vi "fly dominator105.vi"() -> ()   [LabVIEW 2021]
uses:
  states.ctl
  <vilib>/Analysis/NI_AALBase.lvlib
  <vilib>/Analysis/baseanly.llb/Mean (DBL).vi
  <extravilib>/ChannelInstances/Tag-bool.lvlib
  <vilib>/DAQmx/write.llb/DAQmx Write (Digital Bool 1Line 1Point).vi
  <vilib>/DAQmx/create/channels.llb/DAQmx Create Channel (DO-Digital Output).vi
  <resource>/objmgr/daqmx.rc
  <extravilib>/ChannelInstances/Tag-dbl.lvlib
  <vilib>/Waveform/WDTFileIO.llb/ Write Waveform to File.vi
  C:/Users/IMAGINGPC-3/Desktop/software/4c wheel/Thorlabs.MotionControl.Controls.dll
  software/4c wheel/Thorlabs.MotionControl.Controls.dll
  C:/Users/IMAGINGPC-3/Desktop/software/4c wheel/Thorlabs.MotionControl.Benchtop.StepperMotorCLI.dll
  software/4c wheel/Thorlabs.MotionControl.Benchtop.StepperMotorCLI.dll
  <vilib>/Analysis/NI_AALPro.lvlib
  0273469b-1630-426e-8888-91f9d245564e.vi
  8ea25fb4-7a89-4be8-837a-9bc05b844755.vi
  <vilib>/smtpClient/LabVIEWSMTPClient.lvlib
  a9b58a78-20d6-47fd-9184-b30837673e93.vi
  <vilib>/smtpClient/Set Message Text.vi
  <vilib>/DAQmx/create/channels.llb/DAQmx Create Channel (AI-Voltage-Basic).vi
  <vilib>/DAQmx/configure/timing.llb/DAQmx Timing (Sample Clock).vi
  <vilib>/DAQmx/read.llb/DAQmx Read (Analog 1D DBL 1Chan NSamp).vi
  <vilib>/DAQmx/read.llb/DAQmx Read (Digital Bool 1Line 1Point).vi
  <vilib>/DAQmx/create/channels.llb/DAQmx Create Channel (DI-Digital Input).vi
  <vilib>/Instr/_visa.llb/VISA Configure Serial Port (Instr).vi
panel:
  in  "fast scan setting":enum32{"4000", "2000"}(tab)
  out "Last saved file 4000":path
  in  "Save base file name 4000":path=path "\\\\157.82.9.50\\d/20240220/gp mor/tm6b/4000/uasmcherry.tm6b.2.50w.4000"
  out "Last saved file number 4000":i32
  out "Last saved file 2000":path
  in  "Save base file name 2000":path=path "\\\\FINDSCTRL\\findsdata/finds2/20240321/2000test"
  out "Last saved file number 2000":i32
  in  "genotypic screening":enum32{"general ", "morphology", "intensity"}(tab)
  in  "screening method":T1(ring)=enum."Pix count"
  out "mean":dbl format="%0.2f"
  out "screening time":dbl
  in  "Enable screening\n(during flow zoometry)":bool
  in  "go to 2000?":bool=TRUE
  in  "go to 4000?":bool
  in  "GS speed 3":bool
  in  "calibration?":bool
  in  "GS speed 2":bool
  in  "morphology\nthreshold 1":i32=40
  out "morphology \nscreening time":dbl
  in  "morphology\nthreshold 2":dbl=110.0
  in  "max intensity\n threshold":i32=3500
  out "larva size":bool
  out "triggered?":bool
  out "Numeric 7":i32
  out "Numeric 6":i32
  out "Numeric 5":dbl
  out "waiting number":i32
  out "larvae in chamber?":bool
  in  "batch#":string="3"
  in  "High speed?":bool
  out "x-y 2":i32
  out "RAL r2":i32
  in  "clearing date":string="20240224"
  in  "genotype":T2(ring)
  in  "laser channel":string="594-655"
  in  "wait for\nclearing":bool
  in  "wait for clearing? 2":bool
  out "clear finished?":bool
  out "relative seconds 2":dbl format="%_19f"
  in  "real laser power":string="10.5_19mw"
  in  "Operator":enum16{"kobayashi", "hanqing WANG", "chenglang"}(ring)=enum."hanqing WANG"
  out "screening":bool
  out "experiment time(mins)":dbl
  out "experiment stop time (relative)":dbl format="%_19f"
  out "experiment start time (relative)":dbl format="%_19f"
  out "at imaging time":dbl[](graph)
  in  "SerialNumber":string="40227394"
  in  "High Speed 2":u32=10000
  in  "correction":i32=-200
  out "OK Done":bool
  in  "Main/Sub":bool
  in  "Acceleration Time":u16
  in  "Low Speed":u32=100 min=1 max=500000
  in  "Save start #":i32
  out "Last saved file number 4":i32
  in  "sample name":string="exp"
  in  "Acquire speed 3 (um/s)":u32=2000
  in  "Samples to measure 3":i32=100
  out "Mean intensity\nof frame":dbl format="%0.2f"
  in  "wave trigger":dbl
  in  "Acquire speed 2 (um/s)":u32=4000
  in  "Samples to measure 2":i32=100
  in  "file (boundary finding) 3":path=path "D:/data/garbage data/as"
  in  "file ( time) 2":path=path "D:/data/garbage data/sssa"
  in  "Go to edge pulses":u32=500
  in  "Go to edge speed":u32=4000
  in  "um to move":u32=6000
  in  "488":bool
  in  "532":bool
  in  "594":bool
  in  "405":bool
  in  "# to measure":i32=200
  out "Last saved #":i32
  out "Last saved file":path
  out "Current state":string
  in  "Acquire speed (um/s)":u32=200
  in  "Movement direction":bool=TRUE
  out "Saving image":bool
  out "Moving":bool
  in  "Save directory":path=path "\\\\FINDSCTRL\\findsdata/finds2/20240401"
  in  "Mean trigger":i32=150
  out "Sub img mean":dbl
  out "Sub image":u16[][](graph) caption="Image"
  in  "XS x length":i32=1000
  in  "XS x px start":i32=500
  out "READY":bool
  in  "Shut down":bool
  out "Streaming":bool
  in  "XS y length":i32=1000
  in  "XS y px start":i32=1000
  out "Camera error out":errorcluster {"code" format="%.0x"}
  out "Obtained image":u16[][](graph) caption="Image"
  out "Frame count":i32
  in  "Frames in memory":i32=1500
  in  "tube to stop":i32=6
  in  "maximum":i32=15
  in  "594?":bool
  in  "488?":bool
  in  "532?":bool
  in  "405?":bool
  in  "shower time":u32=20000
  in  "waiting time for\n robotic arm":u32=12000
  in  "washing time":u32=11000
  in  "Range 2":bool
  out "4c label #":i32
  out "max value":i32
  out "R2":i32
  out "real R2":i32
  out "R1":i32
  in  "manual loading":bool
  in  "shower time(ms)":u32=5000
  in  "BUBBLE SIZE":i32=3
  out "gp":dbl
  in  "um to move short":u32=6500
  in  "um to move long":u32=7000
  out "OK Done 4":bool
  out "homing speed":bool
  out "homing":bool
  in  "4c direction":bool=TRUE
  in  "manual 4c":bool
  out "tube changing #":i32
  in  "# BEFORE GO DOWN":i32=1
  in  "TIME THRESHOLD":dbl=40.0
  in  "force anticlogging":bool
  in  "Flow Rate (5.00)":dbl=100.0 format="%#.4f"
  in  "milliseconds to wait":u32=4000
  in  "position":dbl=0.083333
  out "#of edgehunting":u32
  in  "wavelength":string
  in  "4c Base file name":string="brp_each"
  out "594 i":bool
  out "532 i":bool
  out "488 i":bool
  out "405 i":bool
  out "Last saved file 4c":path
  in  "BenchtopStepperControl":refnum<k24>(container)
  in  "4C":bool
  in  "Frames in memory 2":i32=800
  out "larva size in frame":i32
  out "backwards pulses":i32
  in  "scanning Speed":u32=20000 min=1 max=500000
  out "larvae size in scan":dbl[](graph)
  in  "Direction 2":bool
  in  "scanning distance (um)":u32=43000 min=1 max=500000
  in  "manual edgehunting":bool
  in  "Number of samples":i32=150
  out "Waveform Graph":dbl[](graph)
  out "loading tube#":i32
  in  "manual load":bool
  in  "Force move":bool
  in  "Larva # to move":i32=1000
  out "Larvae until move":i32
  in  "tb Pulses to move":u32=750 min=1 max=500000
  in  "tube Direction":bool
  in  "force reverse":bool
  in  "reverse flow \nthreshold (sec)":dbl=90.0
  out "Elapsed (sec)":dbl
  in  "next loop":bool=TRUE
  out "False triggers":i32
  in  "Wait v2":u32=100
  in  "Wait v1":u32=40
  in  "Return move":u32=1700
  in  "manual imaging":bool
  in  "SampClk.Rate 2":dbl=100000.0
  in  "Physical Channel 2":tag="Dev1/ai0"
  in  "First move":u32=3000
  in  "Abort 2":bool
  in  "Stop Trigger stream":bool
  out "Mean":dbl format="%0.2f"
  out "Triggered":bool
  in  "Trigger":dbl=0.10000000000000009
  out "Trigger PD running mean":dbl(graph)
  out "#triggers":i32
  in  "START AUTO IMAGING":bool caption="Start\nauto imaging"
  in  "Continuous\nacquisition":bool
  in  "START":bool
  in  "Quit":bool
  # "NOTICE:\nplease check the state frequently\nyou have to go back to chilling state before you do any other operation"
  # "File & save settings"
  # "motion tracker"
  # "Status"
  # "Laser output\n(Chilling state updates)"
  # "Camera streaming"
  # "Acquisition settings"
  # "Edgehunting settings"
  # "B"
  # "F"
  # "Flow zoometry"
  # "Trigger"
  # "No-flow imaging"
  # "error trigger exclusion setting"
  # "Manual image acquisition\n(initiate from chilling state)"
  # "Find boundary settings"
  # "Sucking tube settings"
  # "Abort bd finding"
  # "down"
  # "up"
  # "Anti-clogging settings"
  # "ROBOTIC ARM LOADING"
  # "channel selection"
types:
  T1 = enum16{"morphology", "Pix count", "MAX INTENSITY", "Average int"}
  T2 = enum16{"others", "ptc>mcherry_4hit", "ptc>mcherry_noncancer", "TB", "nonTB", "63148"}
  T3 = enum32{"Invalid", "Standard", "Closed", "Hidden", "Minimized", "Maximized"}
  T4 = typedef "states.ctl" = enum16{"manual_imaging", "initialize_2", "4c?", "Initialize", "Chilling", "4climbo", "light reverse", "wait for clearing", "manual loading", "4cini", "reverse", "2000", "4000", "screening", "tube position", "Edgehunting", "Edgehunting2", "homing", "gp", "antic\n", "Stream w/o flow2", "Stream w/o flow", "stopflow triggertest", "Find boundaries", "Acquire", "save", "auto imaging", "robotic arm", "Close", "594", "532", "488", "405", "4c acquirement", "Stop"}
  T5 = enum32{"Map Pixel Pointer", "Unmap Pixel Pointer", "Get Pixels Infos"}
  T6 = cluster{"Output Trigger Period":dbl, "Delay":dbl, "Source":u32}
  T7 = cluster{"Output Trigger Mode":u32, "Output Trigger Polarity":u32}
  T8 = typedef "Image Type" = u32
  T9 = typedef "IMAQ Image.ctl" = refnum<image>
  T10 = typedef "Tag-bool.lvlib/))Channel.ctl" = refnum<queue>
  T11 = typedef "Tag-dbl.lvlib/))Channel.ctl" = refnum<queue>
  T12 = typedef "LabVIEWSMTPClient.lvlib/SmtpClientHandle.ctl" = refnum<k1>
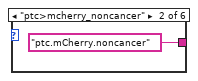
[diagram p2: hidden frame]
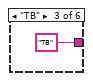
[diagram p3: hidden frame]
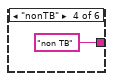
[diagram p4: hidden frame]
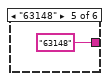
[diagram p5: hidden frame]
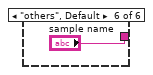
[diagram p6: hidden frame]
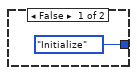
[diagram p9: hidden frame]
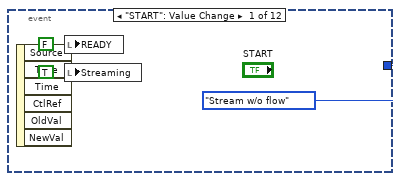
[diagram p13: hidden frame]
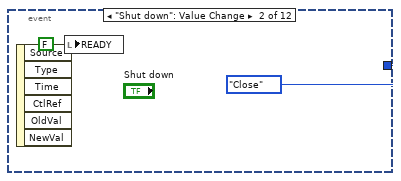
[diagram p14: hidden frame]
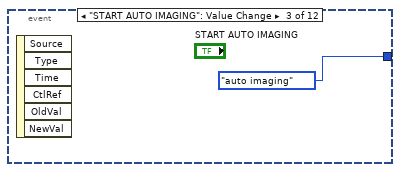
[diagram p15: hidden frame]
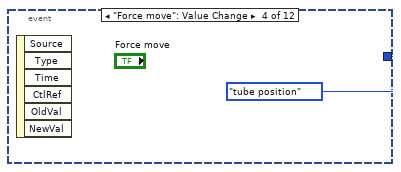
[diagram p16: hidden frame]
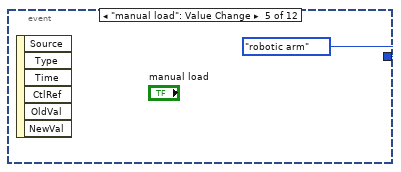
[diagram p17: hidden frame]
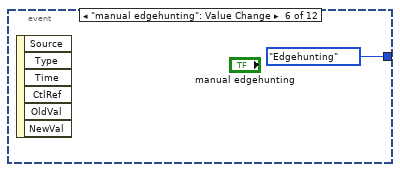
[diagram p18: hidden frame]
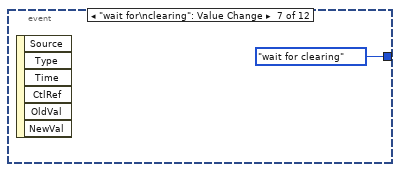
[diagram p19: hidden frame]
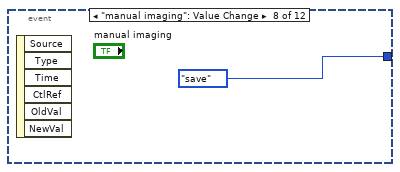
[diagram p20: hidden frame]
diagram:
  w14 = 0  # 4c counter
  # "screening time record"
  # "unused yet"
  # "4c counter"
  # "stage"
  # "HD pump"
  # "command"
  # "stop"
  # "r1"
  # "R2"
  # "R1"
  # "TF"
  # "Is this VISA wired?"
  # "200"
  # "500"
  # "false trigger SR"
  # "laser"
  # "camera"
  # "kimitsu\npw"
  # "laser detector  RF"
  # "HD pump"
  # "IMAQ image SR"
  # "Larva size SR"
  # "Stage SR"
  # "Pinch valve engage to flow"
  # "State shift register"
  # "Pump shift registers"
  n1 = Open VI Reference(vi path=path "C:/FINDS_VIs/Abyss-watcher_love-edition.vi") -> (vi reference=w12:refnum<vi>)  [unwired: 5 in, 1 out]
  n2 = call "PortInit.vi"("VISAリソース名"=refnum<visa-resource-name> "COM11") -> ("VISA resource name out"=w2:refnum<visa-resource-name>)
  n3 = Initialize Array(0.0 ("element"), 1000 ("dimension size")) -> (w64:dbl[])
  n4 = Initialize Array(i16 0 ("element"), 1000 ("dimension size")) -> (w42:i16[])
  n5 = invoke class="VI" method="FP.Open"(reference=w12, "State"=T3."Hidden") -> (reference out=w10:refnum<vi>)  [unwired: 3 in, 4 out]
  n6 = call-poly <vilib>:"DAQmx Create Virtual Channel.vi"("lines"=tag "Dev1/port0/line2") -> ("task out"=w68:refnum<k21>, "error out"=w77:errorcluster)  [unwired: 13 in]
  n7 = call <vilib>:"DAQmx Start Task.vi"("task/channels in"=w68, "error in"=w77) -> ("task out"=w69:refnum<k21>, "error out"=w47:errorcluster)  [unwired: 12 in]
  n8 = Initialize Array(0.0 ("element"), 200 ("dimension size")) -> (w60:dbl[])
  n9 = Initialize Array(i16 0 ("element"), 1000 ("dimension size")) -> (w53:i16[])
  n10 = invoke class="VI" method="Run VI"(reference=w10, "Wait until done"=FALSE ("Wait Until Done"), "Auto Dispose Ref"=TRUE ("Auto Dispose Reference")) -> (reference out=w4:refnum<vi>)  [unwired: 2 in, 4 out]
  n11 = call-poly <vilib>:"DAQmx Create Virtual Channel.vi"("lines"=tag "Dev1/port0/line3") -> ("task out"=w71:refnum<k21>, "error out"=w75:errorcluster)  [unwired: 13 in]
  n12 = call-poly <vilib>:"DAQmx Create Virtual Channel.vi"("lines"=tag "Dev1/port0/line1") -> ("task out"=w80:refnum<k21>, "error out"=w73:errorcluster)  [unwired: 13 in]
  n13 = call <vilib>:"DAQmx Start Task.vi"("task/channels in"=w71, "error in"=w75) -> ("task out"=w70:refnum<k21>, "error out"=w46:errorcluster)  [unwired: 12 in]
  n14 = call-poly <vilib>:"DAQmx Create Virtual Channel.vi"("lines"=tag "Dev1/port1/line2") -> ("task out"=w25:refnum<k21>, "error out"=w23:errorcluster)  [unwired: 13 in]
  n15 = call-poly <vilib>:"DAQmx Create Virtual Channel.vi"("lines"=tag "Dev1/port0/line0") -> ("task out"=w84:refnum<k21>, "error out"=w83:errorcluster)  [unwired: 13 in]
  n16 = Initialize Array(0.0 ("element"), 200 ("dimension size")) -> (w17:dbl[])
  n17 = call <vilib>:"DAQmx Start Task.vi"("task/channels in"=w84, "error in"=w83) -> ("task out"=w81:refnum<k21>, "error out"=w67:errorcluster)  [unwired: 12 in]
  n18 = call <vilib>:"DAQmx Start Task.vi"("task/channels in"=w80, "error in"=w73) -> ("task out"=w78:refnum<k21>, "error out"=w72:errorcluster)  [unwired: 12 in]
  n19 = Create Network Stream Reader Endpoint(7:1 ("reader buffer size"), 9:cluster{dbl, bool} {0.0, TRUE}, 11:"reader" ("reader name")) -> (3:w5:refnum<k21>)  [unwired: 4 in, 1 out]
  n20 = Initialize Array(0.0 ("element"), 200 ("dimension size")) -> (w27:dbl[])
  n21 = Initialize Array("", 1000 ("dimension size")) -> (w57:string[])
  n22 = Initialize Array(i16 0 ("element"), 1000 ("dimension size")) -> (w51:i16[])
  n23 = call <vilib>:"High Resolution Relative Seconds.vi"() -> ("relative seconds"=w31:dbl)
  n24 = call <vilib>:"DAQmx Start Task.vi"("task/channels in"=w25, "error in"=w23) -> ("task out"=w22:refnum<k21>)  [unwired: 12 in, 1 out]
  n25 = while {
    shift-right: [w211] -> _
    shift-left: states."Stream w/o flow2" -> [w225]
    shift-right: [w222] -> _
    shift-left: _ -> [w220]
    shift-right: [w221] -> _
    shift-left: _ -> [w219]
    shift-right: [w217] -> _
    shift-left: "Save start #" -> [w218]
    shift-right: [w216] -> _
    shift-left: _ -> [w215]
    shift-right: [w115] -> w15
    shift-left: _ -> [w214]
    shift-right: [w213] -> _
    shift-left: _ -> [w212]
    shift-right: [w209] -> w66
    shift-left: _ -> [w208]
    tunnel: w81 -> [w126]
    tunnel: w78 -> [w207]
    tunnel: w72 -> [w206]
    tunnel: w70 -> [w204]
    tunnel: w69 -> [w205]
    tunnel: [w126] -> w33
    tunnel: [w125] -> w32
    tunnel: w67 -> [w125]
    shift-right: [w202] -> _
    shift-left: 0 -> [w203]
    shift-right: [w166] -> w45
    shift-left: w64 -> [w201]
    shift-right: [w130] -> _
    shift-left: w60 -> [w200]
    shift-right: [w191] -> _
    shift-left: w57 -> [w193]
    shift-right: [w187] -> _
    shift-left: 0 -> [w188]
    tunnel: ["file ( time) 2"] -> _
    shift-right: [w180] -> _
    shift-left: i32[] [] -> [w181]
    shift-right: [w88] -> w49
    shift-left: w53 -> [w179]
    tunnel: [w160] -> w50
    shift-right: [w165] -> w34
    shift-left: _ -> [w177]
    shift-right: [w175] -> _
    shift-left: 1 -> [w176]
    shift-right: [w173] -> w48
    shift-left: w51 -> [w174]
    tunnel: w47 -> [w170]
    tunnel: w46 -> [w169]
    shift-right: [w167] -> w41
    shift-left: w42 -> [w168]
    shift-right: [w163] -> _
    shift-left: 1 -> [w164]
    shift-right: [w159] -> _
    shift-left: _ -> [w158]
    shift-right: [w156] -> _
    shift-left: 0 -> [w157]
    shift-right: [w155] -> _
    shift-left: u32 0 ("millisecond timer value") -> [w154]
    tunnel: [w153] -> _ mode=indexing
    shift-right: [w151] -> _
    shift-left: 0 -> [w152]
    shift-right: [w141] -> _
    shift-left: _ -> [w138]
    shift-right: [w140] -> _
    shift-left: _ -> [w136]
    shift-right: [w139] -> _
    shift-left: _ -> [w137]
    shift-right: [w135] -> _
    shift-left: _ -> [w133]
    shift-right: [w134] -> _
    shift-left: _ -> [w94]
    tunnel: w31 -> [w132]
    shift-right: [w129] -> _
    shift-left: w27 -> [w131]
    shift-right: [w127] -> _
    shift-left: u32 0 ("millisecond timer value") -> [w128]
    tunnel: w22 -> [w124]
    tunnel: [w123] -> _
    shift-right: [w121] -> _
    shift-left: 0 -> [w122]
    shift-right: [w119] -> _
    shift-left: 0 -> [w120]
    tunnel: w2 -> [w118]
    shift-right: [w116] -> _
    shift-left: w17 -> [w117]
    shift-right: [w98] -> _
    shift-left: w14 -> [w99]
    shift-right: [w95] -> _
    shift-left: w5 -> [w96]
    tunnel: w4 -> [w93]
    shift-right: [w91] -> _
    shift-left: 0 -> [w92]
    shift-right: [w90] -> _
    shift-left: _ -> [w89]
    stop <- w224 stop-if-true
    (unwired) TRUE ("replace all? (F)")
    w111 = "_" ("string")
    # "loading tube#"
    # "larva until move"
    # "robotic arm"
    # "valve"
    # "405"
    # "r1"
    # "r2"
    # "stage"
    # "camera"
    # "camera"
    # "camera"
    n26 = Get Date/Time In Seconds() -> (seconds since 1Jan1904=w105:timestamp)
    n27 = Path To String(path="Save directory") -> (string=w145:string)
    n28 = Concatenate Strings(w145, "\\raw") -> (w143:string)
    n29 = case shown="\"ptc>mcherry_4hit\"" "genotype" {
      tunnel: ["ptc.mCherry.4hit" ("sample name") "ptc.mCherry.noncancer" ("sample name") "TB" ("sample name") "non TB" ("sample name") "63148" ("sample name") "sample name"] -> w109
      frame "ptc>mcherry_4hit" {
      }
      frame "ptc>mcherry_noncancer" {
      }
      frame "TB" {
      }
      frame "nonTB" {
      }
      frame "63148" {
      }
      frame "others", Default {
      }
    }
    n30 = String To Path(string=w143) -> (path=w142:path)
    n31 = Get Date/Time String(date format (0)=enum16{"short", "long", "abbreviated"}."long", seconds (now)=w105) -> (time string=w192:string)  [unwired: 1 in, 1 out]
    n32 = Format Date/Time String(time format string (%c)="%Y", seconds (now)=w105) -> (date/time string=w108:string)  [unwired: 1 in]
    n33 = Format Date/Time String(time format string (%c)="%m", seconds (now)=w105) -> (date/time string=w107:string)  [unwired: 1 in]
    n34 = Format Date/Time String(time format string (%c)="%d", seconds (now)=w105) -> (date/time string=w106:string)  [unwired: 1 in]
    n35 = Concatenate Strings(w145, "\\temp") -> (w147:string)
    n36 = String To Path(string=w147) -> (path=w146:path)
    n37 = call <vilib>:"Check if File or Folder Exists.vi"("path"=w146) -> ("file or folder exists?"=w150:bool)  [unwired: 8 in, 2 out]
    n38 = case shown="False" w150 {
      tunnel: w146 -> [w233 _]
      tunnel: w142 -> [w232 _]
      frame False {
        n39 = Create Folder(path (use dialog)=w232) -> ()  [unwired: 2 in, 3 out]
        n40 = Create Folder(path (use dialog)=w233) -> ()  [unwired: 2 in, 3 out]
      }
      frame True {
      }
    }
    n41 = Concatenate Strings(w108, w107, w106) -> (w97:string)
    n42 = Concatenate Strings(w97, w111, w109, w111, "laser channel", "B" ("string"), "batch#") -> (w114:string)
    n43 = Path To String(path="Save directory") -> (string=w162:string)
    n44 = Search and Replace String(input string=w192, search string="PM", replace string="" ("replace string (\"\")")) -> (result string=w197:string)  [unwired: 5 in, 3 out]
    n45 = Search and Replace String(input string=w197, search string="am", replace string="" ("replace string (\"\")")) -> (result string=w185:string)  [unwired: 5 in, 3 out]
    n46 = Search and Replace String(input string=w185, search string=":", replace string=" " ("replace string (\"\")")) -> (result string=w171:string)  [unwired: 5 in, 3 out]
    n47 = Path To String(path="file (boundary finding) 3") -> ()  [unwired: 1 out]
    n48 = Concatenate Strings(w97, " " ("string")) -> (w190:string)
    n49 = Concatenate Strings(w162, w114) -> (w161:string)
    n50 = Equal?(x=w225, y=states."Stop") -> (x = y?=w224:bool)
    n51 = String To Path(string=w161) -> (path=w160:path)
    n52 = Concatenate Strings(w190, w185) -> (w186:string)
    n53 = case shown="\"manual_imaging\"" w225 {
      tunnel: [w271 w343 w530 w703 w767 w815 w903 w1242 w1443 w1757 w1881 w2119 w2410 w2516 w2754 w2926 w3076 w3239 w3451 w3648 w3705 w3763 w3818 w3875 w3936 w3971 w4182 w4331 w4583 u32 0 ("Handle out") u32 0 ("Handle out")] -> w222
      tunnel: [w270 w346 w533 w702 w766 w816 w905 w1241 w1442 w1756 w1880 w2118 w2409 w2517 w2752 w2925 w3075 w3237 w3449 w3647 w3704 w3762 w3817 w3874 w3935 w3970 w4181 w4330 w4582 errorcluster {"status"=FALSE, "code"=0, "source"=""} ("error out") errorcluster {"status"=FALSE, "code"=0, "source"=""} ("error out")] -> w221
      tunnel: [w247 states."Chilling" states."Chilling" w649 w735 states."Chilling" w906 w1225 w1423 w1729 w1853 w2054 w2338 w2524 w2760 w2895 w3077 w3276 w3483 w3613 w3670 w3729 w3783 w3840 w3884 w4007 w4189 w4296 w4590 states."Stop" states."Stop"] -> w211
      tunnel: w220 -> [w271 _ _ w703 w767 w812 w903 w1242 w1443 w1757 w1881 w2119 w2410 w2528 w2753 w2926 w3076 w3288 w3494 w3648 w3705 w3763 w3818 w3875 w3936 w4018 w4202 w4331 w4603 w4787 _]
      tunnel: w219 -> [w270 _ _ w702 w766 w813 w905 w1241 w1442 w1756 w1880 w2118 w2409 w2526 w2751 w2925 w3075 w3289 w3495 w3647 w3704 w3762 w3817 w3874 w3935 w4019 w4203 w4330 w4604 w4786 _]
      tunnel: w218 -> [w269 w355 w547 w699 w765 w820 w907 w1240 w1441 w1755 w1879 w2117 w2408 w2515 w2774 w2924 w3074 w3217 w3418 w3646 w3703 w3761 w3816 w3873 w3934 w3958 w4140 w4329 w4539 w4782 w4924]
      tunnel: [w269 w355 w547 w699 w765 w820 w907 w1240 w1441 w1755 w1879 w2117 w2408 w2515 w2774 w2924 w3074 w3249 w3460 w3646 w3703 w3761 w3816 w3873 w3934 w3957 w4140 w4329 w4539 w4782 w4924] -> w217
      tunnel: [_ _ _ w696 _ w819 _ _ _ _ _ _ _ _ _ _ _ w3287 w3493 _ _ _ _ _ _ w4017 w4201 _ w4602 refnum<visa-resource-name> refnum ("VISA resource name out") refnum<visa-resource-name> refnum ("VISA resource name out")] -> w216
      tunnel: w215 -> [_ _ _ w696 _ w819 _ _ _ _ _ _ _ _ _ _ _ w3287 w3493 _ _ _ _ _ _ w4017 w4201 _ w4602 _ _]
      tunnel: [w268 w276 w482 w671 w764 w818 w904 w1239 w1422 w1754 w1878 w2116 w2407 w2507 w2741 w2905 w3040 w3271 w3480 w3645 w3702 w3760 w3815 w3872 w3933 w4004 w4184 w4328 w4585 w4780 w4922] -> w115
      tunnel: w214 -> [w268 _ _ w671 w764 w818 w904 w1239 w1422 w1754 w1878 w2116 w2407 w2507 w2759 w2907 w3040 w3286 w3492 w3645 w3702 w3760 w3815 w3872 w3933 w4016 w4200 w4328 w4601 w4780 w4922]
      tunnel: [w267 w335 w522 u32 0 w763 w807 w897 w1238 w1386 w1753 w1877 w2115 w2406 w2518 w2773 w2923 w3079 w3255 w3466 w3644 w3701 w3759 w3814 w3871 w3932 w3989 w4167 w4327 w4518 w4775 w4917] -> w213
      tunnel: w212 -> [w267 w335 w522 _ w763 w807 w897 w1238 w1386 w1753 w1877 w2115 w2406 _ w2773 w2923 w3079 w3255 w3466 w3644 w3701 w3759 w3814 w3871 w3932 w3989 w4167 w4327 w4518 w4775 w4917]
      tunnel: "Save directory" -> [_ _ _ _ _ _ _ _ _ _ _ _ _ _ _ _ _ w3279 w3485 _ _ _ _ _ _ w4009 _ _ _ _ _]
      tunnel: [w266 w340 w527 w694 w762 w811 w901 w1237 w1440 w1752 w1876 w2114 w2405 w2510 w2745 w2922 w3081 w3267 w3477 w3643 w3700 w3758 w3813 w3870 w3931 w4001 w4179 w4326 w4580 w4779 w4921] -> w209
      tunnel: w208 -> [w266 _ _ w694 w762 w814 w901 w1237 w1440 w1752 w1876 w2114 w2405 w2539 w2750 w2922 w3081 w3267 w3477 w3643 w3700 w3758 w3813 w3870 w3931 w4001 w4179 w4326 w4580 w4779 w4921]
      tunnel: w207 -> [_ _ _ w693 _ _ _ _ _ _ _ _ _ _ _ _ _ _ _ w3619 w3676 w3735 w3789 w3846 _ _ _ _ _ w4765 w4909]
      tunnel: w206 -> [_ _ _ w692 _ _ _ _ _ _ _ _ _ _ _ _ _ _ _ _ _ _ _ _ _ _ _ _ _ _ w4908]
      tunnel: w205 -> [_ _ _ w691 _ _ _ _ _ _ _ _ _ _ _ _ _ _ _ w3618 w3675 w3734 w3788 w3845 _ _ _ _ _ w4766 w4907]
      tunnel: w204 -> [_ _ _ w690 _ _ _ _ _ _ _ _ _ _ _ _ _ _ _ w3617 w3674 w3733 w3787 w3844 _ _ _ _ _ w4764 w4906]
      tunnel: w203 -> [w265 w338 w525 w686 w761 w810 w900 w1236 w1439 w1751 w1875 w2113 w2404 _ w2772 w2921 w3073 w3253 w3464 w3642 w3699 w3757 w3812 w3869 w3930 w3987 w4165 w4325 w4567 w4778 w4920]
      tunnel: [w265 w338 w525 w686 w761 w810 w900 w1236 w1439 w1751 w1875 w2113 w2404 0 w2772 w2921 w3072 w3253 w3464 w3642 w3699 w3757 w3812 w3869 w3930 w3987 w4165 w4325 w4567 w4778 w4920] -> w202
      tunnel: [w264 w337 w524 w685 w760 w809 w899 w1235 w1438 w1750 w1874 w2112 w2403 w2494 w2771 w2920 w3071 w3230 w3442 w3641 w3698 w3756 w3811 w3868 w3929 w3976 w4122 w4324 w4537 w4777 w4919] -> w166
      tunnel: w201 -> [w264 w337 w524 w685 w760 w809 w899 w1235 w1438 w1750 w1874 w2112 w2403 w2494 w2771 w2920 w3071 w3230 w3442 w3641 w3698 w3756 w3811 w3868 w3929 w3976 w4124 w4324 w4537 w4777 w4919]
      tunnel: w200 -> [w263 w336 w523 w684 w759 w808 w898 w1234 w1437 w1749 w1873 w2111 w2402 w2493 w2728 w2919 w3070 w3229 w3441 w3640 w3697 w3755 w3810 w3867 w3928 w3975 w4129 w4323 w4565 w4776 w4918]
      tunnel: [w263 w336 w523 w684 w759 w808 w898 w1234 w1437 w1749 w1873 w2111 w2402 w2493 w2727 w2919 w3070 w3229 w3441 w3640 w3697 w3755 w3810 w3867 w3928 w3975 w4129 w4323 w4564 w4776 w4918] -> w130
      tunnel: w186 -> [_ _ _ _ _ _ _ _ _ _ _ _ _ _ _ _ _ _ _ _ _ _ _ _ _ _ _ _ _ _ _]
      tunnel: w193 -> [w262 w334 w521 w683 w758 w806 w894 w1233 w1388 w1748 w1872 w2110 w2401 w2492 w2770 w2918 w3069 w3252 w3463 w3639 w3696 w3754 w3809 w3866 w3927 w3986 w4158 w4322 w4556 w4774 w4916]
      tunnel: w171 -> [_ _ _ _ _ _ _ _ _ _ _ _ _ _ _ _ _ w3251 w3462 _ _ _ _ _ _ w3985 w4163 _ w4562 _ _]
      tunnel: [w262 w334 w521 w683 w758 w806 w894 w1233 w1388 w1748 w1872 w2110 w2401 w2492 w2770 w2918 w3069 w3250 w3461 w3639 w3696 w3754 w3809 w3866 w3927 w3984 w4158 w4322 w4556 w4774 w4916] -> w191
      tunnel: w188 -> [w261 w333 w520 w682 w757 w805 w893 w1232 w1387 w1747 w1871 w2109 w2400 w2491 w2769 w2917 w3068 _ _ w3638 w3695 w3753 w3808 w3865 w3926 w3964 _ w4321 _ w4773 w4915]
      tunnel: [w261 w333 w520 w682 w757 w805 w893 w1232 w1379 w1747 w1871 w2109 w2400 w2491 w2769 w2917 w3068 0 0 w3638 w3695 w3753 w3808 w3865 w3926 w3964 0 w4321 0 w4773 w4915] -> w187
      tunnel: w181 -> [w260 w332 w519 w681 w756 w804 w892 w1231 w1382 w1746 w1870 w2108 w2399 w2480 w2768 w2916 w3067 w3248 w3459 w3637 w3694 w3752 w3807 w3864 w3925 w3983 w4162 w4320 w4561 w4772 w4914]
      tunnel: [w260 w332 w519 w681 w756 w804 w892 w1231 w1382 w1746 w1870 w2108 w2399 w2479 w2768 w2916 w3067 w3248 w3459 w3637 w3694 w3752 w3807 w3864 w3925 w3983 w4162 w4320 w4561 w4772 w4914] -> w180
      tunnel: w179 -> [w259 w331 w518 w680 w755 w803 w891 w1230 w1381 w1745 w1869 w2107 w2398 w2489 w2711 w2915 w3066 _ _ w3636 w3693 w3751 w3806 w3863 w3924 _ w4159 w4319 w4557 w4771 w4913]
      tunnel: [w259 w331 w518 w680 w755 w803 w891 w1230 w1381 w1745 w1869 w2107 w2398 w2489 w2711 w2915 w3066 i16[] [] i16[] [] w3636 w3693 w3751 w3806 w3863 w3924 w3965 w4159 w4319 w4557 w4771 w4913] -> w88
      tunnel: "Save base file name 4000" -> [_ _ _ _ _ _ _ _ _ _ _ _ _ _ _ _ _ _ _ _ _ _ _ _ _ _ w4160 _ _ _ _]
      tunnel: [w258 w330 w517 w679 w754 w802 w890 w1229 w1380 w1744 w1868 w2106 w2397 w2488 w2767 w2914 w3065 w3247 w3458 w3635 w3692 w3750 w3805 w3862 w3923 w3982 w4131 w4318 w4558 w4770 w4912] -> w165
      tunnel: w177 -> [w258 w330 w517 w679 w754 w802 w890 w1229 w1380 w1744 w1868 w2106 w2397 w2488 w2767 w2914 w3065 w3247 w3458 w3635 w3692 w3750 w3805 w3862 w3923 w3982 w4131 w4318 _ w4770 w4912]
      tunnel: w176 -> [w257 w329 w516 w678 w753 w801 w889 w1209 w1378 w1743 w1867 w2105 w2396 w2487 w2766 w2913 w3064 w3246 w3457 w3634 w3691 w3749 w3804 w3861 w3922 w3981 w4141 w4317 w4526 w4763 w4911]
      tunnel: [w257 w329 w516 w678 w753 w801 w889 w1209 w1378 w1743 w1867 w2105 w2396 w2487 w2766 w2913 w3064 w3246 w3457 w3634 w3691 w3749 w3804 w3861 w3922 w3981 w4125 w4317 w4526 w4763 w4911] -> w175
      tunnel: w174 -> [w256 w328 w515 w677 w752 w800 w888 w1228 w1377 w1742 w1866 w2104 w2395 w2486 w2765 w2904 w3063 w3245 w3456 w3633 w3690 w3748 w3803 w3860 w3921 w3965 w4139 w4316 w4533 w4762 w4910]
      tunnel: [w256 w328 w515 w677 w752 w800 w888 w1228 w1377 w1742 w1866 w2104 w2395 w2486 w2765 w2904 w3063 w3245 w3456 w3633 w3690 w3748 w3803 w3860 w3921 w3965 w4138 w4316 w4533 w4762 w4910] -> w173
      tunnel: w170 -> [_ _ _ _ _ _ _ _ _ _ _ _ _ _ _ _ _ _ _ _ _ _ _ _ _ _ _ _ _ _ w4895]
      tunnel: w169 -> [_ _ _ _ _ _ _ _ _ _ _ _ _ _ _ _ _ _ _ _ _ _ _ _ _ _ _ _ _ _ w4892]
      tunnel: [w255 w327 w514 w676 w751 w799 w887 w1227 w1376 w1741 w1865 w2103 w2394 w2485 w2764 w2912 w3062 w3244 w3455 w3632 w3689 w3747 w3802 w3859 w3920 w3980 w4132 w4315 w4535 w4761 w4890] -> w167
      tunnel: w168 -> [w255 w327 w514 w676 w751 w799 w887 w1227 w1376 w1741 w1865 w2103 w2394 w2485 w2764 w2912 w3062 w3244 w3455 w3632 w3689 w3747 w3802 w3859 w3920 w3980 w4132 w4315 w4534 w4761 w4890]
      tunnel: w164 -> [w254 w326 w513 w675 w750 w798 w886 w1226 w1375 w1740 w1864 w2102 w2393 w2484 w2763 w2911 w3028 w3243 w3454 w3631 w3688 w3746 w3801 w3858 w3919 w3979 w4130 w4314 w4506 w4760 w4889]
      tunnel: [w254 w326 w513 w675 w750 w798 w886 w1226 w1375 w1740 w1864 w2102 w2393 w2484 w2763 w2911 w3028 w3243 w3454 w3631 w3688 w3746 w3801 w3858 w3919 w3979 w4130 w4314 w4527 w4760 w4889] -> w163
      tunnel: w114 -> [_ _ _ _ _ _ _ _ _ _ _ _ _ _ _ _ _ w3241 _ _ _ _ _ _ _ w3967 _ _ _ _ w4867]
      tunnel: [w253 refnum<visa-resource-name> refnum ("VISA resource name out") w488 w674 w749 w797 w885 w1214 w1291 w1739 w1863 w2101 w2392 w2478 w2762 w2910 w3061 w3227 w3438 w3630 w3687 w3745 w3800 w3857 w3918 w3961 w4121 w4313 w4521 w4713 w4888] -> w159
      tunnel: w158 -> [w253 _ _ w674 w749 w797 w885 w1214 w1291 w1739 w1863 w2101 w2392 w2478 w2762 w2910 w3061 w3227 w3438 w3630 w3687 w3745 w3800 w3857 w3918 w3961 w4121 w4313 w4521 w4713 w4888]
      tunnel: w157 -> [w252 w301 w487 w673 w748 w796 w884 w1204 w1278 w1738 w1862 _ w2391 w2477 w2761 w2909 w3060 w3226 w3437 w3629 w3686 w3744 w3799 w3856 w3917 w3960 w4120 w4312 w4520 w4726 w4887]
      tunnel: [w252 w301 w487 w673 w748 w796 w884 w1204 w1278 w1738 w1862 0 ("Larva # to move") w2391 w2477 w2761 w2909 w3060 w3225 w3436 w3629 w3686 w3744 w3799 w3856 w3917 w3960 w4120 w4312 w4520 w4726 w4887] -> w156
      tunnel: [w251 w300 w486 w672 w747 w795 w883 w1223 w1277 w1737 w1861 w2100 w2390 w2469 w2720 w2908 w3059 w3223 w3435 w3628 w3685 w3743 w3798 w3855 w3916 w3959 w4119 w4311 w4519 w4725 w4886] -> w155
      tunnel: w154 -> [w251 w300 w486 w672 w747 w795 w882 w1223 w1277 w1737 w1861 w2100 w2390 w2469 w2720 w2908 w3059 w3223 w3435 w3628 w3685 w3743 w3798 w3855 w3916 w3959 w4119 w4311 w4519 w4725 w4886]
      tunnel: [_ _ _ _ _ _ w881 _ _ _ _ _ _ _ _ _ _ _ _ _ _ _ _ _ _ _ _ _ _ _ _] -> w153
      tunnel: w152 -> [w239 w288 w463 w651 w746 w785 w853 w1205 w1267 w1687 w1821 w2053 w2389 w2465 w2713 w2890 w3035 w3193 w3407 w3602 w3659 w3722 w3771 w3829 w3915 w3947 w4109 w4310 w4508 w4705 w4876]
      tunnel: [w239 w288 w463 w651 w746 w785 w853 w1205 w1267 w1687 w1821 w1927 w2389 w2465 w2713 w2890 w3035 w3193 w3407 w3602 w3659 w3722 w3771 w3829 w3915 w3947 w4109 w4310 w4508 w4705 w4876] -> w151
      tunnel: [w250 w298 w484 w663 w745 w793 w878 w1221 w1275 w1736 w1860 w2051 w2388 w2474 w2743 w2906 w3027 w3215 w3402 w3627 w3684 w3742 w3797 w3854 w3914 w3955 w4117 w4309 w4516 w4723 w4884] -> w141
      tunnel: [w249 w297 w483 w662 w744 w792 w877 w1220 w1274 w1735 w1859 w2050 w2387 w2473 w2742 w2902 w3057 w3214 w3430 w3626 w3683 w3741 w3796 w3853 w3913 w3954 w4116 w4308 w4515 w4722 w4883] -> w140
      tunnel: [w248 w299 w485 w664 w743 w794 w879 w1222 w1276 w1734 w1858 w2052 w2386 w2475 w2733 w2900 w3058 w3216 w3405 w3625 w3682 w3740 w3795 w3852 w3912 w3956 w4118 w4307 w4517 w4724 w4885] -> w139
      tunnel: w138 -> [w248 w299 w485 w664 w743 w794 w879 w1222 w1276 w1734 w1858 w2052 w2386 w2475 _ w2900 w3058 w3216 w3405 w3625 w3682 w3740 w3795 w3852 w3912 w3956 w4118 w4307 w4517 w4724 w4885]
      tunnel: w137 -> [w250 w298 w484 w663 w745 w793 w878 w1221 w1275 w1736 w1860 w2051 w2388 w2474 _ w2906 w3027 w3215 w3402 w3627 w3684 w3742 w3797 w3854 w3914 w3955 w4117 w4309 w4516 w4723 w4884]
      tunnel: w136 -> [w249 w297 w483 w662 w744 w792 w877 w1220 w1274 w1735 w1859 w2050 w2387 w2473 _ w2902 w3057 w3214 w3430 w3626 w3683 w3741 w3796 w3853 w3913 w3954 w4116 w4308 w4515 w4722 w4883]
      tunnel: [w245 w294 w473 w659 w742 w791 w876 w1219 w1273 w1733 w1857 w2049 w2385 w2472 w2730 w2897 w3056 w3212 w3423 w3624 w3681 w3739 w3794 w3851 w3911 w3953 w4115 w4306 w4514 w4721 w4882] -> w135
      tunnel: [w244 w293 w468 w658 w741 w790 w875 w1218 w1272 w1732 w1856 w2048 w2384 w2471 w2729 w2896 w3055 w3211 w3416 w3615 w3672 w3731 w3785 w3842 w3910 w3952 w4114 w4305 w4513 w4719 w4881] -> w134
      tunnel: w133 -> [w245 w294 _ w659 w742 w791 w876 w1219 w1273 w1733 w1857 w2049 w2385 w2472 w2730 w2897 w3056 w3212 w3423 w3624 w3681 w3739 w3794 w3851 w3911 w3953 w4115 w4306 w4514 w4721 w4882]
      tunnel: w94 -> [w244 w293 _ w658 w741 w790 w875 w1218 w1272 w1732 w1856 w2048 w2384 w2471 w2729 w2896 w3055 w3211 w3416 w3616 w3673 w3732 w3786 w3843 w3910 w3952 w4114 w4305 w4513 w4719 w4881]
      tunnel: w126 -> [_ _ _ w655 _ _ _ _ _ _ _ _ _ _ _ _ _ _ _ w3620 w3677 w3736 w3790 w3847 _ _ _ _ _ _ _]
      tunnel: w132 -> [_ _ _ _ _ _ _ _ _ _ _ _ _ _ _ _ _ _ _ _ _ _ _ _ _ _ _ _ _ _ _]
      tunnel: w131 -> [w243 w292 w472 w657 w740 w789 w874 w1217 w1271 w1731 w1855 w2047 w2383 w2470 w2724 w2894 w3054 w3210 w3415 w3608 w3665 w3727 w3777 w3835 w3909 w3951 w4113 w4304 w4512 w4718 w4880]
      tunnel: [w243 w292 w472 w657 w740 w789 w872 w1217 w1271 w1731 w1855 w2047 w2383 w2470 w2724 w2894 w3054 w3210 w3415 w3608 w3665 w3727 w3777 w3835 w3909 w3951 w4113 w4304 w4512 w4718 w4880] -> w129
      tunnel: w128 -> [w242 w291 w466 w656 w739 w788 w870 w1216 w1270 w1730 w1854 w2046 w2382 w2468 w2722 w2893 w3053 w3209 w3413 w3606 w3663 w3725 w3775 w3833 w3908 w3950 w4112 w4303 w4511 w4717 w4879]
      tunnel: [w242 w291 w466 w656 w739 w788 w870 w1216 w1270 w1730 w1854 w2046 w2382 w2468 w2721 w2893 w3053 w3209 w3413 w3606 w3663 w3725 w3775 w3833 w3908 w3950 w4112 w4303 w4511 w4717 w4879] -> w127
      tunnel: w124 -> [_ _ _ _ _ _ _ _ _ w1726 w1852 w2042 _ _ _ _ _ _ _ _ _ _ _ _ _ _ _ _ _ _ _]
      tunnel: [_ _ _ _ _ _ _ _ _ w1723 w1849 w2041 _ _ _ _ _ _ _ _ _ _ _ _ _ _ _ _ _ _ _] -> w123
      tunnel: w122 -> [w241 w290 w465 w653 w738 w787 w868 _ w1269 w1699 w1833 w2019 w2381 w2467 w2719 w2892 w3052 w3205 w3412 w3605 w3662 w3724 w3774 w3832 w3907 w3949 w4111 w4302 w4510 w4716 w4878]
      tunnel: [w241 w290 w465 w653 w738 w787 w866 0 w1269 w1699 w1833 w2019 w2381 w2467 w2719 w2892 w3052 w3205 w3412 w3605 w3662 w3724 w3774 w3832 w3907 w3949 w4111 w4302 w4510 w4716 w4878] -> w121
      tunnel: w120 -> [w240 w289 w464 w652 w737 w786 w864 w1208 w1268 w1698 w1832 w2018 w2380 w2466 w2718 w2891 w3051 w3204 w3411 w3604 w3661 w3723 w3773 w3831 w3906 w3948 w4110 w4301 w4509 w4715 w4877]
      tunnel: [w240 w289 w464 w652 w737 w786 w864 w1207 w1268 w1698 w1832 w2018 w2380 w2466 w2718 w2891 w3051 w3204 w3411 w3604 w3661 w3723 w3773 w3831 w3906 w3948 w4110 w4301 w4509 w4715 w4877] -> w119
      tunnel: w118 -> [_ _ _ _ _ _ _ w1206 _ _ _ w2009 _ _ _ _ _ _ _ _ _ _ _ _ _ _ _ _ _ w4706 _]
      tunnel: w117 -> [w238 w287 w462 w650 w736 w784 w858 w1203 w1266 w1686 w1820 w2008 w2379 w2464 w2712 w2889 w3034 w3192 w3406 w3601 w3658 w3721 w3770 w3828 w3905 w3946 w4108 w4300 w4507 w4704 w4875]
      tunnel: [w238 w287 w462 w650 w736 w784 w858 w1203 w1266 w1686 w1820 w2008 w2379 w2464 w2712 w2884 w3034 w3192 w3406 w3601 w3658 w3721 w3770 w3828 w3905 w3946 w4108 w4300 w4507 w4704 w4875] -> w116
      tunnel: "real laser power" -> [_ _ _ _ _ _ _ _ _ _ _ _ _ _ _ _ _ _ _ _ _ _ _ _ _ _ _ _ _ _ w4866]
      tunnel: w99 -> [w237 w280 w457 w648 w722 w783 w857 w1202 w1265 w1676 w1809 w1930 w2337 w2463 w2687 w2881 w3029 w3187 w3401 w3600 w3657 w3720 w3769 w3827 w3904 w3945 w4105 w4293 w4505 w4702 w4865]
      tunnel: [w237 w280 w457 w648 w722 w783 w857 w1202 w1265 w1676 w1809 w1930 w2337 w2463 w2687 w2881 w3029 w3187 w3401 w3600 w3657 w3719 w3769 w3827 w3904 w3945 w4105 w4293 w4505 w4702 w4865] -> w98
      tunnel: w96 -> [w236 w279 w456 w647 w721 w782 w856 w1201 w1264 w1675 w1808 w1929 w2336 w2462 w2686 w2880 w3026 w3186 w3400 w3599 w3656 w3718 w3768 w3826 w3903 w3944 w4104 w4292 w4504 w4701 w4864]
      tunnel: [w236 w278 w456 w647 w721 w782 w855 w1201 w1264 w1675 w1808 w1929 w2336 w2462 w2686 w2880 w3026 w3186 w3400 w3599 w3656 w3718 w3768 w3826 w3903 w3944 w4104 w4292 w4504 w4701 w4864] -> w95
      tunnel: w93 -> [_ _ _ _ _ _ _ _ _ _ _ _ _ _ _ _ _ _ _ _ _ _ _ _ _ _ _ _ _ _ w4863]
      tunnel: w92 -> [w235 w275 w455 w646 w720 w781 w850 w1200 w1263 w1674 w1807 w1924 w2335 w2461 w2679 w2879 w3023 w3185 w3398 w3598 w3655 w3712 w3767 w3825 w3882 w3943 w4103 w4291 w4503 w4700 w4862]
      tunnel: [w235 w275 w455 w646 w720 w781 w850 w1200 w1263 w1674 w1807 w1924 w2335 w2461 w2679 w2879 w3023 w3185 w3398 w3598 w3655 w3712 w3767 w3825 w3882 w3943 w4103 w4291 w4503 w4700 w4862] -> w91
      tunnel: [w234 w274 w454 w645 w719 w780 w849 w1199 w1262 w1673 w1806 w1923 w2334 w2460 w2678 w2878 w3022 w3184 w3397 w3597 w3654 w3711 w3766 w3824 w3881 w3942 w4102 w4290 w4502 w4699 w4861] -> w90
      tunnel: w89 -> [w234 w274 w454 w645 w719 w780 w849 w1199 w1262 w1673 w1806 w1923 w2334 w2460 w2678 w2878 w3022 w3184 w3397 w3597 w3654 w3711 w3766 w3824 w3881 w3942 _ w4290 _ w4699 w4861]
      frame "4c?" {
        n54 = case shown="True" "4C" {
          tunnel: [states."Initialize" states."stopflow triggertest"] -> w247
          frame False {
          }
          frame True {
          }
        }
      }
      frame "Initialize" {
        w344 = 1 items=["Snap", "Sequence"] ("Capture mode")
        w351 = u32 4343216 items=["SENSOR MODE"=4212128, "SENSOR MODE LINE BUNDLE HEIGHT"=4212192, "READOUT DIRECTION"=4211904, "BIT PER CHANNEL"=4342976, "EXPOSURE TIME"=2049184, "CONTRAST GAIN"=3163312, "BINNING"=4215968, "TIMING READOUT TIME"=4223904, "INTERNAL FRAME RATE"=4225952, "INTERNAL FRAME INTERVAL"=4225968, "INTERNAL LINE SPEED"=4226000, "IMAGE WIDTH"=4343200, "IMAGE HEIGHT"=4343216, "IMAGE ROWBYTES"=4343232, "IMAGE FRAMEBYTES"=4343248, "IMAGE PIXEL TYPE"=4343296] ("Parameter")
        w352 = u32 4343200 items=["SENSOR MODE"=4212128, "SENSOR MODE LINE BUNDLE HEIGHT"=4212192, "READOUT DIRECTION"=4211904, "BIT PER CHANNEL"=4342976, "EXPOSURE TIME"=2049184, "CONTRAST GAIN"=3163312, "BINNING"=4215968, "TIMING READOUT TIME"=4223904, "INTERNAL FRAME RATE"=4225952, "INTERNAL FRAME INTERVAL"=4225968, "INTERNAL LINE SPEED"=4226000, "IMAGE WIDTH"=4343200, "IMAGE HEIGHT"=4343216, "IMAGE ROWBYTES"=4343232, "IMAGE FRAMEBYTES"=4343248, "IMAGE PIXEL TYPE"=4343296] ("Parameter")
        (unwired) u32 120000 ("timeout (10sec)")
        (unwired) enum16{"None", "Odd", "Even", "Mark", "Space"}."None" ("parity (0:none)")
        (unwired) u16 8 ("data bits (8)")
        w364 = u32 2 items=["FORWARD"=1, "BACKWARD"=2] ("Readout Direction")
        w391 = u32 2049184 items=["SENSOR MODE"=4212128, "SENSOR MODE LINE BUNDLE HEIGHT"=4212192, "READOUT DIRECTION"=4211904, "BIT PER CHANNEL"=4342976, "EXPOSURE TIME"=2049184, "CONTRAST GAIN"=3163312, "BINNING"=4215968, "TIMING READOUT TIME"=4223904, "INTERNAL FRAME RATE"=4225952, "INTERNAL FRAME INTERVAL"=4225968, "INTERNAL LINE SPEED"=4226000, "IMAGE WIDTH"=4343200, "IMAGE HEIGHT"=4343216, "IMAGE ROWBYTES"=4343232, "IMAGE FRAMEBYTES"=4343248, "IMAGE PIXEL TYPE"=4343296] ("Parameter")
        w385 = 2 items=["Internal"=1, "External"=2, "Software"=3, "Master Pulse"=4] ("Source")
        w372 = u32 2 items=["NEGATIVE"=1, "POSITIVE"=2] ("Output Trigger Polarity")
        w380 = u32 3 items=["LOW"=1, "GLOBAL EXPOSURE"=2, "PROGRAMMABLE"=3, "TRIGGER READY"=4, "HIGH"=5] ("Output Trigger Mode")
        w377 = u32 4 items=["Exposure"=1, "Readout End"=2, "V Sync"=3, "H Sync"=4, "Trigger"=6] ("Source")
        w371 = u32 4226016 items=["SENSOR MODE"=4212128, "CCD MODE"=4212384, "READOUT MODE"=4211872, "ACTIVE VIEW INDEX"=4343136, "BITS PER CHANNEL"=4342976, "IMAGE PIXEL TYPE"=4343296, "BINNING"=4215968, "EXPOSURE TIME"=2049184, "CONTRAST GAIN"=3163312, "CONTRAST OFFSET"=3163328, "LIGHT MODE"=2114720, "SENSITIVITY"=2114992, "PHOTON IMAGING MODE"=2115200, "HIGH DYNAMIC RANGE MODE"=3163360, "WHITE BALANCE"=3163568, "TEMPERATURE"=2115232, "TEMPERATURE TARGET"=2115264, "SENSOR COOLER FAN"=2115296, "LINEBUNDLE HEIGHT"=4212192, "MECHANICAL SHUTTER"=2115488, "BACK FOCUS POSITION"=8422304, "TRIGGER CONNECTOR"=1066432, "TRIGGER SOURCE"=1066144, "OUTPUT TRIGGER SOURCE"=1852576, "TRIGGER GLOBAL EXPOSURE"=2049680, "FIRST TRIGGER BEHAVIOR"=2049696, "CHANNEL SYNC"=1852352, "READOUT DIRECTION"=4211904, "PRE HSYNC COUNT"=1852704, "INTERNAL LINE SPEED"=4226000, "INTERNAL LINE INTERVAL"=4226016] ("Parameter")
        w368 = u32 4212128 items=["SENSOR MODE"=4212128, "CCD MODE"=4212384, "READOUT MODE"=4211872, "ACTIVE VIEW INDEX"=4343136, "BITS PER CHANNEL"=4342976, "IMAGE PIXEL TYPE"=4343296, "BINNING"=4215968, "EXPOSURE TIME"=2049184, "CONTRAST GAIN"=3163312, "CONTRAST OFFSET"=3163328, "LIGHT MODE"=2114720, "SENSITIVITY"=2114992, "PHOTON IMAGING MODE"=2115200, "HIGH DYNAMIC RANGE MODE"=3163360, "WHITE BALANCE"=3163568, "TEMPERATURE"=2115232, "TEMPERATURE TARGET"=2115264, "SENSOR COOLER FAN"=2115296, "LINEBUNDLE HEIGHT"=4212192, "MECHANICAL SHUTTER"=2115488, "BACK FOCUS POSITION"=8422304, "TRIGGER CONNECTOR"=1066432, "TRIGGER SOURCE"=1066144, "OUTPUT TRIGGER SOURCE"=1852576, "TRIGGER GLOBAL EXPOSURE"=2049680, "FIRST TRIGGER BEHAVIOR"=2049696, "CHANNEL SYNC"=1852352, "READOUT DIRECTION"=4211904, "PRE HSYNC COUNT"=1852704, "INTERNAL LINE SPEED"=4191408, "INTERNAL LINE INTERVAL"=4191424] ("Parameter")
        w367 = u32 1852704 items=["SENSOR MODE"=4212128, "CCD MODE"=4212384, "READOUT MODE"=4211872, "ACTIVE VIEW INDEX"=4343136, "BITS PER CHANNEL"=4342976, "IMAGE PIXEL TYPE"=4343296, "BINNING"=4215968, "EXPOSURE TIME"=2049184, "CONTRAST GAIN"=3163312, "CONTRAST OFFSET"=3163328, "LIGHT MODE"=2114720, "SENSITIVITY"=2114992, "PHOTON IMAGING MODE"=2115200, "HIGH DYNAMIC RANGE MODE"=3163360, "WHITE BALANCE"=3163568, "TEMPERATURE"=2115232, "TEMPERATURE TARGET"=2115264, "SENSOR COOLER FAN"=2115296, "LINEBUNDLE HEIGHT"=4212192, "MECHANICAL SHUTTER"=2115488, "BACK FOCUS POSITION"=8422304, "TRIGGER CONNECTOR"=1066432, "TRIGGER SOURCE"=1066144, "OUTPUT TRIGGER SOURCE"=1852576, "TRIGGER GLOBAL EXPOSURE"=2049680, "FIRST TRIGGER BEHAVIOR"=2049696, "CHANNEL SYNC"=1852352, "READOUT DIRECTION"=4211904, "PRE HSYNC COUNT"=1852704, "INTERNAL LINE SPEED"=4191408, "INTERNAL LINE INTERVAL"=4191424] ("Parameter")
        w366 = u32 4211904 items=["SENSOR MODE"=4212128, "CCD MODE"=4212384, "READOUT MODE"=4211872, "ACTIVE VIEW INDEX"=4343136, "BITS PER CHANNEL"=4342976, "IMAGE PIXEL TYPE"=4343296, "BINNING"=4215968, "EXPOSURE TIME"=2049184, "CONTRAST GAIN"=3163312, "CONTRAST OFFSET"=3163328, "LIGHT MODE"=2114720, "SENSITIVITY"=2114992, "PHOTON IMAGING MODE"=2115200, "HIGH DYNAMIC RANGE MODE"=3163360, "WHITE BALANCE"=3163568, "TEMPERATURE"=2115232, "TEMPERATURE TARGET"=2115264, "SENSOR COOLER FAN"=2115296, "LINEBUNDLE HEIGHT"=4212192, "MECHANICAL SHUTTER"=2115488, "BACK FOCUS POSITION"=8422304, "TRIGGER CONNECTOR"=1066432, "TRIGGER SOURCE"=1066144, "OUTPUT TRIGGER SOURCE"=1852576, "TRIGGER GLOBAL EXPOSURE"=2049680, "FIRST TRIGGER BEHAVIOR"=2049696, "CHANNEL SYNC"=1852352, "READOUT DIRECTION"=4211904, "PRE HSYNC COUNT"=1852704, "INTERNAL LINE SPEED"=4191408, "INTERNAL LINE INTERVAL"=4191424] ("Parameter")
        n55 = call <userlib>:"tm_initialize_40.vi"() -> ("error out"=w357:errorcluster)  [unwired: 8 in, 3 out]
        n56 = call <userlib>:"tm_opencamera_40.vi"("error in (no error)"=w357, "Camera Index"=u32 0) -> ("error out"=w381:errorcluster, "Handle out"=w382:u32)  [unwired: 7 in, 1 out]
        n57 = call-poly <vilib>:"DAQmx Create Virtual Channel.vi"("lines"=tag "Dev1/port0/line6") -> ("task out"=w324:refnum<k21>, "error out"=w323:errorcluster)  [unwired: 13 in]
        n58 = Wait (ms)(milliseconds to wait=u32 500) -> ()  [unwired: 1 out]
        n59 = call <vilib>:"DAQmx Start Task.vi"("task/channels in"=w324, "error in"=w323) -> ("task out"=w321:refnum<k21>, "error out"=w320:errorcluster)  [unwired: 12 in]
        n60 = call <userlib>:"tm_setparameter_40.vi"("error in (no error)"=w381, "Value in"=12.0, "Parameter"=w368, "Handle in"=w382) -> ("error out"=w379:errorcluster, "Handle out"=w378:u32)  [unwired: 6 in]
        n61 = call-poly <vilib>:"DAQmx Write.vi"("task/channels in"=w321, "data"=FALSE, "error in"=w320) -> ("task out"=w318:refnum<k21>, "error out"=w317:errorcluster)  [unwired: 10 in, 1 out]
        n62 = call <vilib>:"DAQmx Stop Task.vi"("task/channels in"=w318, "error in"=w317) -> ("task out"=w316:refnum<k21>, "error out"=w315:errorcluster)  [unwired: 12 in]
        n63 = call <vilib>:"DAQmx Clear Task.vi"("task in"=w316, "error in"=w315) -> ()  [unwired: 13 in, 1 out]
        n64 = call "RS232C_Init.vi"("baud rate"=u16 9600 ("baud rate 2"), "COM Port"=refnum<visa-resource-name> "COM9" ("VISA resource name")) -> ("VISA resource name out"=w276:refnum<visa-resource-name>)  [unwired: 1 in, 2 out]
        n65 = To Double Precision Float(number=w364) -> (double precision float=w363:dbl)
        n66 = To Double Precision Float(number=u32 0) -> (double precision float=w360:dbl)
        n67 = call <vilib>:"High Resolution Relative Seconds.vi"() -> ("relative seconds"=→"experiment start time (relative)":dbl)
        n68 = call <userlib>:"tm_setparameter_40.vi"("error in (no error)"=w379, "Value in"=w360, "Parameter"=w367, "Handle in"=w378) -> ("error out"=w361:errorcluster, "Handle out"=w362:u32)  [unwired: 6 in]
        n69 = call <userlib>:"tm_setparameter_40.vi"("error in (no error)"=w361, "Value in"=w363, "Parameter"=w366, "Handle in"=w362) -> ("error out"=w370:errorcluster, "Handle out"=w369:u32)  [unwired: 6 in]
        n70 = call <userlib>:"tm_setparameter_40.vi"("error in (no error)"=w370, "Value in"=9.74436e-06, "Parameter"=w371, "Handle in"=w369) -> ("error out"=w390:errorcluster, "Handle out"=w389:u32)  [unwired: 6 in]
        n71 = flat-sequence {
          tunnel: refnum<visa-resource-name> "USB0::0x1AB1::0x0643::DG9A242400208::INSTR" ("VISA resource name") -> [w399]
          tunnel: [w397] -> w311
          tunnel: refnum<visa-resource-name> "USB0::0x1AB1::0x0643::DG9A242400205::INSTR" ("VISA resource name") -> [w396]
          tunnel: [w395] -> w308
          tunnel: w311 -> [w404]
          tunnel: [w404] -> w310
          tunnel: w308 -> [w401]
          tunnel: [w400] -> w307
          tunnel: w310 -> [w409]
          tunnel: [w409] -> w312
          tunnel: w307 -> [w407]
          tunnel: [w405] -> w304
          tunnel: w312 -> [w414]
          tunnel: [w411] -> w314
          tunnel: [w410] -> w305
          tunnel: w304 -> [w410]
          tunnel: w314 -> [w419]
          tunnel: [w416] -> w313
          tunnel: [w415] -> w306
          tunnel: w305 -> [w415]
          tunnel: w313 -> [w424]
          tunnel: [w421] -> w284
          tunnel: w306 -> [w421]
          tunnel: [w420] -> w282
          tunnel: w284 -> [w429]
          tunnel: [w429] -> w283
          tunnel: w282 -> [w427]
          tunnel: [w425] -> w281
          tunnel: [w430] -> w303
          tunnel: w283 -> [w434]
          tunnel: [w434] -> w302
          tunnel: w281 -> [w431]
          tunnel: w303 -> [w437]
          tunnel: w302 -> [w435]
          frame #0 {
            n72 = VISA Open(VISA resource name=w399) -> (VISA resource name=w397:refnum<visa-resource-name>)  [unwired: 4 in, 1 out]
            n73 = VISA Open(VISA resource name=w396) -> (VISA resource name=w395:refnum<visa-resource-name>)  [unwired: 4 in, 1 out]
            n74 = Wait (ms)(milliseconds to wait=u32 500) -> ()  [unwired: 1 out]
          }
          frame #1 {
            n75 = Wait (ms)(milliseconds to wait=u32 500) -> ()  [unwired: 1 out]
            n76 = VISA Write(VISA resource name=w401, write buffer=":OUTP2 ON") -> (VISA resource name out=w400:refnum<visa-resource-name>)  [unwired: 1 in, 2 out]
          }
          frame #2 {
            n77 = Wait (ms)(milliseconds to wait=u32 500) -> ()  [unwired: 1 out]
            n78 = VISA Write(VISA resource name=w407, write buffer=":OUTP1 ON") -> (VISA resource name out=w405:refnum<visa-resource-name>)  [unwired: 1 in, 2 out]
          }
          frame #3 {
            n79 = Wait (ms)(milliseconds to wait=u32 500) -> ()  [unwired: 1 out]
            n80 = VISA Write(VISA resource name=w414, write buffer=":OUTP2 ON") -> (VISA resource name out=w411:refnum<visa-resource-name>)  [unwired: 1 in, 2 out]
          }
          frame #4 {
            n81 = Wait (ms)(milliseconds to wait=u32 500) -> ()  [unwired: 1 out]
            n82 = VISA Write(VISA resource name=w419, write buffer=":OUTP1 ON") -> (VISA resource name out=w416:refnum<visa-resource-name>)  [unwired: 1 in, 2 out]
          }
          frame #5 {
            n83 = Wait (ms)(milliseconds to wait=u32 500) -> ()  [unwired: 1 out]
            n84 = VISA Write(VISA resource name=w424, write buffer=":TRIG1") -> (VISA resource name out=w420:refnum<visa-resource-name>)  [unwired: 1 in, 2 out]
          }
          frame #6 {
            n85 = Wait (ms)(milliseconds to wait=u32 500) -> ()  [unwired: 1 out]
            n86 = VISA Write(VISA resource name=w427, write buffer=":TRIG2") -> (VISA resource name out=w425:refnum<visa-resource-name>)  [unwired: 1 in, 2 out]
          }
          frame #7 {
            n87 = VISA Write(VISA resource name=w431, write buffer=":TRIG2") -> (VISA resource name out=w430:refnum<visa-resource-name>)  [unwired: 1 in, 2 out]
            n88 = Wait (ms)(milliseconds to wait=u32 500) -> ()  [unwired: 1 out]
          }
          frame #8 {
            n89 = VISA Clear(VISA resource name=w435) -> ()  [unwired: 1 in, 2 out]
            n90 = VISA Clear(VISA resource name=w437) -> ()  [unwired: 1 in, 2 out]
            n91 = Wait (ms)(milliseconds to wait=u32 200) -> ()  [unwired: 1 out]
          }
        }
        n92 = call <userlib>:"tm_setparameter_40.vi"("error in (no error)"=w390, "Value in"=0.0195, "Parameter"=w391, "Handle in"=w389) -> ("error out"=w388:errorcluster, "Handle out"=w387:u32)  [unwired: 6 in]
        n93 = Bundle("Output Trigger Period"=1e-06, "Delay"=0.0, "Source"=w377) -> (w374:T6)  [unwired: 1 in]
        n94 = call <userlib>:"tm_inputtriggersource_40.vi"("error in (no error)"=w388, "External Options"=cluster{"Polarity":i32, "Delay":dbl} {"Polarity"=2, "Delay"=0.0}, "Source"=w385, "Handle in"=w387) -> ("error out"=w384:errorcluster, "Handle out"=w383:u32)  [unwired: 6 in]
        n95 = Bundle("Output Trigger Mode"=w380, "Output Trigger Polarity"=w372) -> (w373:T7)  [unwired: 1 in]
        n96 = call <userlib>:"tm_setoutputtrigger_40.vi"("Port"=0 ("Index"), "error in (no error)"=w384, "Programmable Options"=w374, "Type"=w373, "Handle in"=w383) -> ("error out"=w348:errorcluster, "Handle out"=w342:u32)  [unwired: 5 in]
        n97 = call <userlib>:"tm_getparameter_40.vi"("error in (no error)"=w348, "Parameter"=w351, "Handle in"=w342) -> ("error out"=w350:errorcluster, "Value out"=w353:dbl, "Handle out"=w341:u32)  [unwired: 6 in]
        n98 = call <userlib>:"tm_getparameter_40.vi"("error in (no error)"=w350, "Parameter"=w352, "Handle in"=w341) -> ("error out"=w349:errorcluster, "Value out"=w354:dbl)  [unwired: 6 in, 1 out]
        n99 = for {
          N: "Frames in memory" -> [_]
          tunnel: [w445] -> w345 mode=indexing
          tunnel: [w444] -> w347
          tunnel: w349 -> [w442]
          tunnel: w354 -> [w441]
          tunnel: w353 -> [w440]
          tunnel: [w439] -> w340 mode=indexing
          i -> [w449]
          w446 = T8 7 items=["Grayscale (U8)", "Grayscale (I16)", "Grayscale (SGL)", "Complex (CSG)", "RGB (U32)", "HSL (U32)", "RGB (U64)", "Grayscale (U16)"] ("Image Type")
          w451 = 0
          n100 = Number To Decimal String(number=w449, width (-)=i16 3) -> (decimal integer string=w450:string)
          n101 = call "IMAQ Create"("Border Size"=0, "Image Name"=w450, "Image Type"=w446, "error in (no error)"=w442) -> ("New Image"=w438:T9, "error out"=w453:errorcluster)  [unwired: 1 in]
          n102 = call "IMAQ SetImageSize"("error in (no error)"=w453, "Y Resolution"=w440, "X Resolution"=w441, "Image"=w438) -> ("error out"=w452:errorcluster, "Image Out"=w439:T9)  [unwired: 1 in]
          n103 = call "IMAQ GetImagePixelPtr"("Function"=T5."Map Pixel Pointer", "error in (no error)"=w452, "Y Coordinate"=w451, "X Coordinate"=w451, "Image"=w439) -> ("error out"=w444:errorcluster, "Pixel Pointer out"=w445:u64)  [unwired: 1 in, 4 out]
        }
        n104 = call <userlib>:"tm_prepare_attach_40.vi"("error in (no error)"=w347, "buffers"=w345, "Capture mode"=w344) -> ("error out"=w346:errorcluster, "Handle out"=w343:u32)  [unwired: 7 in]
        n105 = shared-variable-read(w279) -> (w278:refnum<k21>)  [unwired: 2 in, 3 out]
      }
      frame "initialize_2" {
        w531 = 1 items=["Snap", "Sequence"] ("Capture mode")
        w538 = u32 4343216 items=["SENSOR MODE"=4212128, "SENSOR MODE LINE BUNDLE HEIGHT"=4212192, "READOUT DIRECTION"=4211904, "BIT PER CHANNEL"=4342976, "EXPOSURE TIME"=2049184, "CONTRAST GAIN"=3163312, "BINNING"=4215968, "TIMING READOUT TIME"=4223904, "INTERNAL FRAME RATE"=4225952, "INTERNAL FRAME INTERVAL"=4225968, "INTERNAL LINE SPEED"=4226000, "IMAGE WIDTH"=4343200, "IMAGE HEIGHT"=4343216, "IMAGE ROWBYTES"=4343232, "IMAGE FRAMEBYTES"=4343248, "IMAGE PIXEL TYPE"=4343296] ("Parameter")
        w539 = u32 4343200 items=["SENSOR MODE"=4212128, "SENSOR MODE LINE BUNDLE HEIGHT"=4212192, "READOUT DIRECTION"=4211904, "BIT PER CHANNEL"=4342976, "EXPOSURE TIME"=2049184, "CONTRAST GAIN"=3163312, "BINNING"=4215968, "TIMING READOUT TIME"=4223904, "INTERNAL FRAME RATE"=4225952, "INTERNAL FRAME INTERVAL"=4225968, "INTERNAL LINE SPEED"=4226000, "IMAGE WIDTH"=4343200, "IMAGE HEIGHT"=4343216, "IMAGE ROWBYTES"=4343232, "IMAGE FRAMEBYTES"=4343248, "IMAGE PIXEL TYPE"=4343296] ("Parameter")
        w545 = u16 0 items=["なし", "XON/XOFF", "RTS/CTS", "XON/XOFF & RTS/CTS", "DTR/DSR", "XON/XOFF & DTR/DSR"] ("flow control (0:none)")
        w556 = u32 2 items=["FORWARD"=1, "BACKWARD"=2] ("Readout Direction")
        w583 = u32 2049184 items=["SENSOR MODE"=4212128, "SENSOR MODE LINE BUNDLE HEIGHT"=4212192, "READOUT DIRECTION"=4211904, "BIT PER CHANNEL"=4342976, "EXPOSURE TIME"=2049184, "CONTRAST GAIN"=3163312, "BINNING"=4215968, "TIMING READOUT TIME"=4223904, "INTERNAL FRAME RATE"=4225952, "INTERNAL FRAME INTERVAL"=4225968, "INTERNAL LINE SPEED"=4226000, "IMAGE WIDTH"=4343200, "IMAGE HEIGHT"=4343216, "IMAGE ROWBYTES"=4343232, "IMAGE FRAMEBYTES"=4343248, "IMAGE PIXEL TYPE"=4343296] ("Parameter")
        w577 = 2 items=["Internal"=1, "External"=2, "Software"=3, "Master Pulse"=4] ("Source")
        w564 = u32 2 items=["NEGATIVE"=1, "POSITIVE"=2] ("Output Trigger Polarity")
        w572 = u32 3 items=["LOW"=1, "GLOBAL EXPOSURE"=2, "PROGRAMMABLE"=3, "TRIGGER READY"=4, "HIGH"=5] ("Output Trigger Mode")
        w569 = u32 4 items=["Exposure"=1, "Readout End"=2, "V Sync"=3, "H Sync"=4, "Trigger"=6] ("Source")
        w563 = u32 4226016 items=["SENSOR MODE"=4212128, "CCD MODE"=4212384, "READOUT MODE"=4211872, "ACTIVE VIEW INDEX"=4343136, "BITS PER CHANNEL"=4342976, "IMAGE PIXEL TYPE"=4343296, "BINNING"=4215968, "EXPOSURE TIME"=2049184, "CONTRAST GAIN"=3163312, "CONTRAST OFFSET"=3163328, "LIGHT MODE"=2114720, "SENSITIVITY"=2114992, "PHOTON IMAGING MODE"=2115200, "HIGH DYNAMIC RANGE MODE"=3163360, "WHITE BALANCE"=3163568, "TEMPERATURE"=2115232, "TEMPERATURE TARGET"=2115264, "SENSOR COOLER FAN"=2115296, "LINEBUNDLE HEIGHT"=4212192, "MECHANICAL SHUTTER"=2115488, "BACK FOCUS POSITION"=8422304, "TRIGGER CONNECTOR"=1066432, "TRIGGER SOURCE"=1066144, "OUTPUT TRIGGER SOURCE"=1852576, "TRIGGER GLOBAL EXPOSURE"=2049680, "FIRST TRIGGER BEHAVIOR"=2049696, "CHANNEL SYNC"=1852352, "READOUT DIRECTION"=4211904, "PRE HSYNC COUNT"=1852704, "INTERNAL LINE SPEED"=4226000, "INTERNAL LINE INTERVAL"=4226016] ("Parameter")
        w560 = u32 4212128 items=["SENSOR MODE"=4212128, "CCD MODE"=4212384, "READOUT MODE"=4211872, "ACTIVE VIEW INDEX"=4343136, "BITS PER CHANNEL"=4342976, "IMAGE PIXEL TYPE"=4343296, "BINNING"=4215968, "EXPOSURE TIME"=2049184, "CONTRAST GAIN"=3163312, "CONTRAST OFFSET"=3163328, "LIGHT MODE"=2114720, "SENSITIVITY"=2114992, "PHOTON IMAGING MODE"=2115200, "HIGH DYNAMIC RANGE MODE"=3163360, "WHITE BALANCE"=3163568, "TEMPERATURE"=2115232, "TEMPERATURE TARGET"=2115264, "SENSOR COOLER FAN"=2115296, "LINEBUNDLE HEIGHT"=4212192, "MECHANICAL SHUTTER"=2115488, "BACK FOCUS POSITION"=8422304, "TRIGGER CONNECTOR"=1066432, "TRIGGER SOURCE"=1066144, "OUTPUT TRIGGER SOURCE"=1852576, "TRIGGER GLOBAL EXPOSURE"=2049680, "FIRST TRIGGER BEHAVIOR"=2049696, "CHANNEL SYNC"=1852352, "READOUT DIRECTION"=4211904, "PRE HSYNC COUNT"=1852704, "INTERNAL LINE SPEED"=4191408, "INTERNAL LINE INTERVAL"=4191424] ("Parameter")
        w559 = u32 1852704 items=["SENSOR MODE"=4212128, "CCD MODE"=4212384, "READOUT MODE"=4211872, "ACTIVE VIEW INDEX"=4343136, "BITS PER CHANNEL"=4342976, "IMAGE PIXEL TYPE"=4343296, "BINNING"=4215968, "EXPOSURE TIME"=2049184, "CONTRAST GAIN"=3163312, "CONTRAST OFFSET"=3163328, "LIGHT MODE"=2114720, "SENSITIVITY"=2114992, "PHOTON IMAGING MODE"=2115200, "HIGH DYNAMIC RANGE MODE"=3163360, "WHITE BALANCE"=3163568, "TEMPERATURE"=2115232, "TEMPERATURE TARGET"=2115264, "SENSOR COOLER FAN"=2115296, "LINEBUNDLE HEIGHT"=4212192, "MECHANICAL SHUTTER"=2115488, "BACK FOCUS POSITION"=8422304, "TRIGGER CONNECTOR"=1066432, "TRIGGER SOURCE"=1066144, "OUTPUT TRIGGER SOURCE"=1852576, "TRIGGER GLOBAL EXPOSURE"=2049680, "FIRST TRIGGER BEHAVIOR"=2049696, "CHANNEL SYNC"=1852352, "READOUT DIRECTION"=4211904, "PRE HSYNC COUNT"=1852704, "INTERNAL LINE SPEED"=4191408, "INTERNAL LINE INTERVAL"=4191424] ("Parameter")
        w558 = u32 4211904 items=["SENSOR MODE"=4212128, "CCD MODE"=4212384, "READOUT MODE"=4211872, "ACTIVE VIEW INDEX"=4343136, "BITS PER CHANNEL"=4342976, "IMAGE PIXEL TYPE"=4343296, "BINNING"=4215968, "EXPOSURE TIME"=2049184, "CONTRAST GAIN"=3163312, "CONTRAST OFFSET"=3163328, "LIGHT MODE"=2114720, "SENSITIVITY"=2114992, "PHOTON IMAGING MODE"=2115200, "HIGH DYNAMIC RANGE MODE"=3163360, "WHITE BALANCE"=3163568, "TEMPERATURE"=2115232, "TEMPERATURE TARGET"=2115264, "SENSOR COOLER FAN"=2115296, "LINEBUNDLE HEIGHT"=4212192, "MECHANICAL SHUTTER"=2115488, "BACK FOCUS POSITION"=8422304, "TRIGGER CONNECTOR"=1066432, "TRIGGER SOURCE"=1066144, "OUTPUT TRIGGER SOURCE"=1852576, "TRIGGER GLOBAL EXPOSURE"=2049680, "FIRST TRIGGER BEHAVIOR"=2049696, "CHANNEL SYNC"=1852352, "READOUT DIRECTION"=4211904, "PRE HSYNC COUNT"=1852704, "INTERNAL LINE SPEED"=4191408, "INTERNAL LINE INTERVAL"=4191424] ("Parameter")
        n106 = call "RS232C_Init.vi"("baud rate"=u16 9600 ("baud rate 2"), "COM Port"=refnum<visa-resource-name> "COM9" ("VISA resource name")) -> ("VISA resource name out"=w482:refnum<visa-resource-name>)  [unwired: 1 in, 2 out]
        n107 = call <userlib>:"tm_initialize_40.vi"() -> ("error out"=w549:errorcluster)  [unwired: 8 in, 3 out]
        n108 = call-poly "VISA Configure Serial Port"("timeout (10sec)"=u32 120000, "data bits (8)"=u16 8, "parity (0:none)"=enum16{"None", "Odd", "Even", "Mark", "Space"}."None", "flow control (0:none)"=w545) -> ()  [unwired: 10 in, 2 out]
        n109 = call-poly <vilib>:"DAQmx Create Virtual Channel.vi"("lines"=tag "Dev1/port0/line6") -> ("task out"=w511:refnum<k21>, "error out"=w510:errorcluster)  [unwired: 13 in]
        n110 = call <userlib>:"tm_opencamera_40.vi"("error in (no error)"=w549, "Camera Index"=u32 0) -> ("error out"=w573:errorcluster, "Handle out"=w574:u32)  [unwired: 7 in, 1 out]
        n111 = Wait (ms)(milliseconds to wait=u32 500) -> ()  [unwired: 1 out]
        n112 = call <vilib>:"DAQmx Start Task.vi"("task/channels in"=w511, "error in"=w510) -> ("task out"=w508:refnum<k21>, "error out"=w507:errorcluster)  [unwired: 12 in]
        n113 = call-poly <vilib>:"DAQmx Write.vi"("task/channels in"=w508, "data"=FALSE, "error in"=w507) -> ("task out"=w505:refnum<k21>, "error out"=w504:errorcluster)  [unwired: 10 in, 1 out]
        n114 = call <vilib>:"DAQmx Stop Task.vi"("task/channels in"=w505, "error in"=w504) -> ("task out"=w503:refnum<k21>, "error out"=w502:errorcluster)  [unwired: 12 in]
        n115 = call <vilib>:"DAQmx Clear Task.vi"("task in"=w503, "error in"=w502) -> ()  [unwired: 13 in, 1 out]
        n116 = To Double Precision Float(number=w556) -> (double precision float=w555:dbl)
        n117 = call <userlib>:"tm_setparameter_40.vi"("error in (no error)"=w573, "Value in"=12.0, "Parameter"=w560, "Handle in"=w574) -> ("error out"=w571:errorcluster, "Handle out"=w570:u32)  [unwired: 6 in]
        n118 = To Double Precision Float(number=u32 0) -> (double precision float=w552:dbl)
        n119 = call <userlib>:"tm_setparameter_40.vi"("error in (no error)"=w571, "Value in"=w552, "Parameter"=w559, "Handle in"=w570) -> ("error out"=w553:errorcluster, "Handle out"=w554:u32)  [unwired: 6 in]
        n120 = call <userlib>:"tm_setparameter_40.vi"("error in (no error)"=w553, "Value in"=w555, "Parameter"=w558, "Handle in"=w554) -> ("error out"=w562:errorcluster, "Handle out"=w561:u32)  [unwired: 6 in]
        n121 = call <userlib>:"tm_setparameter_40.vi"("error in (no error)"=w562, "Value in"=9.74436e-06, "Parameter"=w563, "Handle in"=w561) -> ("error out"=w582:errorcluster, "Handle out"=w581:u32)  [unwired: 6 in]
        n122 = flat-sequence {
          tunnel: refnum<visa-resource-name> "USB0::0x1AB1::0x0643::DG9A242400208::INSTR" ("VISA resource name") -> [w591]
          tunnel: [w589] -> w498
          tunnel: refnum<visa-resource-name> "USB0::0x1AB1::0x0643::DG9A242400205::INSTR" ("VISA resource name") -> [w588]
          tunnel: [w587] -> w495
          tunnel: w498 -> [w596]
          tunnel: [w596] -> w497
          tunnel: w495 -> [w593]
          tunnel: [w592] -> w494
          tunnel: w497 -> [w601]
          tunnel: [w601] -> w499
          tunnel: w494 -> [w599]
          tunnel: [w597] -> w491
          tunnel: w499 -> [w606]
          tunnel: [w603] -> w501
          tunnel: [w602] -> w492
          tunnel: w491 -> [w602]
          tunnel: w501 -> [w611]
          tunnel: [w608] -> w500
          tunnel: [w607] -> w493
          tunnel: w492 -> [w607]
          tunnel: w500 -> [w616]
          tunnel: [w613] -> w490
          tunnel: [w612] -> w489
          tunnel: w493 -> [w612]
          tunnel: w490 -> [w618]
          tunnel: [w617] -> w461
          tunnel: w489 -> [w621]
          tunnel: [w621] -> w459
          tunnel: w461 -> [w623]
          tunnel: [w623] -> w460
          tunnel: w459 -> [w625]
          tunnel: [w625] -> w458
          tunnel: w460 -> [w628]
          tunnel: w458 -> [w626]
          frame #0 {
            n123 = VISA Open(VISA resource name=w591) -> (VISA resource name=w589:refnum<visa-resource-name>)  [unwired: 4 in, 1 out]
            n124 = VISA Open(VISA resource name=w588) -> (VISA resource name=w587:refnum<visa-resource-name>)  [unwired: 4 in, 1 out]
            n125 = Wait (ms)(milliseconds to wait=u32 500) -> ()  [unwired: 1 out]
          }
          frame #1 {
            n126 = Wait (ms)(milliseconds to wait=u32 500) -> ()  [unwired: 1 out]
            n127 = VISA Write(VISA resource name=w593, write buffer=":OUTP2 ON") -> (VISA resource name out=w592:refnum<visa-resource-name>)  [unwired: 1 in, 2 out]
          }
          frame #2 {
            n128 = Wait (ms)(milliseconds to wait=u32 500) -> ()  [unwired: 1 out]
            n129 = VISA Write(VISA resource name=w599, write buffer=":OUTP1 ON") -> (VISA resource name out=w597:refnum<visa-resource-name>)  [unwired: 1 in, 2 out]
          }
          frame #3 {
            n130 = Wait (ms)(milliseconds to wait=u32 500) -> ()  [unwired: 1 out]
            n131 = VISA Write(VISA resource name=w606, write buffer=":OUTP2 ON") -> (VISA resource name out=w603:refnum<visa-resource-name>)  [unwired: 1 in, 2 out]
          }
          frame #4 {
            n132 = Wait (ms)(milliseconds to wait=u32 500) -> ()  [unwired: 1 out]
            n133 = VISA Write(VISA resource name=w611, write buffer=":OUTP1 ON") -> (VISA resource name out=w608:refnum<visa-resource-name>)  [unwired: 1 in, 2 out]
          }
          frame #5 {
            n134 = Wait (ms)(milliseconds to wait=u32 500) -> ()  [unwired: 1 out]
            n135 = VISA Write(VISA resource name=w616, write buffer=":TRIG1") -> (VISA resource name out=w613:refnum<visa-resource-name>)  [unwired: 1 in, 2 out]
          }
          frame #6 {
            n136 = VISA Write(VISA resource name=w618, write buffer=":TRIG2") -> (VISA resource name out=w617:refnum<visa-resource-name>)  [unwired: 1 in, 2 out]
            n137 = Wait (ms)(milliseconds to wait=u32 500) -> ()  [unwired: 1 out]
          }
          frame #7 {
            n138 = VISA Write(VISA resource name=w623, write buffer=":TRIG2") -> ()  [unwired: 1 in, 3 out]
            n139 = Wait (ms)(milliseconds to wait=u32 500) -> ()  [unwired: 1 out]
          }
          frame #8 {
            n140 = VISA Clear(VISA resource name=w626) -> ()  [unwired: 1 in, 2 out]
            n141 = VISA Clear(VISA resource name=w628) -> ()  [unwired: 1 in, 2 out]
            n142 = Wait (ms)(milliseconds to wait=u32 200) -> ()  [unwired: 1 out]
          }
        }
        n143 = call <userlib>:"tm_setparameter_40.vi"("error in (no error)"=w582, "Value in"=0.0195, "Parameter"=w583, "Handle in"=w581) -> ("error out"=w580:errorcluster, "Handle out"=w579:u32)  [unwired: 6 in]
        n144 = Bundle("Output Trigger Period"=1e-06, "Delay"=0.0, "Source"=w569) -> (w566:T6)  [unwired: 1 in]
        n145 = call <userlib>:"tm_inputtriggersource_40.vi"("error in (no error)"=w580, "External Options"=cluster{"Polarity":i32, "Delay":dbl} {"Polarity"=2, "Delay"=0.0}, "Source"=w577, "Handle in"=w579) -> ("error out"=w576:errorcluster, "Handle out"=w575:u32)  [unwired: 6 in]
        n146 = Bundle("Output Trigger Mode"=w572, "Output Trigger Polarity"=w564) -> (w565:T7)  [unwired: 1 in]
        n147 = call <userlib>:"tm_setoutputtrigger_40.vi"("Port"=0 ("Index"), "error in (no error)"=w576, "Programmable Options"=w566, "Type"=w565, "Handle in"=w575) -> ("error out"=w535:errorcluster, "Handle out"=w529:u32)  [unwired: 5 in]
        n148 = call <userlib>:"tm_getparameter_40.vi"("error in (no error)"=w535, "Parameter"=w538, "Handle in"=w529) -> ("error out"=w537:errorcluster, "Value out"=w540:dbl, "Handle out"=w528:u32)  [unwired: 6 in]
        n149 = call <userlib>:"tm_getparameter_40.vi"("error in (no error)"=w537, "Parameter"=w539, "Handle in"=w528) -> ("error out"=w536:errorcluster, "Value out"=w541:dbl)  [unwired: 6 in, 1 out]
        n150 = for {
          N: "Frames in memory 2" -> [_]
          tunnel: [w636] -> w532 mode=indexing
          tunnel: [w635] -> w534
          tunnel: w536 -> [w633]
          tunnel: w541 -> [w632]
          tunnel: w540 -> [w631]
          tunnel: [w630] -> w527 mode=indexing
          i -> [w640]
          w637 = T8 7 items=["Grayscale (U8)", "Grayscale (I16)", "Grayscale (SGL)", "Complex (CSG)", "RGB (U32)", "HSL (U32)", "RGB (U64)", "Grayscale (U16)"] ("Image Type")
          w642 = 0
          n151 = Number To Decimal String(number=w640, width (-)=i16 3) -> (decimal integer string=w641:string)
          n152 = call "IMAQ Create"("Border Size"=0, "Image Name"=w641, "Image Type"=w637, "error in (no error)"=w633) -> ("New Image"=w629:T9, "error out"=w644:errorcluster)  [unwired: 1 in]
          n153 = call "IMAQ SetImageSize"("error in (no error)"=w644, "Y Resolution"=w631, "X Resolution"=w632, "Image"=w629) -> ("error out"=w643:errorcluster, "Image Out"=w630:T9)  [unwired: 1 in]
          n154 = call "IMAQ GetImagePixelPtr"("Function"=T5."Map Pixel Pointer", "error in (no error)"=w643, "Y Coordinate"=w642, "X Coordinate"=w642, "Image"=w630) -> ("error out"=w635:errorcluster, "Pixel Pointer out"=w636:u64)  [unwired: 1 in, 4 out]
        }
        n155 = call "PortInit2.vi"() -> ("VISA resource name out"=w488:refnum<visa-resource-name>)  [unwired: 1 out]
        n156 = property class="BenchtopStepperControl"(reference="BenchtopStepperControl", "SerialNumber"="SerialNumber") -> (reference out=w479:refnum<k24>, error out=w478:errorcluster)  [unwired: 1 in]
        n157 = call <userlib>:"tm_prepare_attach_40.vi"("error in (no error)"=w534, "buffers"=w532, "Capture mode"=w531) -> ("error out"=w533:errorcluster, "Handle out"=w530:u32)  [unwired: 7 in]
        n158 = invoke class="BenchtopStepperControl" method="CreateDevice"(reference=w479, error in=w478) -> (reference out=w475:refnum<k24>, error out=w474:errorcluster)  [unwired: 1 in, 1 out]
        n159 = property class="BenchtopStepperControl"(reference=w475, error in=w474) -> (reference out=w473:refnum<k24>, "BenchtopStepperMotor"=w469)  [unwired: 1 out]
        n160 = invoke class="StepperMotorChannel" method="SetMoveAbsolutePosition"(reference=w469, "position"="position") -> (reference out=w470:refnum<k24>)  [unwired: 2 in, 3 out]
        n161 = invoke class="StepperMotorChannel" method="MoveAbsolute"(reference=w470, "waitTimeout"=1000) -> (reference out=w468:refnum<k24>)  [unwired: 2 in, 3 out]
      }
      frame "Chilling", Default {
        w667 = u8 2 items=["0", "1", "2", "3", "4"] ("Axis Number")
        n162 = call-poly <vilib>:"DAQmx Write.vi"("task/channels in"=w655, "data"="405") -> ()  [unwired: 11 in, 3 out]
        n163 = call "RS232C_SetSpeed.vi"("Low Speed"=u32 100, "High Speed"="scanning Speed", "Acceleration Time"=u16 100, "Axis Number"=w667, "Delimiter"="\r\n", "VISAリソース名"=w671, "Axis Count"=u8 2, "Range"=TRUE, "Main/Sub"=TRUE) -> ()  [unwired: 2 out]
        n164 = call-poly <vilib>:"DAQmx Write.vi"("task/channels in"=w691, "data"="532") -> ()  [unwired: 11 in, 3 out]
        n165 = call-poly <vilib>:"DAQmx Write.vi"("task/channels in"=w690, "data"="594") -> ()  [unwired: 11 in, 3 out]
        n166 = call-poly <vilib>:"DAQmx Write.vi"("task/channels in"=w693, "data"="488", "error in"=w692) -> ()  [unwired: 10 in, 3 out]
        n167 = event shown="[11] \"manual loading\": Value Change" {
          selector: _ -> [_ _ _ _ _ _ _ _ _ _ _ _]
          dyn-events: _ -> [_ _ _ _ _ _ _ _ _ _ _ _]
          timeout: _ -> [_ _ _ _ _ _ _ _ _ _ _ _]
          tunnel: [states."Stream w/o flow" states."Close" states."auto imaging" states."tube position" states."robotic arm" states."Edgehunting" states."wait for clearing" states."save" states."reverse" states."antic\n" states."405" states."manual loading"] -> w649
          event "START": Value Change {
            n168 = event-data() -> ()  [unwired: 1 in, 6 out]
            n169 = local write "READY"(FALSE ("Ready")) -> ()
            n170 = local write "Streaming"(TRUE ("Streaming")) -> ()
          }
          event "Shut down": Value Change {
            n171 = event-data() -> ()  [unwired: 1 in, 6 out]
            n172 = local write "READY"(FALSE ("Ready")) -> ()
          }
          event "START AUTO IMAGING": Value Change {
            n173 = event-data() -> ()  [unwired: 1 in, 6 out]
          }
          event "Force move": Value Change {
            n174 = event-data() -> ()  [unwired: 1 in, 6 out]
          }
          event "manual load": Value Change {
            n175 = event-data() -> ()  [unwired: 1 in, 6 out]
          }
          event "manual edgehunting": Value Change {
            n176 = event-data() -> ()  [unwired: 1 in, 6 out]
          }
          event "wait for\nclearing": Value Change {
            n177 = event-data() -> ()  [unwired: 1 in, 6 out]
          }
          event "manual imaging": Value Change {
            n178 = event-data() -> ()  [unwired: 1 in, 6 out]
          }
          event "force reverse": Value Change {
            n179 = event-data() -> ()  [unwired: 1 in, 6 out]
          }
          event "force anticlogging": Value Change {
            n180 = event-data() -> ()  [unwired: 1 in, 6 out]
          }
          event "manual 4c": Value Change {
            n181 = event-data() -> ()  [unwired: 1 in, 6 out]
          }
          event "manual loading": Value Change {
            n182 = event-data() -> ()  [unwired: 1 in, 6 out]
          }
        }
        "Streaming" <- FALSE ("Streaming")
        "READY" <- TRUE ("Ready")
        "Moving" <- FALSE ("Moving")
        "Saving image" <- FALSE ("Saving image")
      }
      frame "wait for clearing" {
        n183 = call-poly <vilib>:"DAQmx Create Virtual Channel.vi"("lines"=tag "Dev1/port2/line6") -> ("task out"=w734:refnum<k21>, "error out"=w732:errorcluster)  [unwired: 13 in]
        n184 = call <vilib>:"DAQmx Start Task.vi"("task/channels in"=w734, "error in"=w732) -> ("task out"=w731:refnum<k21>, "error out"=w727:errorcluster)  [unwired: 12 in]
        n185 = while {
          tunnel: w731 -> [w777]
          tunnel: [w776] -> w728
          tunnel: w727 -> [w775]
          tunnel: [w774] -> w726
          shift-right: [w770] -> w724
          shift-left: FALSE -> [_]
          stop <- w773 stop-if-true
          n186 = call-poly <vilib>:"DAQmx Read.vi"("task/channels in"=w777, "error in"=w775) -> ("task out"=w776:refnum<k21>, "data"=w770:bool, "error out"=w774:errorcluster)  [unwired: 11 in]
          "clear finished?" <- w770
          n187 = Or(x=w770, y="wait for clearing? 2") -> (x .or. y?=w773:bool)
          n188 = call <vilib>:"High Resolution Relative Seconds.vi"() -> ("relative seconds"=→"relative seconds 2":dbl)
        }
        n189 = call <vilib>:"DAQmx Stop Task.vi"("task/channels in"=w728, "error in"=w726) -> ("task out"=w730:refnum<k21>, "error out"=w729:errorcluster)  [unwired: 12 in]
        n190 = call <vilib>:"DAQmx Clear Task.vi"("task in"=w730, "error in"=w729) -> ()  [unwired: 13 in, 1 out]
        n191 = flat-sequence {
          tunnel: w724 -> [w769]
          tunnel: [w769] -> w723
          frame #0 {
            n192 = Wait (ms)(milliseconds to wait=u32 50) -> ()  [unwired: 1 out]
          }
        }
        n193 = case shown="False" w723 {
          tunnel: [states."Chilling" states."robotic arm"] -> w735
          frame False {
          }
          frame True {
          }
        }
      }
      frame "Stream w/o flow" {
        n194 = call <userlib>:"tm_startcapture_40.vi"("error in (no error)"=w813, "Handle in"=w812) -> ("error out"=w821:errorcluster, "Handle out"=w822:u32)  [unwired: 8 in]
        n195 = while {
          tunnel: [w830] -> w823
          tunnel: [w831] -> w824
          tunnel: w822 -> [w847]
          tunnel: w821 -> [w848]
          tunnel: w814 -> [w829]
          tunnel: [w829] -> w811
          stop <- w842 stop-if-true
          n196 = call <userlib>:"tm_waitnextframe_40.vi"("error in (no error)"=w848, "Handle in"=w847) -> ("error out"=w831:errorcluster, "Frame Count"=→"Frame count":i32, "Frame Index"=w833:i32, "Handle out"=w830:u32)  [unwired: 6 in]
          n197 = Unbundle By Name(w831) -> ("status"=w844:bool)
          n198 = Index Array(array=w829, index=w833) -> (element=w832:T9)
          n199 = Multiply(x="XS y length", y="XS x length") -> (x*y=w836:i32)
          n200 = call "IMAQ ImageToArray"("Image"=w832) -> ("Image Pixels (U16)"=w827:u16[][])  [unwired: 3 in, 4 out]
          "Obtained image" <- w827
          n201 = Build Array("Quit", w844) -> (w843:bool[])
          n202 = Or Array Elements(Boolean array=w843) -> (logical OR=w842:bool)
          n203 = Reshape Array(w827, 4194304 ("dimension size")) -> (w828:u16[])
          n204 = Array Subset(array=w827, index (row)="XS y px start", length (row)="XS y length", index (col)="XS x px start", length (col)="XS x length") -> (w839:u16[][])
          "Sub image" <- w839
          n205 = call-poly <vilib>:"Mean.vi"("X"=w828) -> ("mean"=→"Mean intensity\nof frame":dbl)  [unwired: 1 out]
          n206 = Reshape Array(w839, w836) -> (w838:u16[])
          n207 = call-poly <vilib>:"Mean.vi"("X"=w838) -> ("mean"=→"Sub img mean":dbl)  [unwired: 1 out]
        }
        n208 = call <userlib>:"tm_stopcapture_40.vi"("error in (no error)"=w824, "Handle in"=w823) -> ("error out"=w816:errorcluster, "Handle out"=w815:u32)  [unwired: 8 in]
      }
      frame "auto imaging" {
        # "abyss watcher"
        n209 = call <vilib>:"High Resolution Relative Seconds.vi"() -> ("relative seconds"=w873:dbl)
        n210 = local read "#of edgehunting"() -> (w871:u32)
        n211 = while {
          shift-right: [w1061] -> _
          shift-left: 0.0 -> [w1060]
          tunnel: [w966] -> w896
          shift-right: [w1016] -> _
          shift-left: 0.0 -> [w1016]
          tunnel: [w965] -> w883
          tunnel: w882 -> [w964]
          tunnel: [w963] -> w881
          tunnel: "Number of samples" -> [w962]
          tunnel: w874 -> [w961]
          tunnel: w873 -> [w960]
          tunnel: [w958] -> w872
          tunnel: w871 -> [w957]
          tunnel: [w954] -> w867
          shift-right: [w943] -> w855
          shift-left: w856 -> [w944]
          tunnel: [w942] -> w854
          i -> [w939]
          stop <- w1018 stop-if-true
          w1038 = 10123 items=["Finite Samples"=10178, "Continuous Samples"=10123, "Hardware Timed Single Point"=12522] ("sample mode")
          w1040 = 10106 items=["Default"=-1, "RSE"=10083, "NRSE"=10078, "Differential"=10106, "Pseudodifferential"=12529] ("input terminal configuration")
          # "V2"
          # "v2"
          n212 = call-poly <vilib>:"DAQmx Create Virtual Channel.vi"("maximum value"=5.0, "minimum value"=-5.0, "input terminal configuration"=w1040, "physical channels"="Physical Channel 2") -> ("task out"=w1035:refnum<k21>, "error out"=w1034:errorcluster)  [unwired: 10 in]
          n213 = call-poly <vilib>:"DAQmx Timing.vi"("task/channels in"=w1035, "sample mode"=w1038, "rate"=10000.0, "source"=tag "OnboardClock", "error in"=w1034) -> ("task out"=w1033:refnum<k21>, "error out"=w1032:errorcluster)  [unwired: 9 in]
          n214 = property class="DAQmx Timing"(reference=w1033, error in=w1032, "SampClk.Rate"="SampClk.Rate 2") -> (reference out=w1030:refnum<k21>, error out=w1029:errorcluster)
          n215 = call <vilib>:"DAQmx Start Task.vi"("task/channels in"=w1030, "error in"=w1029) -> ("task out"=w1028:refnum<k21>, "error out"=w1027:errorcluster)  [unwired: 12 in]
          n216 = call-poly <vilib>:"DAQmx Create Virtual Channel.vi"("lines"=tag "Dev1/port0/line5") -> ("task out"=w953:refnum<k21>)  [unwired: 13 in, 1 out]
          n217 = Increment(x=w1060) -> (x+1=w1061:dbl)
          n218 = call <vilib>:"DAQmx Start Task.vi"("task/channels in"=w953) -> ("task out"=w951:refnum<k21>)  [unwired: 13 in, 1 out]
          n219 = call-poly <vilib>:"DAQmx Create Virtual Channel.vi"("lines"=tag "Dev1/port1/line7") -> ("task out"=w1058:refnum<k21>, "error out"=w1057:errorcluster)  [unwired: 13 in]
          n220 = call-poly <vilib>:"DAQmx Create Virtual Channel.vi"("lines"=tag "Dev1/port0/line4") -> ("task out"=w1053:refnum<k21>, "error out"=w1052:errorcluster)  [unwired: 13 in]
          n221 = call-poly <vilib>:"DAQmx Create Virtual Channel.vi"("lines"=tag "Dev1/port0/line7") -> ("task out"=w998:refnum<k21>, "error out"=w1003:errorcluster)  [unwired: 13 in]
          n222 = call-poly <vilib>:"DAQmx Create Virtual Channel.vi"("lines"=tag "Dev1/port1/line6") -> ("task out"=w999:refnum<k21>, "error out"=w1002:errorcluster)  [unwired: 13 in]
          n223 = call-poly <vilib>:"DAQmx Create Virtual Channel.vi"("lines"=tag "Dev1/port1/line5") -> ("task out"=w1000:refnum<k21>, "error out"=w1001:errorcluster)  [unwired: 13 in]
          n224 = call <vilib>:"DAQmx Start Task.vi"("task/channels in"=w1053, "error in"=w1052) -> ("task out"=w1015:refnum<k21>, "error out"=w1013:errorcluster)  [unwired: 12 in]
          n225 = call <vilib>:"DAQmx Start Task.vi"("task/channels in"=w1058, "error in"=w1057) -> ("task out"=w1055:refnum<k21>, "error out"=w1054:errorcluster)  [unwired: 12 in]
          n226 = call <vilib>:"DAQmx Start Task.vi"("task/channels in"=w998, "error in"=w1003) -> ("task out"=w997:refnum<k21>, "error out"=w996:errorcluster)  [unwired: 12 in]
          n227 = call <vilib>:"DAQmx Start Task.vi"("task/channels in"=w999, "error in"=w1002) -> ("task out"=w995:refnum<k21>)  [unwired: 12 in, 1 out]
          n228 = call <vilib>:"DAQmx Start Task.vi"("task/channels in"=w1000, "error in"=w1001) -> ("task out"=w993:refnum<k21>)  [unwired: 12 in, 1 out]
          n229 = flat-sequence {
            tunnel: [w1116] -> w1067
            tunnel: w1055 -> [w1116]
            tunnel: w1054 -> [w1115]
            tunnel: [w1115] -> w1066
            tunnel: w1015 -> [w1102]
            tunnel: [w1101] -> w1014
            tunnel: w1013 -> [w1100]
            tunnel: [w1099] -> w1012
            tunnel: w997 -> [w1098]
            tunnel: w996 -> [w1096]
            tunnel: w995 -> [w1095]
            tunnel: [w1095] -> w994
            tunnel: w993 -> [w1094]
            tunnel: [w1094] -> w992
            tunnel: [w1093] -> w987
            tunnel: w951 -> [w1092]
            tunnel: [w1090] -> w950
            tunnel: w1067 -> [w1132]
            tunnel: w1066 -> [w1131]
            tunnel: [w1130] -> w1065
            tunnel: [w1129] -> w1063
            tunnel: w1014 -> [w1128]
            tunnel: w1012 -> [w1127]
            tunnel: [w1128] -> w1011
            tunnel: [w1127] -> w1010
            tunnel: w994 -> [w1126]
            tunnel: w992 -> [w1122]
            tunnel: [w1121] -> w990
            tunnel: [w1120] -> w989
            tunnel: [w1119] -> w988
            tunnel: w987 -> [w1119]
            tunnel: w950 -> [w1118]
            tunnel: [w1118] -> w949
            tunnel: w1065 -> [w1140]
            tunnel: [w1140] -> w1064
            tunnel: w1063 -> [w1139]
            tunnel: [w1139] -> w1062
            tunnel: [w1138] -> w1007
            tunnel: w1011 -> [w1138]
            tunnel: [w1137] -> _
            tunnel: w1010 -> [w1137]
            tunnel: [w1137] -> w1006
            tunnel: [w1136] -> w986
            tunnel: w990 -> [w1136]
            tunnel: w989 -> [w1135]
            tunnel: [w1134] -> w983
            tunnel: w988 -> [w1134]
            tunnel: [w1135] -> w985
            tunnel: w949 -> [w1133]
            tunnel: [w1133] -> w948
            frame #0 {
              # "7 jet pump\n6 push pump\n5 HD pump"
              n230 = Wait (ms)(milliseconds to wait=u32 50) -> ()  [unwired: 1 out]
              n231 = call-poly <vilib>:"DAQmx Write.vi"("task/channels in"=w1102, "data"=TRUE ("new element/subarray"), "error in"=w1100) -> ("task out"=w1101:refnum<k21>, "error out"=w1099:errorcluster)  [unwired: 10 in, 1 out]
              n232 = Initialize Array(FALSE, 8 ("dimension size")) -> (w1113:bool[])
              n233 = Replace Array Subset(array=w1113, new element #1=TRUE ("new element/subarray"), index #1=7 ("index"), new element #2=TRUE ("new element/subarray"), index #2=6 ("index"), new element #3=TRUE ("new element/subarray"), index #3=5 ("index"), new element #4=TRUE ("new element/subarray"), index #4=1 ("index")) -> ()  [unwired: 1 out]
              n234 = call-poly <vilib>:"DAQmx Write.vi"("task/channels in"=w1098, "data"=TRUE, "error in"=w1096) -> ("task out"=w1093:refnum<k21>)  [unwired: 10 in, 2 out]
              n235 = call-poly <vilib>:"DAQmx Write.vi"("task/channels in"=w1092, "data"=FALSE) -> ("task out"=w1090:refnum<k21>)  [unwired: 11 in, 2 out]
            }
            frame #1 {
              # "start"
              n236 = call-poly <vilib>:"DAQmx Write.vi"("task/channels in"=w1126, "data"=TRUE) -> ("task out"=w1121:refnum<k21>)  [unwired: 11 in, 2 out]
              n237 = call-poly <vilib>:"DAQmx Write.vi"("task/channels in"=w1122, "data"=TRUE) -> ("task out"=w1120:refnum<k21>)  [unwired: 11 in, 2 out]
              n238 = call-poly <vilib>:"DAQmx Write.vi"("task/channels in"=w1132, "data"=TRUE, "error in"=w1131) -> ("task out"=w1130:refnum<k21>, "error out"=w1129:errorcluster)  [unwired: 10 in, 1 out]
            }
            frame #2 {
              n239 = Wait (ms)(milliseconds to wait=u32 50) -> ()  [unwired: 1 out]
            }
          }
          n240 = flat-sequence {
            tunnel: w967 -> [w1089]
            tunnel: [w1089] -> w966
            tunnel: [w1088] -> w965
            tunnel: w964 -> [w1087]
            tunnel: [w1086] -> w963
            frame #0 {
              n241 = Tick Count (ms)() -> (millisecond timer value=w1088:u32)
              n242 = Subtract(x=w1088, y=w1087) -> (x-y=w1086:u32)
            }
          }
          n243 = call <vilib>:"High Resolution Relative Seconds.vi"() -> ("relative seconds"=w1017:dbl)
          n244 = while {
            tunnel: w1028 -> [w1195]
            tunnel: w1027 -> [w1194]
            tunnel: [w1193] -> w1024
            tunnel: [w1192] -> w1023
            shift-right: [w1191] -> _
            shift-left: w1017 -> [w1190]
            shift-right: [w1186] -> _
            shift-left: 100.0 ("relative seconds") -> [w1187]
            tunnel: w1064 -> [w1185]
            tunnel: w1062 -> [w1184]
            tunnel: [w1169] -> w1059
            tunnel: [w1185] -> w1009
            tunnel: [w1184] -> w1008
            tunnel: [w1168] -> w967
            shift-right: [w1181] -> _
            shift-left: w1016 -> [w1183]
            tunnel: w1007 -> [w1179]
            tunnel: [w1179] -> w1005
            tunnel: w1006 -> [w1178]
            tunnel: [w1178] -> w1004
            tunnel: w986 -> [w1177]
            tunnel: [w1177] -> w971
            tunnel: w985 -> [w1176]
            tunnel: [w1176] -> w970
            tunnel: w983 -> [w1175]
            tunnel: [w1175] -> w982
            tunnel: w962 -> [w1173]
            tunnel: w948 -> [w1172]
            tunnel: [w1172] -> w947
            tunnel: [w1166] -> w941
            stop <- w1167 stop-if-true
            n245 = call <vilib>:"High Resolution Relative Seconds.vi"() -> ("relative seconds"=w1191:dbl)
            n246 = call-poly <vilib>:"DAQmx Read.vi"("task/channels in"=w1195, "number of samples per channel"=w1173, "error in"=w1194) -> ("task out"=w1193:refnum<k21>, "data"=w1174:dbl[], "error out"=w1192:errorcluster)  [unwired: 10 in]
            "Waveform Graph" <- w1174
            n247 = Less?(x=w1187, y="Trigger") -> (x < y?=w1189:bool)
            n248 = Subtract(x=w1191, y=w1190) -> (x-y=w1182:dbl)
            n249 = Unbundle By Name(w1192) -> ()  [unwired: 1 out]
            n250 = case shown="True" w1189 {
              selector: w1189 -> [w1196 w1198]
              tunnel: [w1196 w1198] -> w1169
              frame False {
              }
              frame True {
                n251 = Wait (ms)(milliseconds to wait="Wait v1") -> ()  [unwired: 1 out]
              }
            }
            "Triggered" <- w1169
            n252 = Add(x=w1183, y=w1182) -> (x+y=w1181:dbl)
            "Elapsed (sec)" <- w1181
            n253 = call-poly <vilib>:"Mean.vi"("X"=w1174) -> ("mean"=w1186:dbl)  [unwired: 1 out]
            "Mean" <- w1186
            "Trigger PD running mean" <- w1186
            n254 = Greater?(x=w1181, y="reverse flow \nthreshold (sec)") -> (0:w1168:bool)
            n255 = Or(x=w1169, y="Stop Trigger stream") -> (x .or. y?=w1170:bool)
            n256 = Or(x=w1170, y=w1168) -> (x .or. y?=w1167:bool)
            n257 = call <extravilib>:"Write.vi"("element"=w1167) -> ("channel"=w1166:T10)  [unwired: 1 out]
          }
          n258 = while {
            tunnel: [w1075] -> w942
            shift-right: [w1081] -> w943
            shift-left: w944 -> [w1082]
            shift-right: [w1077] -> _
            shift-left: 0 -> [w1070]
            tunnel: w941 -> [w1072]
            i -> [w1073]
            stop <- w1074 stop-if-true
            n259 = shared-variable-read(w1082) -> (w1081:refnum<k21>, w1080:cluster{dbl, bool})  [unwired: 2 in, 2 out]
            n260 = Unbundle(w1080) -> (→"Numeric 5":dbl, w1069:bool)
            "larvae in chamber?" <- w1069
            n261 = Not(x=w1069) -> (.not. x?=w1078:bool)
            n262 = case shown="True" w1078 {
              tunnel: w1070 -> [w1083 w1085]
              tunnel: [w1083 w1084] -> w1077
              frame False {
              }
              frame True {
                n263 = Increment(x=w1085) -> (x+1=w1084:i32)
              }
            }
            n264 = Greater Or Equal?(x=w1077, y=120) -> (x >= y?=w1075:bool)
            n265 = call <extravilib>:"Read.vi"("channel"=w1072) -> ("element"=w1071:bool)  [unwired: 1 in, 1 out]
            n266 = Or(x=w1071, y=w1075) -> (x .or. y?=w1074:bool)
            "waiting number" <- w1070
            "Numeric 6" <- w1073
          }
          "triggered?" <- w942
          n267 = call <vilib>:"DAQmx Stop Task.vi"("task/channels in"=w1024, "error in"=w1023) -> ("task out"=w1026:refnum<k21>, "error out"=w1025:errorcluster)  [unwired: 12 in]
          n268 = call <vilib>:"DAQmx Clear Task.vi"("task in"=w1026, "error in"=w1025) -> ()  [unwired: 13 in, 1 out]
          n269 = call-poly <vilib>:"DAQmx Write.vi"("task/channels in"=w1005, "data"=FALSE, "error in"=w1004) -> ("task out"=w1022:refnum<k21>, "error out"=w1021:errorcluster)  [unwired: 10 in, 1 out]
          n270 = call-poly <vilib>:"DAQmx Write.vi"("task/channels in"=w982, "data"=FALSE) -> ("task out"=w978:refnum<k21>)  [unwired: 11 in, 2 out]
          n271 = while {
            tunnel: w1022 -> [w1165]
            tunnel: [w1165] -> w1048
            tunnel: w1021 -> [w1164]
            tunnel: [w1164] -> w1047
            tunnel: [w1155] -> w1044
            tunnel: [w1154] -> w1043
            tunnel: w1059 -> [w1161]
            tunnel: [w1162] -> w1019
            tunnel: w966 -> [w1158]
            tunnel: w1009 -> [w1157]
            tunnel: w1008 -> [w1156]
            tunnel: w978 -> [w1152]
            tunnel: [w1152] -> w977
            tunnel: [w1151] -> w973
            tunnel: [w1150] -> w972
            tunnel: w971 -> [w1147]
            tunnel: w970 -> [w1146]
            tunnel: [w1145] -> w959
            tunnel: w947 -> [w1144]
            tunnel: [w1142] -> w946
            stop <- w1162 stop-if-true
            n272 = call-poly <vilib>:"DAQmx Write.vi"("task/channels in"=w1157, "data"=FALSE, "error in"=w1156) -> ("task out"=w1155:refnum<k21>, "error out"=w1154:errorcluster)  [unwired: 10 in, 1 out]
            n273 = call-poly <vilib>:"DAQmx Write.vi"("task/channels in"=w1147, "data"=FALSE) -> ("task out"=w1150:refnum<k21>)  [unwired: 11 in, 2 out]
            n274 = Wait (ms)(milliseconds to wait=u32 1000) -> ()  [unwired: 1 out]
            n275 = And(x=w1161, y="next loop") -> (x .and. y?=w1159:bool)
            n276 = call-poly <vilib>:"DAQmx Write.vi"("task/channels in"=w1144, "data"=FALSE) -> ("task out"=w1142:refnum<k21>)  [unwired: 11 in, 2 out]
            n277 = call-poly <vilib>:"DAQmx Write.vi"("task/channels in"=w1146, "data"=FALSE) -> ("task out"=w1151:refnum<k21>)  [unwired: 11 in, 2 out]
            n278 = Or(x=w1159, y=w1158) -> (x .or. y?=w1162:bool)
            n279 = call <vilib>:"High Resolution Relative Seconds.vi"() -> ("relative seconds"=w1145:dbl)
          }
          n280 = Subtract(x=w959, y=w960) -> (x-y=w956:dbl)
          n281 = Greater?(x=w956, y="TIME THRESHOLD") -> (0:w954:bool)
          n282 = Insert Into Array(array=w961, index=w957, new element=w956) -> (w958:dbl[])
          n283 = call <vilib>:"DAQmx Stop Task.vi"("task/channels in"=w946) -> ("task out"=w945:refnum<k21>)  [unwired: 13 in, 1 out]
          n284 = call <vilib>:"DAQmx Stop Task.vi"("task/channels in"=w977) -> ("task out"=w976:refnum<k21>, "error out"=w979:errorcluster)  [unwired: 13 in]
          n285 = call <vilib>:"DAQmx Stop Task.vi"("task/channels in"=w972) -> ("task out"=w975:refnum<k21>, "error out"=w981:errorcluster)  [unwired: 13 in]
          n286 = Or(x=w1019, y=w966) -> (x .or. y?=w1018:bool)
          n287 = call <vilib>:"DAQmx Stop Task.vi"("task/channels in"=w1044, "error in"=w1043) -> ("task out"=w1046:refnum<k21>, "error out"=w1045:errorcluster)  [unwired: 12 in]
          n288 = call <vilib>:"DAQmx Stop Task.vi"("task/channels in"=w973) -> ("task out"=w974:refnum<k21>, "error out"=w980:errorcluster)  [unwired: 13 in]
          n289 = call <vilib>:"DAQmx Stop Task.vi"("task/channels in"=w1048, "error in"=w1047) -> ("task out"=w1050:refnum<k21>, "error out"=w1049:errorcluster)  [unwired: 12 in]
          n290 = call <vilib>:"DAQmx Clear Task.vi"("task in"=w945) -> ()  [unwired: 14 in, 1 out]
          n291 = call <vilib>:"DAQmx Clear Task.vi"("task in"=w976, "error in"=w979) -> ()  [unwired: 13 in, 1 out]
          n292 = call <vilib>:"DAQmx Clear Task.vi"("task in"=w975, "error in"=w981) -> ()  [unwired: 13 in, 1 out]
          n293 = call <vilib>:"DAQmx Clear Task.vi"("task in"=w1050, "error in"=w1049) -> ()  [unwired: 13 in, 1 out]
          n294 = call <vilib>:"DAQmx Clear Task.vi"("task in"=w1046, "error in"=w1045) -> ()  [unwired: 13 in, 1 out]
          n295 = call <vilib>:"DAQmx Clear Task.vi"("task in"=w974, "error in"=w980) -> ()  [unwired: 13 in, 1 out]
          "#triggers" <- w1060
          "Numeric 7" <- w939
        }
        n296 = case shown="True" w867 {
          tunnel: w868 -> [w908 w910]
          tunnel: [w908 w909] -> w866
          frame False {
          }
          frame True {
            n297 = Increment(x=w910) -> (x+1=w909:i32)
          }
        }
        n298 = Greater?(x=w866, y="# BEFORE GO DOWN") -> (0:w861:bool)
        n299 = local read "Continuous\nacquisition"() -> (w869:bool)
        n300 = local read "tube changing #"() -> (w863:i32)
        n301 = Less?(x=w863, y=10) -> (x < y?=w860:bool)
        n302 = And(x=w861, y=w860) -> (x .and. y?=w859:bool)
        n303 = local read "tube to stop"() -> (w851:i32)
        n304 = Greater?(x=w853, y=w851) -> (0:w852:bool)
        n305 = case shown="True" w869 {
          tunnel: [states."Edgehunting" w916] -> w906
          tunnel: w896 -> [_ w915]
          tunnel: w859 -> [_ w914]
          tunnel: w854 -> [_ w913]
          tunnel: w852 -> [_ w912]
          frame False {
          }
          frame True {
            n306 = case shown="False" w914 {
              tunnel: [w920 states."tube position"] -> w916
              tunnel: w915 -> [w919 _]
              tunnel: w913 -> [w918 _]
              tunnel: w912 -> [w917 _]
              frame False {
                n307 = case shown="True" w919 {
                  tunnel: [w923 w932] -> w920
                  tunnel: w918 -> [w922 w929]
                  tunnel: w917 -> [w921 w931]
                  frame False {
                    n308 = case shown="False" w922 {
                      tunnel: [states."Edgehunting" w926] -> w923
                      tunnel: w921 -> [_ w925]
                      frame False {
                      }
                      frame True {
                        n309 = case shown="False" w925 {
                          tunnel: [states."robotic arm" states."Chilling"] -> w926
                          frame False {
                          }
                          frame True {
                          }
                        }
                      }
                    }
                  }
                  frame True {
                    n310 = Not(x=w931) -> (.not. x?=w930:bool)
                    n311 = case shown="True" w929 {
                      tunnel: [states."reverse" w935] -> w932
                      tunnel: w930 -> [_ w934]
                      frame False {
                      }
                      frame True {
                        n312 = case shown="True" w934 {
                          tunnel: [states."Close" states."robotic arm"] -> w935
                          frame False {
                          }
                          frame True {
                          }
                        }
                      }
                    }
                  }
                }
              }
              frame True {
              }
            }
          }
        }
      }
      frame "tube position" {
        n313 = Increment(x=w1208) -> (x+1=w1207:i32)
        n314 = stacked-sequence {
          tunnel: w1206 -> [w1245 w1252]
          tunnel: FALSE ("Main/Sub") -> [w1246 w1259]
          tunnel: "tb Pulses to move" -> [_ w1256]
          tunnel: "tube Direction" -> [_ w1255]
          tunnel: "\r\n" -> [w1244 w1253]
          tunnel: [_ w1254] -> _
          tunnel: [_ w1252] -> _
          tunnel: [_ w1253] -> _
          frame #0 {
            w1249 = u8 2 items=["0", "1", "2", "3", "4"] ("Axis Number")
            n315 = call "RS232C_SetSpeed.vi"("Low Speed"=u32 100, "High Speed"=u32 2000, "Acceleration Time"=u16 100, "Axis Number"=w1249, "Delimiter"=w1244, "VISAリソース名"=w1245, "Axis Count"=u8 2, "Range"=TRUE, "Main/Sub"=w1246) -> ()  [unwired: 2 out]
          }
          frame #1 {
            w1257 = u8 1 items=["0", "1", "2", "3", "4"] ("Axis Number")
            n316 = call "RS232C_Move.vi"("VISAリソース名"=w1252, "Axis Count"=u8 2, "Axis Number"=w1257, "Pulse Number"=w1256, "Direction"=w1255, "Delimiter"=w1253, "Main/Sub"=w1259) -> ("OK Done"=w1254:bool)  [unwired: 1 out]
          }
        }
        n317 = local read "Continuous\nacquisition"() -> (w1224:bool)
        n318 = case shown="True" w1224 {
          tunnel: [states."Chilling" states."auto imaging"] -> w1225
          frame False {
          }
          frame True {
          }
        }
      }
      frame "antic\n" {
        n319 = Increment(x=w1387) -> (x+1=w1379:i32)
        n320 = local read "Continuous\nacquisition"() -> (w1384:bool)
        n321 = Greater?(x=w1379, y=u32 5) -> (0:w1383:bool)
        n322 = call-poly <vilib>:"DAQmx Create Virtual Channel.vi"("lines"=tag "Dev1/port0/line4") -> ("task out"=w1436:refnum<k21>, "error out"=w1435:errorcluster)  [unwired: 13 in]
        n323 = call-poly <vilib>:"DAQmx Create Virtual Channel.vi"("lines"=tag "Dev1/port1/line5") -> ("task out"=w1421:refnum<k21>, "error out"=w1420:errorcluster)  [unwired: 13 in]
        n324 = call-poly <vilib>:"DAQmx Create Virtual Channel.vi"("lines"=tag "Dev1/port0/line7") -> ("task out"=w1356:refnum<k21>, "error out"=w1355:errorcluster)  [unwired: 13 in]
        n325 = call <vilib>:"DAQmx Start Task.vi"("task/channels in"=w1436, "error in"=w1435) -> ("task out"=w1434:refnum<k21>, "error out"=w1433:errorcluster)  [unwired: 12 in]
        n326 = call <vilib>:"DAQmx Start Task.vi"("task/channels in"=w1421, "error in"=w1420) -> ("task out"=w1418:refnum<k21>, "error out"=w1417:errorcluster)  [unwired: 12 in]
        n327 = call <vilib>:"DAQmx Start Task.vi"("task/channels in"=w1356, "error in"=w1355) -> ("task out"=w1353:refnum<k21>, "error out"=w1352:errorcluster)  [unwired: 12 in]
        n328 = flat-sequence {
          tunnel: w1297 -> [w1459]
          tunnel: w1296 -> [w1458]
          tunnel: [w1456] -> w1351
          tunnel: [w1455] -> w1350
          tunnel: w1295 -> [w1453]
          tunnel: w1294 -> [w1452]
          tunnel: [w1450] -> w1349
          tunnel: [w1449] -> w1348
          tunnel: [w1447] -> w1347
          tunnel: [w1446] -> w1346
          tunnel: w1293 -> [w1445]
          tunnel: w1292 -> [w1444]
          tunnel: w1351 -> [w1469]
          tunnel: w1350 -> [w1468]
          tunnel: [w1467] -> w1345
          tunnel: [w1466] -> w1344
          tunnel: [w1463] -> w1343
          tunnel: w1349 -> [w1463]
          tunnel: [w1462] -> w1342
          tunnel: w1348 -> [w1462]
          tunnel: [w1461] -> w1341
          tunnel: w1347 -> [w1461]
          tunnel: [w1460] -> w1340
          tunnel: w1346 -> [w1460]
          tunnel: w1345 -> [w1479]
          tunnel: w1344 -> [w1478]
          tunnel: [w1477] -> w1339
          tunnel: [w1476] -> w1338
          tunnel: [w1474] -> w1337
          tunnel: w1343 -> [w1474]
          tunnel: [w1473] -> w1336
          tunnel: w1342 -> [w1473]
          tunnel: [w1472] -> w1335
          tunnel: w1341 -> [w1472]
          tunnel: [w1471] -> w1334
          tunnel: w1340 -> [w1471]
          tunnel: w1339 -> [w1489]
          tunnel: w1338 -> [w1488]
          tunnel: [w1487] -> w1333
          tunnel: [w1486] -> w1332
          tunnel: [w1483] -> w1331
          tunnel: w1337 -> [w1483]
          tunnel: [w1482] -> w1330
          tunnel: w1336 -> [w1482]
          tunnel: [w1481] -> w1329
          tunnel: w1335 -> [w1481]
          tunnel: [w1480] -> w1328
          tunnel: w1334 -> [w1480]
          tunnel: w1333 -> [w1499]
          tunnel: w1332 -> [w1498]
          tunnel: [w1496] -> w1327
          tunnel: [w1495] -> w1326
          tunnel: [w1493] -> w1325
          tunnel: w1331 -> [w1493]
          tunnel: [w1492] -> w1324
          tunnel: w1330 -> [w1492]
          tunnel: [w1491] -> w1323
          tunnel: w1329 -> [w1491]
          tunnel: [w1490] -> w1322
          tunnel: w1328 -> [w1490]
          tunnel: w1327 -> [w1506]
          tunnel: [w1505] -> w1321
          tunnel: w1326 -> [w1504]
          tunnel: [w1503] -> w1320
          tunnel: w1325 -> [w1509]
          tunnel: [w1509] -> w1319
          tunnel: w1324 -> [w1508]
          tunnel: [w1508] -> w1318
          tunnel: [w1501] -> w1317
          tunnel: w1323 -> [w1501]
          tunnel: [w1500] -> w1316
          tunnel: w1322 -> [w1500]
          tunnel: w1321 -> [w1514]
          tunnel: [w1513] -> w1315
          tunnel: w1320 -> [w1516]
          tunnel: [w1515] -> w1314
          tunnel: w1319 -> [w1519]
          tunnel: [w1519] -> w1313
          tunnel: w1318 -> [w1518]
          tunnel: [w1518] -> w1312
          tunnel: [w1511] -> w1311
          tunnel: w1317 -> [w1511]
          tunnel: [w1510] -> w1310
          tunnel: w1316 -> [w1510]
          tunnel: w1315 -> [w1524]
          tunnel: [w1523] -> w1309
          tunnel: w1314 -> [w1526]
          tunnel: [w1525] -> w1308
          tunnel: w1313 -> [w1529]
          tunnel: [w1529] -> w1307
          tunnel: w1312 -> [w1528]
          tunnel: [w1528] -> w1306
          tunnel: [w1521] -> w1305
          tunnel: w1311 -> [w1521]
          tunnel: [w1520] -> w1304
          tunnel: w1310 -> [w1520]
          tunnel: w1309 -> [w1536]
          tunnel: [w1533] -> w1303
          tunnel: w1308 -> [w1535]
          tunnel: [w1534] -> w1302
          tunnel: w1307 -> [w1539]
          tunnel: [w1539] -> w1301
          tunnel: w1306 -> [w1538]
          tunnel: [w1538] -> w1300
          tunnel: [w1531] -> w1299
          tunnel: w1305 -> [w1531]
          tunnel: [w1530] -> w1298
          tunnel: w1304 -> [w1530]
          tunnel: w1303 -> [w1555]
          tunnel: w1302 -> [w1545]
          tunnel: [w1553] -> w1280
          tunnel: [w1552] -> w1279
          tunnel: w1301 -> [w1550]
          tunnel: w1300 -> [w1549]
          tunnel: [w1548] -> w1282
          tunnel: [w1547] -> w1281
          tunnel: w1299 -> [w1543]
          tunnel: w1298 -> [w1542]
          tunnel: [w1541] -> w1284
          tunnel: [w1540] -> w1283
          frame #0 {
            n329 = Wait (ms)(milliseconds to wait=u32 300) -> ()  [unwired: 1 out]
            n330 = call-poly <vilib>:"DAQmx Write.vi"("task/channels in"=w1459, "data"=TRUE, "error in"=w1458) -> ("task out"=w1456:refnum<k21>, "error out"=w1455:errorcluster)  [unwired: 10 in, 1 out]
            n331 = call-poly <vilib>:"DAQmx Write.vi"("task/channels in"=w1453, "data"=TRUE, "error in"=w1452) -> ("task out"=w1450:refnum<k21>, "error out"=w1449:errorcluster)  [unwired: 10 in, 1 out]
            n332 = call-poly <vilib>:"DAQmx Write.vi"("task/channels in"=w1445, "data"=TRUE, "error in"=w1444) -> ("task out"=w1447:refnum<k21>, "error out"=w1446:errorcluster)  [unwired: 10 in, 1 out]
          }
          frame #1 {
            n333 = call-poly <vilib>:"DAQmx Write.vi"("task/channels in"=w1469, "data"=FALSE, "error in"=w1468) -> ("task out"=w1467:refnum<k21>, "error out"=w1466:errorcluster)  [unwired: 10 in, 1 out]
            n334 = Wait (ms)(milliseconds to wait=u32 300) -> ()  [unwired: 1 out]
          }
          frame #2 {
            n335 = call-poly <vilib>:"DAQmx Write.vi"("task/channels in"=w1479, "data"=TRUE, "error in"=w1478) -> ("task out"=w1477:refnum<k21>, "error out"=w1476:errorcluster)  [unwired: 10 in, 1 out]
            n336 = Wait (ms)(milliseconds to wait=u32 300) -> ()  [unwired: 1 out]
          }
          frame #3 {
            n337 = call-poly <vilib>:"DAQmx Write.vi"("task/channels in"=w1489, "data"=FALSE, "error in"=w1488) -> ("task out"=w1487:refnum<k21>, "error out"=w1486:errorcluster)  [unwired: 10 in, 1 out]
            n338 = Wait (ms)(milliseconds to wait=u32 300) -> ()  [unwired: 1 out]
          }
          frame #4 {
            n339 = call-poly <vilib>:"DAQmx Write.vi"("task/channels in"=w1499, "data"=TRUE, "error in"=w1498) -> ("task out"=w1496:refnum<k21>, "error out"=w1495:errorcluster)  [unwired: 10 in, 1 out]
            n340 = Wait (ms)(milliseconds to wait=u32 300) -> ()  [unwired: 1 out]
          }
          frame #5 {
            n341 = call-poly <vilib>:"DAQmx Write.vi"("task/channels in"=w1506, "data"=FALSE, "error in"=w1504) -> ("task out"=w1505:refnum<k21>, "error out"=w1503:errorcluster)  [unwired: 10 in, 1 out]
            n342 = Wait (ms)(milliseconds to wait=u32 300) -> ()  [unwired: 1 out]
          }
          frame #6 {
            n343 = call-poly <vilib>:"DAQmx Write.vi"("task/channels in"=w1514, "data"=TRUE, "error in"=w1516) -> ("task out"=w1513:refnum<k21>, "error out"=w1515:errorcluster)  [unwired: 10 in, 1 out]
            n344 = Wait (ms)(milliseconds to wait=u32 300) -> ()  [unwired: 1 out]
          }
          frame #7 {
            n345 = call-poly <vilib>:"DAQmx Write.vi"("task/channels in"=w1524, "data"=FALSE, "error in"=w1526) -> ("task out"=w1523:refnum<k21>, "error out"=w1525:errorcluster)  [unwired: 10 in, 1 out]
            n346 = Wait (ms)(milliseconds to wait=u32 300) -> ()  [unwired: 1 out]
          }
          frame #8 {
            n347 = call-poly <vilib>:"DAQmx Write.vi"("task/channels in"=w1536, "data"=TRUE, "error in"=w1535) -> ("task out"=w1533:refnum<k21>, "error out"=w1534:errorcluster)  [unwired: 10 in, 1 out]
            n348 = Wait (ms)(milliseconds to wait=u32 300) -> ()  [unwired: 1 out]
          }
          frame #9 {
            n349 = call-poly <vilib>:"DAQmx Write.vi"("task/channels in"=w1555, "data"=FALSE, "error in"=w1545) -> ("task out"=w1553:refnum<k21>, "error out"=w1552:errorcluster)  [unwired: 10 in, 1 out]
            n350 = call-poly <vilib>:"DAQmx Write.vi"("task/channels in"=w1550, "data"=FALSE, "error in"=w1549) -> ("task out"=w1548:refnum<k21>, "error out"=w1547:errorcluster)  [unwired: 10 in, 1 out]
            n351 = call-poly <vilib>:"DAQmx Write.vi"("task/channels in"=w1543, "data"=TRUE, "error in"=w1542) -> ("task out"=w1541:refnum<k21>, "error out"=w1540:errorcluster)  [unwired: 10 in, 1 out]
            n352 = Wait (ms)(milliseconds to wait=u32 300) -> ()  [unwired: 1 out]
          }
        }
        n353 = flat-sequence {
          tunnel: w1434 -> [w1576]
          tunnel: w1433 -> [w1575]
          tunnel: [w1573] -> w1431
          tunnel: [w1572] -> w1430
          tunnel: w1418 -> [w1570]
          tunnel: w1417 -> [w1569]
          tunnel: [w1567] -> w1413
          tunnel: [w1566] -> w1409
          tunnel: [w1564] -> w1366
          tunnel: [w1563] -> w1357
          tunnel: w1353 -> [w1562]
          tunnel: w1352 -> [w1561]
          tunnel: w1431 -> [w1586]
          tunnel: w1430 -> [w1585]
          tunnel: [w1584] -> w1429
          tunnel: [w1583] -> w1428
          tunnel: [w1580] -> w1414
          tunnel: w1413 -> [w1580]
          tunnel: [w1579] -> w1410
          tunnel: w1409 -> [w1579]
          tunnel: [w1578] -> w1367
          tunnel: w1366 -> [w1578]
          tunnel: [w1577] -> w1358
          tunnel: w1357 -> [w1577]
          tunnel: w1429 -> [w1596]
          tunnel: w1428 -> [w1595]
          tunnel: [w1594] -> w1427
          tunnel: [w1593] -> w1426
          tunnel: [w1590] -> w1415
          tunnel: w1414 -> [w1590]
          tunnel: [w1589] -> w1411
          tunnel: w1410 -> [w1589]
          tunnel: [w1588] -> w1368
          tunnel: w1367 -> [w1588]
          tunnel: [w1587] -> w1359
          tunnel: w1358 -> [w1587]
          tunnel: w1427 -> [w1606]
          tunnel: w1426 -> [w1605]
          tunnel: [w1604] -> w1425
          tunnel: [w1603] -> w1424
          tunnel: [w1600] -> w1416
          tunnel: w1415 -> [w1600]
          tunnel: [w1599] -> w1412
          tunnel: w1411 -> [w1599]
          tunnel: [w1598] -> w1369
          tunnel: w1368 -> [w1598]
          tunnel: [w1597] -> w1360
          tunnel: w1359 -> [w1597]
          tunnel: w1425 -> [w1616]
          tunnel: w1424 -> [w1615]
          tunnel: [w1613] -> w1408
          tunnel: [w1612] -> w1407
          tunnel: [w1610] -> w1406
          tunnel: w1416 -> [w1610]
          tunnel: [w1609] -> w1405
          tunnel: w1412 -> [w1609]
          tunnel: [w1608] -> w1370
          tunnel: w1369 -> [w1608]
          tunnel: [w1607] -> w1361
          tunnel: w1360 -> [w1607]
          tunnel: w1408 -> [w1623]
          tunnel: [w1622] -> w1404
          tunnel: w1407 -> [w1621]
          tunnel: [w1620] -> w1403
          tunnel: w1406 -> [w1626]
          tunnel: [w1626] -> w1402
          tunnel: w1405 -> [w1625]
          tunnel: [w1625] -> w1401
          tunnel: [w1618] -> w1371
          tunnel: w1370 -> [w1618]
          tunnel: [w1617] -> w1362
          tunnel: w1361 -> [w1617]
          tunnel: w1404 -> [w1631]
          tunnel: [w1630] -> w1400
          tunnel: w1403 -> [w1633]
          tunnel: [w1632] -> w1399
          tunnel: w1402 -> [w1636]
          tunnel: [w1636] -> w1398
          tunnel: w1401 -> [w1635]
          tunnel: [w1635] -> w1397
          tunnel: [w1628] -> w1372
          tunnel: w1371 -> [w1628]
          tunnel: [w1627] -> w1363
          tunnel: w1362 -> [w1627]
          tunnel: w1400 -> [w1641]
          tunnel: [w1640] -> w1396
          tunnel: w1399 -> [w1643]
          tunnel: [w1642] -> w1394
          tunnel: w1398 -> [w1646]
          tunnel: [w1646] -> w1392
          tunnel: w1397 -> [w1645]
          tunnel: [w1645] -> w1390
          tunnel: [w1638] -> w1373
          tunnel: w1372 -> [w1638]
          tunnel: [w1637] -> w1364
          tunnel: w1363 -> [w1637]
          tunnel: w1396 -> [w1653]
          tunnel: [w1650] -> w1395
          tunnel: w1394 -> [w1652]
          tunnel: [w1651] -> w1393
          tunnel: w1392 -> [w1656]
          tunnel: [w1656] -> w1391
          tunnel: w1390 -> [w1655]
          tunnel: [w1655] -> w1389
          tunnel: [w1648] -> w1374
          tunnel: w1373 -> [w1648]
          tunnel: [w1647] -> w1365
          tunnel: w1364 -> [w1647]
          tunnel: w1395 -> [w1672]
          tunnel: w1393 -> [w1662]
          tunnel: [w1670] -> w1297
          tunnel: [w1669] -> w1296
          tunnel: w1391 -> [w1667]
          tunnel: w1389 -> [w1666]
          tunnel: [w1665] -> w1295
          tunnel: [w1664] -> w1294
          tunnel: w1374 -> [w1660]
          tunnel: w1365 -> [w1659]
          tunnel: [w1658] -> w1293
          tunnel: [w1657] -> w1292
          frame #0 {
            n354 = call-poly <vilib>:"DAQmx Write.vi"("task/channels in"=w1576, "data"=TRUE, "error in"=w1575) -> ("task out"=w1573:refnum<k21>, "error out"=w1572:errorcluster)  [unwired: 10 in, 1 out]
            n355 = call-poly <vilib>:"DAQmx Write.vi"("task/channels in"=w1570, "data"=TRUE, "error in"=w1569) -> ("task out"=w1567:refnum<k21>, "error out"=w1566:errorcluster)  [unwired: 10 in, 1 out]
            n356 = call-poly <vilib>:"DAQmx Write.vi"("task/channels in"=w1562, "data"=TRUE, "error in"=w1561) -> ("task out"=w1564:refnum<k21>, "error out"=w1563:errorcluster)  [unwired: 10 in, 1 out]
            n357 = Wait (ms)(milliseconds to wait=u32 300) -> ()  [unwired: 1 out]
          }
          frame #1 {
            n358 = call-poly <vilib>:"DAQmx Write.vi"("task/channels in"=w1586, "data"=FALSE, "error in"=w1585) -> ("task out"=w1584:refnum<k21>, "error out"=w1583:errorcluster)  [unwired: 10 in, 1 out]
            n359 = Wait (ms)(milliseconds to wait=u32 300) -> ()  [unwired: 1 out]
          }
          frame #2 {
            n360 = call-poly <vilib>:"DAQmx Write.vi"("task/channels in"=w1596, "data"=TRUE, "error in"=w1595) -> ("task out"=w1594:refnum<k21>, "error out"=w1593:errorcluster)  [unwired: 10 in, 1 out]
            n361 = Wait (ms)(milliseconds to wait=u32 300) -> ()  [unwired: 1 out]
          }
          frame #3 {
            n362 = call-poly <vilib>:"DAQmx Write.vi"("task/channels in"=w1606, "data"=FALSE, "error in"=w1605) -> ("task out"=w1604:refnum<k21>, "error out"=w1603:errorcluster)  [unwired: 10 in, 1 out]
            n363 = Wait (ms)(milliseconds to wait=u32 300) -> ()  [unwired: 1 out]
          }
          frame #4 {
            n364 = call-poly <vilib>:"DAQmx Write.vi"("task/channels in"=w1616, "data"=TRUE, "error in"=w1615) -> ("task out"=w1613:refnum<k21>, "error out"=w1612:errorcluster)  [unwired: 10 in, 1 out]
            n365 = Wait (ms)(milliseconds to wait=u32 300) -> ()  [unwired: 1 out]
          }
          frame #5 {
            n366 = Wait (ms)(milliseconds to wait=u32 300) -> ()  [unwired: 1 out]
            n367 = call-poly <vilib>:"DAQmx Write.vi"("task/channels in"=w1623, "data"=FALSE, "error in"=w1621) -> ("task out"=w1622:refnum<k21>, "error out"=w1620:errorcluster)  [unwired: 10 in, 1 out]
          }
          frame #6 {
            n368 = Wait (ms)(milliseconds to wait=u32 300) -> ()  [unwired: 1 out]
            n369 = call-poly <vilib>:"DAQmx Write.vi"("task/channels in"=w1631, "data"=TRUE, "error in"=w1633) -> ("task out"=w1630:refnum<k21>, "error out"=w1632:errorcluster)  [unwired: 10 in, 1 out]
          }
          frame #7 {
            n370 = call-poly <vilib>:"DAQmx Write.vi"("task/channels in"=w1641, "data"=FALSE, "error in"=w1643) -> ("task out"=w1640:refnum<k21>, "error out"=w1642:errorcluster)  [unwired: 10 in, 1 out]
            n371 = Wait (ms)(milliseconds to wait=u32 300) -> ()  [unwired: 1 out]
          }
          frame #8 {
            n372 = call-poly <vilib>:"DAQmx Write.vi"("task/channels in"=w1653, "data"=TRUE, "error in"=w1652) -> ("task out"=w1650:refnum<k21>, "error out"=w1651:errorcluster)  [unwired: 10 in, 1 out]
            n373 = Wait (ms)(milliseconds to wait=u32 300) -> ()  [unwired: 1 out]
          }
          frame #9 {
            n374 = call-poly <vilib>:"DAQmx Write.vi"("task/channels in"=w1672, "data"=TRUE, "error in"=w1662) -> ("task out"=w1670:refnum<k21>, "error out"=w1669:errorcluster)  [unwired: 10 in, 1 out]
            n375 = call-poly <vilib>:"DAQmx Write.vi"("task/channels in"=w1667, "data"=FALSE, "error in"=w1666) -> ("task out"=w1665:refnum<k21>, "error out"=w1664:errorcluster)  [unwired: 10 in, 1 out]
            n376 = call-poly <vilib>:"DAQmx Write.vi"("task/channels in"=w1660, "data"=TRUE, "error in"=w1659) -> ("task out"=w1658:refnum<k21>, "error out"=w1657:errorcluster)  [unwired: 10 in, 1 out]
            n377 = Wait (ms)(milliseconds to wait=u32 300) -> ()  [unwired: 1 out]
          }
        }
        n378 = call <vilib>:"DAQmx Stop Task.vi"("task/channels in"=w1282, "error in"=w1281) -> ("task out"=w1288:refnum<k21>, "error out"=w1287:errorcluster)  [unwired: 12 in]
        n379 = call <vilib>:"DAQmx Stop Task.vi"("task/channels in"=w1284, "error in"=w1283) -> ("task out"=w1286:refnum<k21>, "error out"=w1285:errorcluster)  [unwired: 12 in]
        n380 = call <vilib>:"DAQmx Stop Task.vi"("task/channels in"=w1280, "error in"=w1279) -> ("task out"=w1290:refnum<k21>, "error out"=w1289:errorcluster)  [unwired: 12 in]
        n381 = call <vilib>:"DAQmx Clear Task.vi"("task in"=w1288, "error in"=w1287) -> ()  [unwired: 13 in, 1 out]
        n382 = call <vilib>:"DAQmx Clear Task.vi"("task in"=w1286, "error in"=w1285) -> ()  [unwired: 13 in, 1 out]
        n383 = call <vilib>:"DAQmx Clear Task.vi"("task in"=w1290, "error in"=w1289) -> ()  [unwired: 13 in, 1 out]
        n384 = case shown="False" w1384 {
          tunnel: [states."Chilling" w1558] -> w1423
          tunnel: w1383 -> [_ w1557]
          frame False {
          }
          frame True {
            n385 = case shown="False" w1557 {
              tunnel: [states."auto imaging" states."Close"] -> w1558
              frame False {
              }
              frame True {
              }
            }
          }
        }
      }
      frame "reverse" {
        # "valve 3"
        # "pinch valve v2"
        # "pinch valve1"
        # "shower valve3"
        n386 = call-poly <vilib>:"DAQmx Create Virtual Channel.vi"("lines"=tag "Dev1/port0/line5") -> ("task out"=w1697:refnum<k21>)  [unwired: 13 in, 1 out]
        n387 = call-poly <vilib>:"DAQmx Create Virtual Channel.vi"("lines"=tag "Dev1/port0/line4") -> ("task out"=w1694:refnum<k21>)  [unwired: 13 in, 1 out]
        n388 = call-poly <vilib>:"DAQmx Create Virtual Channel.vi"("lines"=tag "Dev1/port0/line7") -> ("task out"=w1720:refnum<k21>, "error out"=w1721:errorcluster)  [unwired: 13 in]
        n389 = flat-sequence {
          tunnel: "milliseconds to wait" -> [w1762]
          tunnel: "Flow Rate (5.00)" -> [w1763]
          tunnel: [w1763] -> w1713
          tunnel: [w1762] -> w1711
          tunnel: w1685 -> [w1761]
          tunnel: [w1761] -> w1684
          tunnel: w1713 -> [w1768]
          tunnel: [w1768] -> w1712
          tunnel: w1711 -> [w1767]
          tunnel: [w1767] -> w1710
          tunnel: w1684 -> [w1765]
          tunnel: [w1764] -> w1683
          tunnel: w1712 -> [w1774]
          tunnel: w1710 -> [w1773]
          tunnel: [w1774] -> w1709
          tunnel: [w1774] -> w1707
          tunnel: [w1773] -> w1705
          tunnel: w1683 -> [w1772]
          tunnel: [w1770] -> w1682
          tunnel: w1709 -> [w1780]
          tunnel: [w1780] -> w1708
          tunnel: w1707 -> [w1779]
          tunnel: [w1779] -> w1706
          tunnel: w1705 -> [w1778]
          tunnel: [w1778] -> w1704
          tunnel: w1682 -> [w1777]
          tunnel: [w1775] -> w1681
          tunnel: w1708 -> [_]
          tunnel: [w1786] -> w1703
          tunnel: w1706 -> [w1786]
          tunnel: w1704 -> [w1785]
          tunnel: [w1785] -> w1701
          tunnel: w1681 -> [w1784]
          tunnel: [w1782] -> w1680
          tunnel: w1703 -> [w1791]
          tunnel: [w1791] -> w1702
          tunnel: w1701 -> [w1790]
          tunnel: [w1790] -> w1700
          tunnel: w1680 -> [w1789]
          tunnel: [w1787] -> w1679
          tunnel: w1702 -> [_]
          tunnel: w1700 -> [_]
          tunnel: w1679 -> [w1795]
          tunnel: [w1793] -> w1678
          tunnel: w1724 -> [w1805]
          tunnel: [w1803] -> w1723
          tunnel: w1716 -> [w1801]
          tunnel: [w1800] -> w1714
          tunnel: [w1799] -> w1689
          tunnel: w1688 -> [w1797]
          tunnel: w1678 -> [w1796]
          tunnel: [w1796] -> w1677
          frame #0 {
            (unwired) FALSE ("Boolean")
            n390 = Wait (ms)(milliseconds to wait=u32 1000) -> ()  [unwired: 1 out]
          }
          frame #1 {
            n391 = call-poly <vilib>:"DAQmx Write.vi"("task/channels in"=w1765, "data"=TRUE) -> ("task out"=w1764:refnum<k21>)  [unwired: 11 in, 2 out]
            n392 = Wait (ms)(milliseconds to wait=w1767) -> ()  [unwired: 1 out]
          }
          frame #2 {
            n393 = call-poly <vilib>:"DAQmx Write.vi"("task/channels in"=w1772, "data"=FALSE) -> ("task out"=w1770:refnum<k21>)  [unwired: 11 in, 2 out]
            n394 = Wait (ms)(milliseconds to wait=u32 500) -> ()  [unwired: 1 out]
          }
          frame #3 {
            (unwired) FALSE ("Boolean")
            n395 = call-poly <vilib>:"DAQmx Write.vi"("task/channels in"=w1777, "data"=TRUE) -> ("task out"=w1775:refnum<k21>)  [unwired: 11 in, 2 out]
          }
          frame #4 {
            n396 = call-poly <vilib>:"DAQmx Write.vi"("task/channels in"=w1784, "data"=FALSE) -> ("task out"=w1782:refnum<k21>)  [unwired: 11 in, 2 out]
            n397 = Wait (ms)(milliseconds to wait=u32 500) -> ()  [unwired: 1 out]
          }
          frame #5 {
            n398 = call-poly <vilib>:"DAQmx Write.vi"("task/channels in"=w1789, "data"=TRUE ("Boolean")) -> ("task out"=w1787:refnum<k21>)  [unwired: 11 in, 2 out]
            n399 = Wait (ms)(milliseconds to wait=w1790) -> ()  [unwired: 1 out]
          }
          frame #6 {
            n400 = call-poly <vilib>:"DAQmx Write.vi"("task/channels in"=w1795, "data"=FALSE) -> ("task out"=w1793:refnum<k21>)  [unwired: 11 in, 2 out]
            n401 = Wait (ms)(milliseconds to wait=u32 500) -> ()  [unwired: 1 out]
          }
          frame #7 {
            n402 = call-poly <vilib>:"DAQmx Write.vi"("task/channels in"=w1801, "data"=FALSE) -> ("task out"=w1800:refnum<k21>)  [unwired: 11 in, 2 out]
            n403 = call-poly <vilib>:"DAQmx Write.vi"("task/channels in"=w1805, "data"=FALSE) -> ("task out"=w1803:refnum<k21>)  [unwired: 11 in, 2 out]
            n404 = call-poly <vilib>:"DAQmx Write.vi"("task/channels in"=w1797, "data"=FALSE) -> ("task out"=w1799:refnum<k21>)  [unwired: 11 in, 2 out]
          }
        }
        n405 = call <vilib>:"DAQmx Start Task.vi"("task/channels in"=w1697) -> ("task out"=w1685:refnum<k21>)  [unwired: 13 in, 1 out]
        n406 = call-poly <vilib>:"DAQmx Write.vi"("task/channels in"=w1726, "data"=TRUE) -> ("task out"=w1724:refnum<k21>)  [unwired: 11 in, 2 out]
        n407 = call <vilib>:"DAQmx Start Task.vi"("task/channels in"=w1694) -> ("task out"=w1691:refnum<k21>)  [unwired: 13 in, 1 out]
        n408 = call <vilib>:"DAQmx Start Task.vi"("task/channels in"=w1720, "error in"=w1721) -> ("task out"=w1717:refnum<k21>)  [unwired: 12 in, 1 out]
        n409 = call-poly <vilib>:"DAQmx Write.vi"("task/channels in"=w1717, "data"=TRUE) -> ("task out"=w1716:refnum<k21>)  [unwired: 11 in, 2 out]
        n410 = call-poly <vilib>:"DAQmx Write.vi"("task/channels in"=w1691, "data"=TRUE) -> ("task out"=w1688:refnum<k21>)  [unwired: 11 in, 2 out]
        n411 = call <vilib>:"DAQmx Stop Task.vi"("task/channels in"=w1714) -> ("task out"=w1715:refnum<k21>)  [unwired: 13 in, 1 out]
        n412 = call <vilib>:"DAQmx Stop Task.vi"("task/channels in"=w1677) -> ("task out"=w1695:refnum<k21>)  [unwired: 13 in, 1 out]
        n413 = call <vilib>:"DAQmx Stop Task.vi"("task/channels in"=w1689) -> ("task out"=w1692:refnum<k21>)  [unwired: 13 in, 1 out]
        n414 = call <vilib>:"DAQmx Clear Task.vi"("task in"=w1715) -> ()  [unwired: 14 in, 1 out]
        n415 = call <vilib>:"DAQmx Clear Task.vi"("task in"=w1695) -> ()  [unwired: 14 in, 1 out]
        n416 = call <vilib>:"DAQmx Clear Task.vi"("task in"=w1692) -> ()  [unwired: 14 in, 1 out]
        n417 = local read "Continuous\nacquisition"() -> (w1722:bool)
        n418 = case shown="True" w1722 {
          tunnel: [states."Chilling" states."antic\n"] -> w1729
          frame False {
          }
          frame True {
          }
        }
      }
      frame "light reverse" {
        (unwired) FALSE ("data")
        # "valve 3"
        # "pinch valve v2"
        # "pinch valve1"
        # "shower valve3"
        n419 = call-poly <vilib>:"DAQmx Create Virtual Channel.vi"("lines"=tag "Dev1/port0/line5") -> ("task out"=w1831:refnum<k21>)  [unwired: 13 in, 1 out]
        n420 = call-poly <vilib>:"DAQmx Create Virtual Channel.vi"("lines"=tag "Dev1/port0/line4") -> ("task out"=w1828:refnum<k21>)  [unwired: 13 in, 1 out]
        n421 = call-poly <vilib>:"DAQmx Create Virtual Channel.vi"("lines"=tag "Dev1/port0/line7") -> ("task out"=w1846:refnum<k21>, "error out"=w1847:errorcluster)  [unwired: 13 in]
        n422 = flat-sequence {
          tunnel: u32 1000 ("milliseconds to wait 2") -> [w1886]
          tunnel: [w1886] -> w1839
          tunnel: w1819 -> [w1885]
          tunnel: [w1885] -> w1818
          tunnel: w1839 -> [w1890]
          tunnel: [w1890] -> w1838
          tunnel: w1818 -> [w1888]
          tunnel: [w1887] -> w1817
          tunnel: w1838 -> [w1895]
          tunnel: [w1895] -> w1837
          tunnel: w1817 -> [w1894]
          tunnel: [w1892] -> w1816
          tunnel: w1837 -> [w1899]
          tunnel: [w1899] -> w1836
          tunnel: w1816 -> [w1898]
          tunnel: [w1896] -> w1815
          tunnel: w1836 -> [w1904]
          tunnel: [w1904] -> w1835
          tunnel: w1815 -> [w1903]
          tunnel: [w1901] -> w1814
          tunnel: w1835 -> [w1908]
          tunnel: [w1908] -> w1834
          tunnel: w1814 -> [w1907]
          tunnel: [w1905] -> w1813
          tunnel: w1834 -> [_]
          tunnel: w1813 -> [w1912]
          tunnel: [w1910] -> w1812
          tunnel: w1850 -> [w1922]
          tunnel: [w1920] -> w1849
          tunnel: w1842 -> [w1918]
          tunnel: [w1917] -> w1840
          tunnel: [w1916] -> w1823
          tunnel: w1822 -> [w1914]
          tunnel: w1812 -> [w1913]
          tunnel: [w1913] -> w1811
          frame #0 {
            (unwired) FALSE ("Boolean")
            n423 = Wait (ms)(milliseconds to wait=u32 1000) -> ()  [unwired: 1 out]
          }
          frame #1 {
            n424 = call-poly <vilib>:"DAQmx Write.vi"("task/channels in"=w1888, "data"=TRUE) -> ("task out"=w1887:refnum<k21>)  [unwired: 11 in, 2 out]
            n425 = Wait (ms)(milliseconds to wait=w1890) -> ()  [unwired: 1 out]
          }
          frame #2 {
            n426 = call-poly <vilib>:"DAQmx Write.vi"("task/channels in"=w1894, "data"=FALSE) -> ("task out"=w1892:refnum<k21>)  [unwired: 11 in, 2 out]
            n427 = Wait (ms)(milliseconds to wait=u32 500) -> ()  [unwired: 1 out]
          }
          frame #3 {
            (unwired) FALSE ("Boolean")
            n428 = call-poly <vilib>:"DAQmx Write.vi"("task/channels in"=w1898, "data"=TRUE) -> ("task out"=w1896:refnum<k21>)  [unwired: 11 in, 2 out]
          }
          frame #4 {
            n429 = call-poly <vilib>:"DAQmx Write.vi"("task/channels in"=w1903, "data"=FALSE) -> ("task out"=w1901:refnum<k21>)  [unwired: 11 in, 2 out]
            n430 = Wait (ms)(milliseconds to wait=u32 500) -> ()  [unwired: 1 out]
          }
          frame #5 {
            n431 = call-poly <vilib>:"DAQmx Write.vi"("task/channels in"=w1907, "data"=TRUE ("Boolean")) -> ("task out"=w1905:refnum<k21>)  [unwired: 11 in, 2 out]
            n432 = Wait (ms)(milliseconds to wait=w1908) -> ()  [unwired: 1 out]
          }
          frame #6 {
            n433 = call-poly <vilib>:"DAQmx Write.vi"("task/channels in"=w1912, "data"=FALSE) -> ("task out"=w1910:refnum<k21>)  [unwired: 11 in, 2 out]
            n434 = Wait (ms)(milliseconds to wait=u32 500) -> ()  [unwired: 1 out]
          }
          frame #7 {
            n435 = call-poly <vilib>:"DAQmx Write.vi"("task/channels in"=w1918, "data"=FALSE) -> ("task out"=w1917:refnum<k21>)  [unwired: 11 in, 2 out]
            n436 = call-poly <vilib>:"DAQmx Write.vi"("task/channels in"=w1922, "data"=FALSE) -> ("task out"=w1920:refnum<k21>)  [unwired: 11 in, 2 out]
            n437 = call-poly <vilib>:"DAQmx Write.vi"("task/channels in"=w1914, "data"=FALSE) -> ("task out"=w1916:refnum<k21>)  [unwired: 11 in, 2 out]
          }
        }
        n438 = call <vilib>:"DAQmx Start Task.vi"("task/channels in"=w1831) -> ("task out"=w1819:refnum<k21>)  [unwired: 13 in, 1 out]
        n439 = call-poly <vilib>:"DAQmx Write.vi"("task/channels in"=w1852, "data"=TRUE) -> ("task out"=w1850:refnum<k21>)  [unwired: 11 in, 2 out]
        n440 = call <vilib>:"DAQmx Start Task.vi"("task/channels in"=w1828) -> ("task out"=w1825:refnum<k21>)  [unwired: 13 in, 1 out]
        n441 = call <vilib>:"DAQmx Start Task.vi"("task/channels in"=w1846, "error in"=w1847) -> ("task out"=w1843:refnum<k21>)  [unwired: 12 in, 1 out]
        n442 = call-poly <vilib>:"DAQmx Write.vi"("task/channels in"=w1843, "data"=TRUE) -> ("task out"=w1842:refnum<k21>)  [unwired: 11 in, 2 out]
        n443 = call-poly <vilib>:"DAQmx Write.vi"("task/channels in"=w1825, "data"=TRUE) -> ("task out"=w1822:refnum<k21>)  [unwired: 11 in, 2 out]
        n444 = call <vilib>:"DAQmx Stop Task.vi"("task/channels in"=w1840) -> ("task out"=w1841:refnum<k21>)  [unwired: 13 in, 1 out]
        n445 = call <vilib>:"DAQmx Stop Task.vi"("task/channels in"=w1811) -> ("task out"=w1829:refnum<k21>)  [unwired: 13 in, 1 out]
        n446 = call <vilib>:"DAQmx Stop Task.vi"("task/channels in"=w1823) -> ("task out"=w1826:refnum<k21>)  [unwired: 13 in, 1 out]
        n447 = call <vilib>:"DAQmx Clear Task.vi"("task in"=w1841) -> ()  [unwired: 14 in, 1 out]
        n448 = call <vilib>:"DAQmx Clear Task.vi"("task in"=w1829) -> ()  [unwired: 14 in, 1 out]
        n449 = call <vilib>:"DAQmx Clear Task.vi"("task in"=w1826) -> ()  [unwired: 14 in, 1 out]
        n450 = local read "Continuous\nacquisition"() -> (w1848:bool)
        n451 = case shown="False" w1848 {
          tunnel: [states."Chilling" states."auto imaging"] -> w1853
          frame False {
          }
          frame True {
          }
        }
      }
      frame "robotic arm" {
        # "1+2+10+"
        # "shower flow"
        # "shower valve high"
        # "shower valve low:"
        # "robotic arm signal"
        n452 = Increment(x=w2053) -> (x+1=w1927:i32)
        "loading tube#" <- w1927
        n453 = local read "tb Pulses to move"() -> (w2012:u32)
        n454 = local read "tube changing #"() -> (w2011:i32)
        n455 = local read "tube Direction"() -> (w2014:bool)
        n456 = Multiply(x=w2012, y=w2011) -> (x*y=w2010:u32)
        n457 = Not(x=w2014) -> (.not. x?=w2013:bool)
        n458 = stacked-sequence {
          tunnel: w2009 -> [w2127 w2134]
          tunnel: FALSE ("Main/Sub") -> [w2128 w2141]
          tunnel: w2010 -> [_ w2138]
          tunnel: w2013 -> [_ w2137]
          tunnel: "\r\n" -> [w2126 w2135]
          tunnel: [_ w2136] -> _
          tunnel: [_ w2134] -> _
          tunnel: [_ w2135] -> _
          frame #0 {
            w2131 = u8 2 items=["0", "1", "2", "3", "4"] ("Axis Number")
            n459 = call "RS232C_SetSpeed.vi"("Low Speed"=u32 100, "High Speed"=u32 2000, "Acceleration Time"=u16 100, "Axis Number"=w2131, "Delimiter"=w2126, "VISAリソース名"=w2127, "Axis Count"=u8 2, "Range"=TRUE, "Main/Sub"=w2128) -> ()  [unwired: 2 out]
          }
          frame #1 {
            w2139 = u8 1 items=["0", "1", "2", "3", "4"] ("Axis Number")
            n460 = call "RS232C_Move.vi"("VISAリソース名"=w2134, "Axis Count"=u8 2, "Axis Number"=w2139, "Pulse Number"=w2138, "Direction"=w2137, "Delimiter"=w2135, "Main/Sub"=w2141) -> ("OK Done"=w2136:bool)  [unwired: 1 out]
          }
        }
        n461 = local write "Larvae until move"(0 ("Larva # to move")) -> ()
        n462 = call-poly <vilib>:"DAQmx Create Virtual Channel.vi"("lines"=tag "Dev1/port1/line4") -> ("task out"=w2084:refnum<k21>, "error out"=w2083:errorcluster)  [unwired: 13 in]
        n463 = call-poly <vilib>:"DAQmx Create Virtual Channel.vi"("lines"=tag "Dev1/port1/line3") -> ("task out"=w2082:refnum<k21>, "error out"=w2081:errorcluster)  [unwired: 13 in]
        n464 = call-poly <vilib>:"DAQmx Create Virtual Channel.vi"("lines"=tag "Dev1/port1/line0") -> ("task out"=w2099:refnum<k21>, "error out"=w2098:errorcluster)  [unwired: 13 in]
        n465 = call <vilib>:"DAQmx Start Task.vi"("task/channels in"=w2084, "error in"=w2083) -> ("task out"=w2079:refnum<k21>, "error out"=w2071:errorcluster)  [unwired: 12 in]
        n466 = call <vilib>:"DAQmx Start Task.vi"("task/channels in"=w2082, "error in"=w2081) -> ("task out"=w2075:refnum<k21>, "error out"=w2067:errorcluster)  [unwired: 12 in]
        n467 = call <vilib>:"DAQmx Start Task.vi"("task/channels in"=w2099, "error in"=w2098) -> ("task out"=w2096:refnum<k21>, "error out"=w2095:errorcluster)  [unwired: 12 in]
        n468 = flat-sequence {
          tunnel: w2096 -> [w2152]
          tunnel: w2095 -> [w2151]
          tunnel: [w2149] -> w2094
          tunnel: [w2148] -> w2093
          tunnel: [w2147] -> w2080
          tunnel: w2079 -> [w2147]
          tunnel: [w2146] -> w2076
          tunnel: w2075 -> [w2146]
          tunnel: [w2145] -> w2072
          tunnel: w2071 -> [w2145]
          tunnel: [w2144] -> w2068
          tunnel: w2067 -> [w2144]
          tunnel: [w2142] -> w2045
          tunnel: w2042 -> [w2142]
          tunnel: w2094 -> [w2162]
          tunnel: w2093 -> [w2161]
          tunnel: [w2159] -> w2091
          tunnel: [w2158] -> w2089
          tunnel: w2080 -> [w2157]
          tunnel: [w2157] -> w2077
          tunnel: w2076 -> [w2156]
          tunnel: [w2156] -> w2074
          tunnel: w2072 -> [w2155]
          tunnel: [w2155] -> w2069
          tunnel: w2068 -> [w2154]
          tunnel: [w2154] -> w2065
          tunnel: w2045 -> [w2153]
          tunnel: [w2153] -> w2043
          tunnel: [w2170] -> w2092
          tunnel: w2091 -> [w2170]
          tunnel: [w2169] -> w2090
          tunnel: w2089 -> [w2169]
          tunnel: [w2168] -> w2078
          tunnel: w2077 -> [w2168]
          tunnel: w2074 -> [w2167]
          tunnel: [w2167] -> w2073
          tunnel: [w2166] -> w2070
          tunnel: w2069 -> [w2166]
          tunnel: [w2165] -> w2066
          tunnel: w2065 -> [w2165]
          tunnel: [w2164] -> w2044
          tunnel: w2043 -> [w2164]
          tunnel: w2092 -> [w2184]
          tunnel: w2090 -> [w2183]
          tunnel: w2078 -> [w2182]
          tunnel: w2073 -> [w2180]
          tunnel: w2070 -> [w2181]
          tunnel: w2066 -> [w2179]
          tunnel: [w2180] -> w1980
          tunnel: [w2179] -> w1978
          tunnel: [w2177] -> w1976
          tunnel: [w2176] -> w1974
          tunnel: [w2175] -> w1972
          tunnel: w2044 -> [w2175]
          tunnel: [w2174] -> w1970
          tunnel: [w2173] -> w1968
          tunnel: w1980 -> [w2195]
          tunnel: [w2195] -> w1979
          tunnel: w1978 -> [w2194]
          tunnel: [w2194] -> w1977
          tunnel: w1976 -> [w2193]
          tunnel: [w2193] -> w1975
          tunnel: w1974 -> [w2192]
          tunnel: [w2192] -> w1973
          tunnel: w1972 -> [w2191]
          tunnel: [w2191] -> w1971
          tunnel: w1970 -> [w2190]
          tunnel: [w2189] -> w1969
          tunnel: w1968 -> [w2188]
          tunnel: [w2187] -> w1967
          tunnel: [w2199] -> w1994
          tunnel: [w2198] -> w1992
          tunnel: [w2197] -> w1990
          tunnel: [w2206] -> w1988
          tunnel: [w2203] -> w1986
          tunnel: [w2205] -> w1984
          tunnel: w1979 -> [w2208]
          tunnel: w1977 -> [w2207]
          tunnel: w1975 -> [w2197]
          tunnel: w1973 -> [w2203]
          tunnel: w1971 -> [w2202]
          tunnel: [w2201] -> w1982
          tunnel: w1969 -> [w2199]
          tunnel: w1967 -> [w2198]
          tunnel: w1994 -> [w2217]
          tunnel: [w2217] -> w1993
          tunnel: w1992 -> [w2216]
          tunnel: [w2216] -> w1991
          tunnel: w1990 -> [w2211]
          tunnel: [w2210] -> w1989
          tunnel: w1988 -> [w2215]
          tunnel: [w2215] -> w1987
          tunnel: w1986 -> [w2214]
          tunnel: [w2214] -> w1985
          tunnel: w1984 -> [w2213]
          tunnel: [w2213] -> w1983
          tunnel: w1982 -> [w2212]
          tunnel: [w2212] -> w1981
          tunnel: w1993 -> [w2223]
          tunnel: w1991 -> [w2222]
          tunnel: w1989 -> [w2227]
          tunnel: [w2227] -> w2001
          tunnel: w1987 -> [w2226]
          tunnel: [w2226] -> w2000
          tunnel: w1985 -> [w2225]
          tunnel: [w2225] -> w1999
          tunnel: w1983 -> [w2224]
          tunnel: [w2224] -> w1998
          tunnel: [w2221] -> w1997
          tunnel: [w2220] -> w1996
          tunnel: [w2218] -> w1995
          tunnel: w1981 -> [w2218]
          tunnel: w1997 -> [w2240]
          tunnel: w1996 -> [w2239]
          tunnel: w2001 -> [w2238]
          tunnel: w1999 -> [w2237]
          tunnel: w2000 -> [w2236]
          tunnel: w1998 -> [w2235]
          tunnel: w1995 -> [w2231]
          tunnel: [w2240] -> w2040
          tunnel: [w2239] -> w2039
          tunnel: [w2238] -> w2038
          tunnel: [w2237] -> w2037
          tunnel: [w2234] -> w2036
          tunnel: [w2233] -> w2035
          tunnel: [w2229] -> w2034
          tunnel: w2040 -> [w2250]
          tunnel: w2039 -> [w2249]
          tunnel: w2038 -> [w2248]
          tunnel: w2037 -> [w2247]
          tunnel: w2036 -> [w2244]
          tunnel: w2035 -> [w2246]
          tunnel: w2034 -> [w2245]
          tunnel: [w2250] -> w2026
          tunnel: [w2249] -> w2025
          tunnel: [w2248] -> w2024
          tunnel: [w2247] -> w2023
          tunnel: [w2243] -> w2022
          tunnel: [w2246] -> w2021
          tunnel: [w2245] -> w2020
          tunnel: w2026 -> [w2260]
          tunnel: [w2260] -> w1966
          tunnel: w2025 -> [w2259]
          tunnel: [w2259] -> w1965
          tunnel: w2024 -> [w2258]
          tunnel: [w2258] -> w1964
          tunnel: w2023 -> [w2257]
          tunnel: [w2257] -> w1963
          tunnel: w2022 -> [w2253]
          tunnel: [w2252] -> w1962
          tunnel: w2021 -> [w2256]
          tunnel: [w2256] -> w1961
          tunnel: w2020 -> [w2255]
          tunnel: [w2255] -> w1960
          tunnel: w1966 -> [w2270]
          tunnel: [w2270] -> w1959
          tunnel: w1965 -> [w2269]
          tunnel: [w2269] -> w1958
          tunnel: w1964 -> [w2268]
          tunnel: [w2268] -> w1957
          tunnel: w1963 -> [w2267]
          tunnel: [w2267] -> w1956
          tunnel: w1962 -> [w2264]
          tunnel: [w2263] -> w1955
          tunnel: w1961 -> [w2266]
          tunnel: [w2266] -> w1954
          tunnel: w1960 -> [w2265]
          tunnel: [w2265] -> w1953
          tunnel: w1959 -> [w2280]
          tunnel: [w2280] -> w1952
          tunnel: w1958 -> [w2279]
          tunnel: [w2279] -> w1951
          tunnel: w1957 -> [w2278]
          tunnel: [w2278] -> w1950
          tunnel: w1956 -> [w2277]
          tunnel: [w2277] -> w1949
          tunnel: w1955 -> [w2274]
          tunnel: w1954 -> [w2276]
          tunnel: [w2276] -> w1948
          tunnel: w1953 -> [w2275]
          tunnel: [w2275] -> w1947
          tunnel: [w2273] -> w1934
          tunnel: w1952 -> [w2290]
          tunnel: [w2290] -> w1946
          tunnel: w1951 -> [w2289]
          tunnel: [w2289] -> w1944
          tunnel: w1950 -> [w2288]
          tunnel: [w2288] -> w1942
          tunnel: w1949 -> [w2287]
          tunnel: [w2287] -> w1940
          tunnel: w1948 -> [w2286]
          tunnel: [w2286] -> w1938
          tunnel: w1947 -> [w2285]
          tunnel: [w2285] -> w1936
          tunnel: w1934 -> [w2284]
          tunnel: [w2283] -> w1933
          tunnel: w1946 -> [w2300]
          tunnel: [w2300] -> w1945
          tunnel: w1944 -> [w2299]
          tunnel: [w2299] -> w1943
          tunnel: w1942 -> [w2298]
          tunnel: [w2298] -> w1941
          tunnel: w1940 -> [w2297]
          tunnel: [w2297] -> w1939
          tunnel: w1938 -> [w2296]
          tunnel: [w2296] -> w1937
          tunnel: w1936 -> [w2295]
          tunnel: [w2295] -> w1935
          tunnel: w1933 -> [w2294]
          tunnel: [w2293] -> w1932
          tunnel: w1945 -> [w2310]
          tunnel: w1943 -> [w2309]
          tunnel: w1941 -> [w2308]
          tunnel: w1939 -> [w2307]
          tunnel: w1937 -> [w2306]
          tunnel: w1935 -> [w2305]
          tunnel: [w2310] -> w2033
          tunnel: [w2309] -> w2032
          tunnel: [w2308] -> w2031
          tunnel: [w2307] -> w2030
          tunnel: [w2304] -> w2029
          tunnel: [w2306] -> w2028
          tunnel: [w2305] -> w2027
          tunnel: w1932 -> [w2301]
          tunnel: w2033 -> [w2321]
          tunnel: w2032 -> [w2320]
          tunnel: w2031 -> [w2319]
          tunnel: w2030 -> [w2318]
          tunnel: w2029 -> [w2316]
          tunnel: w2028 -> [w2317]
          tunnel: w2027 -> [w2312]
          tunnel: [w2321] -> w2007
          tunnel: [w2320] -> w2006
          tunnel: [w2319] -> w2005
          tunnel: [w2318] -> w2004
          tunnel: [w2315] -> w2003
          tunnel: [w2317] -> w2002
          tunnel: [w2312] -> w1931
          tunnel: [w2323] -> w2041
          tunnel: [w2326] -> w2057
          tunnel: [w2327] -> w2058
          tunnel: [w2330] -> w2061
          tunnel: [w2331] -> w2062
          tunnel: [w2332] -> w2085
          tunnel: [w2333] -> w2086
          tunnel: w2007 -> [w2333]
          tunnel: w2006 -> [w2332]
          tunnel: w2005 -> [w2331]
          tunnel: w2004 -> [w2330]
          tunnel: w2003 -> [w2329]
          tunnel: w2002 -> [w2328]
          tunnel: w1931 -> [w2324]
          frame #0 {
            n469 = call-poly <vilib>:"DAQmx Write.vi"("task/channels in"=w2152, "data"=TRUE, "error in"=w2151) -> ("task out"=w2149:refnum<k21>, "error out"=w2148:errorcluster)  [unwired: 10 in, 1 out]
            n470 = Wait (ms)(milliseconds to wait=u32 1000) -> ()  [unwired: 1 out]
          }
          frame #1 {
            n471 = call-poly <vilib>:"DAQmx Write.vi"("task/channels in"=w2162, "data"=FALSE, "error in"=w2161) -> ("task out"=w2159:refnum<k21>, "error out"=w2158:errorcluster)  [unwired: 10 in, 1 out]
          }
          frame #2 {
            n472 = Wait (ms)(milliseconds to wait="waiting time for\n robotic arm") -> ()  [unwired: 1 out]
          }
          frame #3 {
            n473 = call-poly <vilib>:"DAQmx Write.vi"("task/channels in"=w2184, "data"=TRUE, "error in"=w2183) -> ("task out"=w2174:refnum<k21>, "error out"=w2173:errorcluster)  [unwired: 10 in, 1 out]
            n474 = call-poly <vilib>:"DAQmx Write.vi"("task/channels in"=w2182, "data"=TRUE, "error in"=w2181) -> ("task out"=w2177:refnum<k21>, "error out"=w2176:errorcluster)  [unwired: 10 in, 1 out]
            n475 = Wait (ms)(milliseconds to wait=u32 2000 ("milliseconds to wait 4")) -> ()  [unwired: 1 out]
          }
          frame #4 {
            n476 = call-poly <vilib>:"DAQmx Write.vi"("task/channels in"=w2190, "data"=FALSE, "error in"=w2188) -> ("task out"=w2189:refnum<k21>, "error out"=w2187:errorcluster)  [unwired: 10 in, 1 out]
            n477 = Wait (ms)(milliseconds to wait=u32 500) -> ()  [unwired: 1 out]
          }
          frame #5 {
            n478 = call-poly <vilib>:"DAQmx Write.vi"("task/channels in"=w2202, "data"=TRUE) -> ("task out"=w2201:refnum<k21>)  [unwired: 11 in, 2 out]
            n479 = call-poly <vilib>:"DAQmx Write.vi"("task/channels in"=w2208, "data"=TRUE, "error in"=w2207) -> ("task out"=w2206:refnum<k21>, "error out"=w2205:errorcluster)  [unwired: 10 in, 1 out]
            n480 = Wait (ms)(milliseconds to wait="shower time") -> ()  [unwired: 1 out]
          }
          frame #6 {
            n481 = call-poly <vilib>:"DAQmx Write.vi"("task/channels in"=w2211, "data"=FALSE) -> ("task out"=w2210:refnum<k21>)  [unwired: 11 in, 2 out]
          }
          frame #7 {
            n482 = call-poly <vilib>:"DAQmx Write.vi"("task/channels in"=w2223, "data"=FALSE, "error in"=w2222) -> ("task out"=w2221:refnum<k21>, "error out"=w2220:errorcluster)  [unwired: 10 in, 1 out]
          }
          frame #8 {
            n483 = call-poly <vilib>:"DAQmx Write.vi"("task/channels in"=w2236, "data"=TRUE, "error in"=w2235) -> ("task out"=w2234:refnum<k21>, "error out"=w2233:errorcluster)  [unwired: 10 in, 1 out]
            n484 = call-poly <vilib>:"DAQmx Write.vi"("task/channels in"=w2231, "data"=TRUE) -> ("task out"=w2229:refnum<k21>)  [unwired: 11 in, 2 out]
            n485 = Wait (ms)(milliseconds to wait=u32 2000) -> ()  [unwired: 1 out]
          }
          frame #9 {
            n486 = call-poly <vilib>:"DAQmx Write.vi"("task/channels in"=w2244, "data"=FALSE) -> ("task out"=w2243:refnum<k21>)  [unwired: 11 in, 2 out]
            n487 = Wait (ms)(milliseconds to wait=u32 500) -> ()  [unwired: 1 out]
          }
          frame #10 {
            n488 = call-poly <vilib>:"DAQmx Write.vi"("task/channels in"=w2253, "data"=TRUE) -> ("task out"=w2252:refnum<k21>)  [unwired: 11 in, 2 out]
            n489 = Wait (ms)(milliseconds to wait=u32 500) -> ()  [unwired: 1 out]
          }
          frame #11 {
            n490 = call-poly <vilib>:"DAQmx Write.vi"("task/channels in"=w2264, "data"=FALSE) -> ("task out"=w2263:refnum<k21>)  [unwired: 11 in, 2 out]
            n491 = Wait (ms)(milliseconds to wait=u32 500) -> ()  [unwired: 1 out]
          }
          frame #12 {
            n492 = call-poly <vilib>:"DAQmx Write.vi"("task/channels in"=w2274, "data"=TRUE) -> ("task out"=w2273:refnum<k21>)  [unwired: 11 in, 2 out]
            n493 = Wait (ms)(milliseconds to wait=u32 500) -> ()  [unwired: 1 out]
          }
          frame #13 {
            n494 = call-poly <vilib>:"DAQmx Write.vi"("task/channels in"=w2284, "data"=FALSE) -> ("task out"=w2283:refnum<k21>)  [unwired: 11 in, 2 out]
            n495 = Wait (ms)(milliseconds to wait=u32 500) -> ()  [unwired: 1 out]
          }
          frame #14 {
            n496 = call-poly <vilib>:"DAQmx Write.vi"("task/channels in"=w2294, "data"=TRUE) -> ("task out"=w2293:refnum<k21>)  [unwired: 11 in, 2 out]
            n497 = Wait (ms)(milliseconds to wait=u32 3000) -> ()  [unwired: 1 out]
          }
          frame #15 {
            n498 = call-poly <vilib>:"DAQmx Write.vi"("task/channels in"=w2301, "data"=FALSE) -> ("task out"=w2304:refnum<k21>)  [unwired: 11 in, 2 out]
            n499 = Wait (ms)(milliseconds to wait=u32 500) -> ()  [unwired: 1 out]
          }
          frame #16 {
            n500 = call-poly <vilib>:"DAQmx Write.vi"("task/channels in"=w2316, "data"=TRUE) -> ("task out"=w2315:refnum<k21>)  [unwired: 11 in, 2 out]
            n501 = local write "tube changing #"(0 ("tube changing #")) -> ()
            n502 = Wait (ms)(milliseconds to wait="washing time") -> ()  [unwired: 1 out]
          }
          frame #17 {
            n503 = call-poly <vilib>:"DAQmx Write.vi"("task/channels in"=w2329, "data"=FALSE, "error in"=w2328) -> ("task out"=w2327:refnum<k21>, "error out"=w2326:errorcluster)  [unwired: 10 in, 1 out]
            n504 = call-poly <vilib>:"DAQmx Write.vi"("task/channels in"=w2324, "data"=FALSE) -> ("task out"=w2323:refnum<k21>)  [unwired: 11 in, 2 out]
          }
        }
        n505 = Greater?(x=w1927, y="tube to stop") -> (0:w1925:bool)
        n506 = case shown="False" w1925 {
          tunnel: [w2121 states."Close"] -> w2054
          frame False {
            n507 = local read "Continuous\nacquisition"() -> (w2120:bool)
            n508 = case shown="False" w2120 {
              tunnel: [states."Chilling" states."auto imaging"] -> w2121
              frame False {
              }
              frame True {
              }
            }
          }
          frame True {
          }
        }
        n509 = call <vilib>:"DAQmx Stop Task.vi"("task/channels in"=w2058, "error in"=w2057) -> ("task out"=w2060:refnum<k21>, "error out"=w2059:errorcluster)  [unwired: 12 in]
        n510 = call <vilib>:"DAQmx Clear Task.vi"("task in"=w2060, "error in"=w2059) -> ()  [unwired: 13 in, 1 out]
        n511 = call <vilib>:"DAQmx Stop Task.vi"("task/channels in"=w2062, "error in"=w2061) -> ("task out"=w2064:refnum<k21>, "error out"=w2063:errorcluster)  [unwired: 12 in]
        n512 = call <vilib>:"DAQmx Clear Task.vi"("task in"=w2064, "error in"=w2063) -> ()  [unwired: 13 in, 1 out]
        n513 = call <vilib>:"DAQmx Stop Task.vi"("task/channels in"=w2086, "error in"=w2085) -> ("task out"=w2088:refnum<k21>, "error out"=w2087:errorcluster)  [unwired: 12 in]
        n514 = call <vilib>:"DAQmx Clear Task.vi"("task in"=w2088, "error in"=w2087) -> ()  [unwired: 13 in, 1 out]
      }
      frame "manual loading" {
        # "shower valves"
        n515 = call-poly <vilib>:"DAQmx Create Virtual Channel.vi"("lines"=tag "Dev1/port1/line2") -> ("task out"=w2375:refnum<k21>, "error out"=w2374:errorcluster)  [unwired: 13 in]
        n516 = call-poly <vilib>:"DAQmx Create Virtual Channel.vi"("lines"=tag "Dev1/port1/line3") -> ("task out"=w2373:refnum<k21>, "error out"=w2372:errorcluster)  [unwired: 13 in]
        n517 = call-poly <vilib>:"DAQmx Create Virtual Channel.vi"("lines"=tag "Dev1/port1/line4") -> ("task out"=w2371:refnum<k21>, "error out"=w2370:errorcluster)  [unwired: 13 in]
        n518 = call <vilib>:"DAQmx Start Task.vi"("task/channels in"=w2375, "error in"=w2374) -> ("task out"=w2368:refnum<k21>)  [unwired: 12 in, 1 out]
        n519 = call <vilib>:"DAQmx Start Task.vi"("task/channels in"=w2373, "error in"=w2372) -> ("task out"=w2367:refnum<k21>)  [unwired: 12 in, 1 out]
        n520 = call <vilib>:"DAQmx Start Task.vi"("task/channels in"=w2371, "error in"=w2370) -> ("task out"=w2369:refnum<k21>)  [unwired: 12 in, 1 out]
        n521 = flat-sequence {
          tunnel: w2369 -> [w2416]
          tunnel: w2368 -> [w2418]
          tunnel: w2367 -> [w2417]
          tunnel: [w2418] -> w2366
          tunnel: [w2417] -> w2365
          tunnel: [w2413] -> w2364
          tunnel: w2366 -> [w2426]
          tunnel: w2365 -> [w2425]
          tunnel: w2364 -> [w2421]
          tunnel: [w2421] -> w2363
          tunnel: [w2420] -> w2362
          tunnel: [w2419] -> w2357
          tunnel: w2363 -> [w2428]
          tunnel: w2362 -> [w2432]
          tunnel: [w2430] -> w2361
          tunnel: w2357 -> [w2429]
          tunnel: [w2429] -> w2353
          tunnel: [w2428] -> w2352
          tunnel: w2361 -> [w2440]
          tunnel: [w2439] -> w2360
          tunnel: [w2438] -> w2354
          tunnel: w2353 -> [w2438]
          tunnel: w2352 -> [w2437]
          tunnel: [w2434] -> w2343
          tunnel: w2360 -> [w2446]
          tunnel: [w2445] -> w2359
          tunnel: [w2444] -> w2355
          tunnel: w2354 -> [w2444]
          tunnel: w2343 -> [w2442]
          tunnel: [w2442] -> w2341
          tunnel: w2359 -> [w2452]
          tunnel: [w2451] -> w2358
          tunnel: [w2450] -> w2356
          tunnel: w2355 -> [w2450]
          tunnel: [w2448] -> w2342
          tunnel: w2341 -> [w2448]
          tunnel: w2358 -> [w2459]
          tunnel: w2356 -> [w2458]
          tunnel: [w2456] -> w2345
          tunnel: [w2455] -> w2344
          tunnel: [w2454] -> w2340
          tunnel: w2342 -> [w2454]
          frame #0 {
            n522 = call-poly <vilib>:"DAQmx Write.vi"("task/channels in"=w2416, "data"=TRUE) -> ("task out"=w2413:refnum<k21>)  [unwired: 11 in, 2 out]
            n523 = Wait (ms)(milliseconds to wait=u32 1000) -> ()  [unwired: 1 out]
          }
          frame #1 {
            n524 = call-poly <vilib>:"DAQmx Write.vi"("task/channels in"=w2426, "data"=TRUE) -> ("task out"=w2419:refnum<k21>)  [unwired: 11 in, 2 out]
            n525 = call-poly <vilib>:"DAQmx Write.vi"("task/channels in"=w2425, "data"=TRUE) -> ("task out"=w2420:refnum<k21>)  [unwired: 11 in, 2 out]
            n526 = Wait (ms)(milliseconds to wait="shower time(ms)") -> ()  [unwired: 1 out]
          }
          frame #2 {
            n527 = call-poly <vilib>:"DAQmx Write.vi"("task/channels in"=w2432, "data"=FALSE) -> ("task out"=w2430:refnum<k21>)  [unwired: 11 in, 2 out]
            n528 = Wait (ms)(milliseconds to wait=u32 500) -> ()  [unwired: 1 out]
          }
          frame #3 {
            n529 = call-poly <vilib>:"DAQmx Write.vi"("task/channels in"=w2440, "data"=TRUE ("auto start")) -> ("task out"=w2439:refnum<k21>)  [unwired: 11 in, 2 out]
            n530 = call-poly <vilib>:"DAQmx Write.vi"("task/channels in"=w2437, "data"=FALSE) -> ("task out"=w2434:refnum<k21>)  [unwired: 11 in, 2 out]
            n531 = Wait (ms)(milliseconds to wait=u32 500) -> ()  [unwired: 1 out]
          }
          frame #4 {
            n532 = call-poly <vilib>:"DAQmx Write.vi"("task/channels in"=w2446, "data"=FALSE ("auto start")) -> ("task out"=w2445:refnum<k21>)  [unwired: 11 in, 2 out]
            n533 = Wait (ms)(milliseconds to wait=u32 500) -> ()  [unwired: 1 out]
          }
          frame #5 {
            n534 = call-poly <vilib>:"DAQmx Write.vi"("task/channels in"=w2452, "data"=TRUE ("auto start")) -> ("task out"=w2451:refnum<k21>)  [unwired: 11 in, 2 out]
            n535 = Wait (ms)(milliseconds to wait=u32 2000) -> ()  [unwired: 1 out]
          }
          frame #6 {
            n536 = call-poly <vilib>:"DAQmx Write.vi"("task/channels in"=w2459, "data"=FALSE ("auto start")) -> ("task out"=w2456:refnum<k21>)  [unwired: 11 in, 2 out]
            n537 = call-poly <vilib>:"DAQmx Write.vi"("task/channels in"=w2458, "data"=FALSE) -> ("task out"=w2455:refnum<k21>)  [unwired: 11 in, 2 out]
          }
        }
        n538 = call <vilib>:"DAQmx Stop Task.vi"("task/channels in"=w2345) -> ("task out"=w2351:refnum<k21>, "error out"=w2350:errorcluster)  [unwired: 13 in]
        n539 = call <vilib>:"DAQmx Stop Task.vi"("task/channels in"=w2344) -> ("task out"=w2349:refnum<k21>, "error out"=w2348:errorcluster)  [unwired: 13 in]
        n540 = call <vilib>:"DAQmx Stop Task.vi"("task/channels in"=w2340) -> ("task out"=w2347:refnum<k21>, "error out"=w2346:errorcluster)  [unwired: 13 in]
        n541 = call <vilib>:"DAQmx Clear Task.vi"("task in"=w2351, "error in"=w2350) -> ()  [unwired: 13 in, 1 out]
        n542 = call <vilib>:"DAQmx Clear Task.vi"("task in"=w2349, "error in"=w2348) -> ()  [unwired: 13 in, 1 out]
        n543 = call <vilib>:"DAQmx Clear Task.vi"("task in"=w2347, "error in"=w2346) -> ()  [unwired: 13 in, 1 out]
        n544 = local read "Continuous\nacquisition"() -> (w2339:bool)
        n545 = case shown="False" w2339 {
          tunnel: [states."Chilling" states."auto imaging"] -> w2338
          frame False {
          }
          frame True {
          }
        }
      }
      frame "Find boundaries" {
        n546 = local read "Last saved #"() -> (w2481:i32)
        n547 = call <userlib>:"tm_startcapture_40.vi"("error in (no error)"=w2526, "Handle in"=w2528) -> ("error out"=w2525:errorcluster, "Handle out"=w2527:u32)  [unwired: 8 in]
        n548 = stacked-sequence {
          tunnel: [w2568] -> w2535
          tunnel: w2507 -> [w2568]
          tunnel: [w2569] -> w2537
          frame #0 {
            w2569 = "\r\n"
            w2572 = u8 2 items=["0", "1", "2", "3", "4"] ("Axis Number")
            n549 = local write "Moving"(TRUE ("Moving")) -> ()
            n550 = Wait (ms)(milliseconds to wait=u32 100) -> ()  [unwired: 1 out]
            n551 = call "RS232C_SetSpeed.vi"("Low Speed"="Low Speed", "High Speed"="Go to edge speed", "Acceleration Time"="Acceleration Time", "Axis Number"=w2572, "Delimiter"=w2569, "VISAリソース名"=w2568, "Axis Count"=u8 2, "Range"=TRUE, "Main/Sub"=TRUE) -> ()  [unwired: 2 out]
          }
        }
        n552 = local read "Movement direction"() -> (w2538:bool)
        n553 = flat-sequence {
          tunnel: w2535 -> [w2584]
          tunnel: w2537 -> [w2583]
          tunnel: "Go to edge pulses" -> [w2585]
          tunnel: w2538 -> [w2579]
          tunnel: w2527 -> [w2586]
          tunnel: w2525 -> [w2587]
          tunnel: w2539 -> [w2588]
          tunnel: [w2588] -> w2504
          tunnel: [w2587] -> w2503
          tunnel: [w2586] -> w2502
          tunnel: [w2579] -> w2501
          tunnel: [w2585] -> w2500
          tunnel: [w2583] -> w2499
          tunnel: [w2584] -> w2498
          tunnel: ["First move"] -> w2496
          tunnel: [w2601] -> w2536
          tunnel: [w2599] -> w2534
          tunnel: [w2598] -> w2533
          tunnel: [w2597] -> w2532
          tunnel: [w2596] -> w2531
          tunnel: [w2595] -> w2530
          tunnel: [w2594] -> w2529
          tunnel: [w2591] -> w2509
          tunnel: w2504 -> [w2605]
          tunnel: w2503 -> [w2604]
          tunnel: w2502 -> [w2603]
          tunnel: w2501 -> [w2597]
          tunnel: w2500 -> [w2598]
          tunnel: w2499 -> [w2599]
          tunnel: w2498 -> [w2601]
          tunnel: [w2590] -> w2483
          tunnel: [w2589] -> w2482
          tunnel: w2536 -> [w2669]
          tunnel: w2534 -> [w2672]
          tunnel: w2533 -> [w2677]
          tunnel: w2532 -> [w2668]
          tunnel: w2531 -> [w2670]
          tunnel: w2530 -> [w2671]
          tunnel: w2529 -> [w2667]
          tunnel: [w2672] -> w2514
          tunnel: [w2671] -> w2513
          tunnel: [w2670] -> w2512
          tunnel: [w2669] -> w2511
          tunnel: [w2668] -> w2505
          tunnel: [w2667] -> w2510
          tunnel: w2509 -> [w2666]
          tunnel: [w2666] -> w2508
          frame #0 {
            w2581 = u8 2 items=["0", "1", "2", "3", "4"] ("Axis Number")
            n554 = Wait (ms)(milliseconds to wait=u32 100) -> ()  [unwired: 1 out]
            n555 = call "RS232C_Move.vi"("VISAリソース名"=w2584, "Axis Count"=u8 2, "Axis Number"=w2581, "Pulse Number"="First move", "Direction"=w2579, "Delimiter"=w2583, "Main/Sub"=FALSE) -> ()  [unwired: 2 out]
          }
          frame #1 {
            n556 = while {
              tunnel: w2601 -> [w2647]
              tunnel: w2599 -> [w2646]
              tunnel: [w2644] -> w2600
              shift-right: [w2640] -> _
              shift-left: 0 -> [w2641]
              tunnel: w2598 -> [w2638]
              shift-right: [w2632] -> w2591
              shift-left: 0 -> [w2639]
              tunnel: w2602 -> [w2636]
              tunnel: w2597 -> [w2635]
              tunnel: [w2628] -> w2590
              stop <- w2643 stop-if-true
              # "find boundary jogs"
              n557 = call <extravilib>:"Read.vi"("channel"=w2636) -> ("element"=w2633:dbl)  [unwired: 1 in, 1 out]
              n558 = Greater?(x=w2641, y=2) -> ()  [unwired: 1 out]
              n559 = local read "Mean trigger"() -> (w2634:i32)
              n560 = local write "Sub img mean"(w2633) -> ()
              n561 = Wait (ms)(milliseconds to wait=u32 50) -> ()  [unwired: 1 out]
              n562 = Greater?(x=w2634, y=w2633) -> (0:w2645:bool)
              n563 = case shown="True" w2645 {
                tunnel: w2647 -> [_ w2661]
                tunnel: w2646 -> [_ w2660]
                tunnel: w2638 -> [_ w2659]
                tunnel: w2635 -> [_ w2658]
                tunnel: w2635 -> [_ _]
                tunnel: w2641 -> [w2652 w2657]
                tunnel: [w2650 w2657] -> w2640
                tunnel: w2639 -> [w2649 w2656]
                tunnel: [w2649 w2654] -> w2632
                tunnel: [TRUE FALSE] -> w2627
                frame False {
                  n564 = Add(x=w2652, y=1) -> (x+y=w2650:i32)
                }
                frame True {
                  w2665 = u8 2 items=["0", "1", "2", "3", "4"] ("Axis Number")
                  # "Image is above threshold"
                  n565 = Add(x=w2656, y=1) -> (x+y=w2654:i32)
                  n566 = call "RS232C_Move.vi"("VISAリソース名"=w2661, "Axis Count"=u8 2, "Axis Number"=w2665, "Pulse Number"=w2659, "Direction"=w2658, "Delimiter"=w2660, "Main/Sub"=FALSE) -> ()  [unwired: 2 out]
                  n567 = Wait (ms)(milliseconds to wait="Wait v2") -> ()  [unwired: 1 out]
                }
              }
              n568 = Greater?(x=w2632, y=5) -> (0:w2628:bool)
              n569 = Or(x=w2628, y="Abort 2") -> (x .or. y?=w2629:bool)
              n570 = Or(x=w2627, y=w2629) -> (x .or. y?=w2643:bool)
              n571 = call <extravilib>:"Write.vi"("element"=w2643) -> ("channel"=w2644:T10)  [unwired: 1 out]
            }
            n572 = while {
              tunnel: w2603 -> [w2626]
              tunnel: w2604 -> [w2625]
              tunnel: [w2611] -> w2595
              tunnel: [w2612] -> w2596
              tunnel: w2600 -> [w2620]
              tunnel: [w2610] -> w2594
              tunnel: w2605 -> [w2610]
              tunnel: [w2608] -> w2602
              tunnel: [w2606] -> w2589
              stop <- w2619 stop-if-true
              n573 = call <extravilib>:"Read.vi"("channel"=w2620) -> ("element"=w2619:bool)  [unwired: 1 in, 1 out]
              n574 = call <userlib>:"tm_waitnextframe_40.vi"("error in (no error)"=w2625, "Handle in"=w2626) -> ("error out"=w2612:errorcluster, "Frame Count"=w2606:i32, "Frame Index"=w2613:i32, "Handle out"=w2611:u32)  [unwired: 6 in]
              n575 = local read "XS x px start"() -> (w2623:i32)
              n576 = local read "XS y length"() -> (w2617:i32)
              n577 = local read "XS y px start"() -> (w2624:i32)
              n578 = local read "XS x length"() -> (w2616:i32)
              n579 = Index Array(array=w2610, index=w2613) -> (element=w2614:T9)
              n580 = local write "Frame count"(w2606) -> ()
              n581 = Multiply(x=w2617, y=w2616) -> (x*y=w2615:i32)
              n582 = call "IMAQ ImageToArray"("Image"=w2614) -> ("Image Pixels (U16)"=w2609:u16[][])  [unwired: 3 in, 4 out]
              n583 = local write "Obtained image"(w2609) -> ()
              n584 = local read "Mean trigger"() -> (w2618:i32)
              n585 = Array Subset(array=w2609, index (row)=w2624, length (row)=w2617, index (col)=w2623, length (col)=w2616) -> (w2622:u16[][])
              n586 = Reshape Array(w2622, w2615) -> (w2621:u16[])
              n587 = local write "Sub image"(w2622) -> ()
              n588 = call-poly <vilib>:"Mean.vi"("X"=w2621) -> ("mean"=w2607:dbl)  [unwired: 1 out]
              n589 = local write "Sub img mean"(w2607) -> ()
              n590 = Greater Or Equal?(x=w2607, y=w2618) -> ()  [unwired: 1 out]
              n591 = call <extravilib>:"Write.vi"("element"=w2607) -> ("channel"=w2608:T11)  [unwired: 1 out]
            }
          }
          frame #2 {
            w2675 = u8 2 items=["0", "1", "2", "3", "4"] ("Axis Number")
            n592 = Wait (ms)(milliseconds to wait=u32 50) -> ()  [unwired: 1 out]
            n593 = call "RS232C_Move.vi"("VISAリソース名"=w2669, "Axis Count"=u8 2, "Axis Number"=w2675, "Pulse Number"=w2677, "Direction"=w2668, "Delimiter"=w2672, "Main/Sub"=FALSE) -> ()  [unwired: 2 out]
          }
        }
        n594 = local read "Continuous\nacquisition"() -> (w2476:bool)
        n595 = Insert Into Array(array=w2480, index=w2481, new element=w2482) -> (w2479:i32[])
        n596 = Add(x=w2508, y=1) -> (x+y=w2520:i32)
        n597 = Multiply(x="Go to edge pulses", y=w2520) -> (x*y=w2497:u32)
        n598 = Add(x=w2497, y=w2496) -> (x+y=w2495:u32)
        n599 = flat-sequence {
          tunnel: w2512 -> [w2558]
          tunnel: w2513 -> [w2559]
          tunnel: [w2559] -> w2522
          tunnel: [w2558] -> w2523
          tunnel: w2511 -> [w2554]
          tunnel: w2514 -> [w2553]
          tunnel: w2505 -> [w2551]
          tunnel: ["Return move"] -> w2506
          tunnel: [w2563] -> w2516
          tunnel: [w2562] -> w2517
          tunnel: w2523 -> [w2564]
          tunnel: w2522 -> [w2565]
          frame #0 {
            w2557 = u8 2 items=["0", "1", "2", "3", "4"] ("Axis Number")
            n600 = Not(x=w2551) -> (.not. x?=w2552:bool)
            n601 = Wait (ms)(milliseconds to wait=u32 100) -> ()  [unwired: 1 out]
            n602 = call "RS232C_Move.vi"("VISAリソース名"=w2554, "Axis Count"=u8 2, "Axis Number"=w2557, "Pulse Number"="Return move", "Direction"=w2552, "Delimiter"=w2553, "Main/Sub"=FALSE) -> ()  [unwired: 2 out]
          }
          frame #1 {
            w2561 = FALSE ("Stop producer")
            n603 = local write "Streaming"(w2561) -> ()
            n604 = local write "Moving"(w2561) -> ()
            n605 = Wait (ms)(milliseconds to wait=u32 100) -> ()  [unwired: 1 out]
            n606 = call <userlib>:"tm_stopcapture_40.vi"("error in (no error)"=w2564, "Handle in"=w2565) -> ("error out"=w2562:errorcluster, "Handle out"=w2563:u32)  [unwired: 8 in]
          }
        }
        n607 = case shown="False" w2483 {
          tunnel: [w2542 states."homing"] -> w2524
          tunnel: w2476 -> [w2540 _]
          frame False {
            n608 = case shown="False" "Enable screening\n(during flow zoometry)" {
              tunnel: [w2544 states."2000"] -> w2542
              tunnel: w2540 -> [w2543 _]
              frame False {
                n609 = case shown="False" w2543 {
                  tunnel: [states."Chilling" states."Acquire"] -> w2544
                  frame False {
                  }
                  frame True {
                  }
                }
              }
              frame True {
              }
            }
          }
          frame True {
          }
        }
        n610 = Subtract(x=w2495, y=w2506) -> (x-y=w2518:u32)
      }
      frame "Edgehunting" {
        w2732 = 120 ("dimension size")
        # "t"
        # "give up L size"
        n611 = while {
          tunnel: w2759 -> [w2825]
          tunnel: [w2822] -> w2694
          tunnel: ["scanning distance (um)"] -> _
          tunnel: ["Direction 2"] -> _
          tunnel: [w2818] -> w2741
          tunnel: [w2817] -> w2744
          stop <- w2820 stop-if-true
          n612 = stacked-sequence {
            tunnel: w2825 -> [w2827 w2836 _]
            tunnel: "Main/Sub" -> [w2828 w2842 _]
            tunnel: "scanning distance (um)" -> [_ w2839 _]
            tunnel: "Direction 2" -> [_ w2838 _]
            tunnel: "\r\n" -> [w2826 w2837 _]
            tunnel: [_ _ TRUE] -> w2820
            tunnel: [_ w2836 _] -> w2818
            tunnel: [_ w2837 _] -> w2817
            frame #0 {
              w2831 = u8 2 items=["0", "1", "2", "3", "4"] ("Axis Number")
              n613 = call "RS232C_SetSpeed.vi"("Low Speed"=u32 100, "High Speed"="High Speed 2", "Acceleration Time"=u16 100, "Axis Number"=w2831, "Delimiter"=w2826, "VISAリソース名"=w2827, "Axis Count"=u8 2, "Range"=TRUE, "Main/Sub"=w2828) -> ()  [unwired: 2 out]
              n614 = local write "OK Done"(FALSE ("OK Done")) -> ()
            }
            frame #1 {
              w2840 = u8 2 items=["0", "1", "2", "3", "4"] ("Axis Number")
              n615 = call "RS232C_Move.vi"("VISAリソース名"=w2836, "Axis Count"=u8 2, "Axis Number"=w2840, "Pulse Number"=w2839, "Direction"=w2838, "Delimiter"=w2837, "Main/Sub"=w2842) -> ()  [unwired: 2 out]
            }
            frame #2 {
            }
          }
          n616 = call <extravilib>:"Write.vi"("element"=w2820) -> ("channel"=w2822:T10)  [unwired: 1 out]
        }
        n617 = Increment(x=w2722) -> (x+1=w2721:u32)
        n618 = call <userlib>:"tm_startcapture_40.vi"("error in (no error)"=w2751, "Handle in"=w2753) -> ("error out"=w2757:errorcluster, "Handle out"=w2758:u32)  [unwired: 8 in]
        n619 = Initialize Array(0.0 ("element"), w2732) -> (w2748:dbl[])
        n620 = call <vilib>:"High Resolution Relative Seconds.vi"() -> ("relative seconds"=w2726:dbl)
        n621 = Initialize Array(0, 0 ("dimension size"), 0 ("dimension size")) -> (w2693:i32[][])
        n622 = Initialize Array(0 ("element"), 0 ("dimension size")) -> (w2688:i32[])
        n623 = Bundle(w2693, 0) -> (w2691:cluster{i32[][], i32})  [unwired: 1 in]
        n624 = Obtain Queue(name (unnamed)="stream", element data type=w2691) -> (queue out=w2696:refnum<queue>)  [unwired: 3 in, 2 out]
        n625 = while {
          tunnel: w2758 -> [w2870]
          tunnel: w2757 -> [w2869]
          tunnel: [w2860] -> w2756
          tunnel: [w2861] -> w2755
          tunnel: [w2859] -> w2746
          tunnel: w2750 -> [w2859]
          tunnel: [w2850] -> _
          tunnel: w2694 -> [w2856]
          shift-right: [w2853] -> w2747
          shift-left: w2748 -> [w2854]
          tunnel: [w2850] -> w2733
          shift-right: [w2849] -> w2695
          shift-left: w2696 -> [w2848]
          stop <- w2857 stop-if-true
          n626 = call <extravilib>:"Read.vi"("channel"=w2856) -> ("element"=w2857:bool)  [unwired: 1 in, 1 out]
          n627 = call <userlib>:"tm_waitnextframe_40.vi"("error in (no error)"=w2869, "Handle in"=w2870) -> ("error out"=w2861:errorcluster, "Frame Count"=w2850:i32, "Frame Index"=w2845:i32, "Handle out"=w2860:u32)  [unwired: 6 in]
          n628 = local read "XS x px start"() -> (w2867:i32)
          n629 = local read "XS y length"() -> (w2864:i32)
          n630 = local read "XS y px start"() -> (w2868:i32)
          n631 = local read "XS x length"() -> (w2863:i32)
          n632 = Index Array(array=w2859, index=w2845) -> (element=w2862:T9)
          n633 = local write "Frame count"(w2850) -> ()
          n634 = Multiply(x=w2864, y=w2863) -> (x*y=w2847:i32)
          n635 = call "IMAQ ImageToArray"("Image"=w2862) -> ("Image Pixels (U16)"=w2858:u16[][])  [unwired: 3 in, 4 out]
          n636 = local write "Obtained image"(w2858) -> ()
          n637 = local read "Mean trigger"() -> (w2865:i32)
          n638 = Array Subset(array=w2858, index (row)=w2868, length (row)=w2864, index (col)=w2867, length (col)=w2863) -> (w2846:u16[][])
          n639 = Bundle(w2846, "Frame Index"=w2845) -> (w2844:cluster{u16[][], "Frame Index":i32})  [unwired: 1 in]
          n640 = Reshape Array(w2846, w2847) -> (w2866:u16[])
          n641 = local write "Sub image"(w2846) -> ()
          n642 = Enqueue Element(queue=w2848, element=w2844) -> (queue out=w2849:refnum<queue>)  [unwired: 2 in, 2 out]
          n643 = call-poly <vilib>:"Mean.vi"("X"=w2866) -> ("mean"=w2855:dbl)  [unwired: 1 out]
          n644 = local write "Sub img mean"(w2855) -> ()
          n645 = Greater Or Equal?(x=w2855, y=w2865) -> (x >= y?=w2852:bool)
          n646 = Boolean To (0,1)(Boolean=w2852) -> (0, 1=w2851:i16)
          n647 = Replace Array Subset(array=w2854, new element=w2851, index=w2850) -> (w2853:dbl[])
        }
        "larvae size in scan" <- w2747
        n648 = while {
          shift-right: [w2785] -> _
          shift-left: w2696 -> [w2786]
          tunnel: w2694 -> [w2784]
          shift-right: [w2775] -> _
          shift-left: w2688 -> [w2776]
          stop <- w2783 stop-if-true
          n649 = call <extravilib>:"Read.vi"("channel"=w2784) -> ("element"=w2783:bool)  [unwired: 1 in, 1 out]
          n650 = Dequeue Element(queue=w2786) -> (queue out=w2785:refnum<queue>, element=w2782:cluster{i32[][], i32})  [unwired: 2 in, 2 out]
          n651 = Unbundle(w2782) -> (w2781:i32[][], w2777:i32)
          n652 = Array Max & Min(array=w2781) -> (max value=w2780:i32)  [unwired: 3 out]
          "max value" <- w2780
          n653 = Greater Or Equal?(x=w2780, y=300) -> (x >= y?=w2778:bool)
          n654 = case shown="True" w2778 {
            tunnel: w2777 -> [_ w2790]
            tunnel: w2776 -> [w2787 w2791]
            tunnel: [w2787 w2788] -> w2775
            frame False {
            }
            frame True {
              n655 = Insert Into Array(array=w2791, index=w2790, new element=1 ("new element/subarray")) -> (w2788:i32[])
            }
          }
        }
        n656 = Release Queue(queue=w2695) -> ()  [unwired: 2 in, 3 out]
        n657 = call <userlib>:"tm_stopcapture_40.vi"("error in (no error)"=w2755, "Handle in"=w2756) -> ("error out"=w2752:errorcluster, "Handle out"=w2754:u32)  [unwired: 8 in]
        n658 = flat-sequence {
          tunnel: w2747 -> [w2797]
          tunnel: w2746 -> [w2794]
          tunnel: w2744 -> [_]
          tunnel: [w2792] -> w2740
          tunnel: [w2794] -> w2737
          tunnel: [w2792] -> w2736
          tunnel: [w2793] -> w2735
          tunnel: [w2793] -> w2734
          tunnel: [w2792] -> w2731
          tunnel: w2737 -> [w2810]
          tunnel: w2736 -> [w2809]
          tunnel: w2735 -> [w2808]
          tunnel: w2734 -> [w2806]
          tunnel: w2733 -> [w2807]
          tunnel: w2732 -> [w2805]
          tunnel: w2731 -> [w2804]
          tunnel: [w2803] -> w2716
          tunnel: [w2803] -> w2682
          tunnel: [w2801] -> w2683
          tunnel: [w2810] -> w2705
          tunnel: [w2809] -> w2704
          tunnel: [w2808] -> w2703
          tunnel: [w2800] -> w2702
          tunnel: [w2812] -> w2742
          tunnel: [w2813] -> w2743
          tunnel: [w2814] -> w2745
          tunnel: w2705 -> [w2814]
          tunnel: w2704 -> [w2813]
          tunnel: w2703 -> [w2812]
          tunnel: w2702 -> [w2811]
          frame #0 {
            (unwired) 0.0 ("element")
            n659 = Search 1D Array(1D array=w2797, element=1.0, start index (0)=0) -> (index of element=w2792:i32)
            "R1" <- w2792
            n660 = Reverse 1D Array(array=w2797) -> (reversed array=w2796:dbl[])
            n661 = Search 1D Array(1D array=w2796, element=1.0) -> (index of element=w2793:i32)  [unwired: 1 in]
            "R2" <- w2793
          }
          frame #1 {
            n662 = Subtract(x=w2805, y=w2806) -> (x-y=w2803:i32)
            "real R2" <- w2803
            n663 = Subtract(x=w2807, y=w2803) -> ()  [unwired: 1 out]
            n664 = Subtract(x=w2803, y=w2804) -> (x-y=w2801:i32)
            "larva size in frame" <- w2801
            n665 = Greater?(x=10.0, y=w2801) -> (0:w2800:bool)
          }
          frame #2 {
            n666 = case shown="True" w2811 {
              frame False {
                n667 = local write "um to move"("um to move long") -> ()
              }
              frame True {
                n668 = local write "um to move"("um to move short") -> ()
              }
            }
          }
        }
        n669 = Greater?(x=w2740, y=0) -> (0:w2715:bool)
        n670 = local read "Continuous\nacquisition"() -> (w2739:bool)
        n671 = Less?(x=16 ("y"), y=w2716) -> (x < y?=w2714:bool)
        n672 = And(x=w2715, y=w2714) -> (x .and. y?=w2710:bool)
        n673 = Less?(x=w2683, y="maximum") -> (x < y?=w2684:bool)
        n674 = Less?(x="BUBBLE SIZE", y=w2683) -> (x < y?=w2685:bool)
        n675 = Less Or Equal?(x=w2682, y=85) -> (x <= y?=w2708:bool)
        n676 = And(x=w2710, y=w2708) -> (x .and. y?=w2706:bool)
        n677 = And(x=w2685, y=w2684) -> (x .and. y?=w2680:bool)
        n678 = And(x=w2680, y=w2706) -> (x .and. y?=w2707:bool)
        n679 = case shown="True" w2739 {
          tunnel: [states."gp" w2875] -> w2760
          tunnel: w2707 -> [_ w2874]
          tunnel: [w2871 w2873] -> w2723
          frame False {
            n680 = call <vilib>:"High Resolution Relative Seconds.vi"() -> ("relative seconds"=w2871:dbl)
          }
          frame True {
            n681 = case shown="False" w2874 {
              tunnel: [states."homing" states."gp"] -> w2875
              frame False {
              }
              frame True {
              }
            }
            n682 = call <vilib>:"High Resolution Relative Seconds.vi"() -> ("relative seconds"=w2873:dbl)
          }
        }
        n683 = Subtract(x=w2723, y=w2726) -> (x-y=w2725:dbl)
        n684 = Insert Into Array(array=w2728, index=w2722, new element=w2725) -> (w2727:dbl[])
        "#of edgehunting" <- w2722
      }
      frame "gp" {
        w2898 = 91 ("x")
        n685 = local read "Last saved #"() -> (w2885:i32)
        n686 = call <vilib>:"High Resolution Relative Seconds.vi"() -> ("relative seconds"=w2888:dbl)
        n687 = Subtract(x=120 ("y"), y=w2902) -> (x-y=w2901:i32)
        "RAL r2" <- w2901
        n688 = Subtract(x=w2898, y=w2901) -> (x-y=w2899:i32)
        "x-y 2" <- w2899
        n689 = while {
          tunnel: w2900 -> [_]
          tunnel: w2904 -> [_]
          tunnel: w2907 -> [w2951]
          tunnel: [w2952] -> w2905
          tunnel: w2898 -> [w2949]
          tunnel: w2899 -> [w2948]
          tunnel: [w2946] -> w2882
          stop <- w2947 stop-if-true
          n690 = case shown="True" TRUE {
            tunnel: [w2954 w2973] -> w2952
            tunnel: [TRUE ("OK Done") w2958] -> w2947
            tunnel: w2951 -> [w2954 w2970]
            tunnel: w2949 -> [_ w2964]
            tunnel: w2948 -> [_ w2963]
            tunnel: [-1 w2956] -> w2946
            frame False {
            }
            frame True {
              n691 = flat-sequence {
                tunnel: [w2975] -> w2972
                tunnel: [w2974] -> w2971
                tunnel: w2970 -> [w2975]
                tunnel: "\r\n" -> [w2974]
                tunnel: [w2985] -> w2968
                tunnel: [w2977] -> w2966
                tunnel: w2972 -> [w2985]
                tunnel: w2971 -> [w2977]
                tunnel: w2968 -> [w2995]
                tunnel: [w2995] -> w2967
                tunnel: w2966 -> [w2994]
                tunnel: [w2994] -> w2965
                tunnel: w2964 -> [w2993]
                tunnel: w2963 -> [w2989]
                tunnel: [w2986] -> w2962
                tunnel: [w2986] -> w2956
                tunnel: [w2997] -> w2973
                tunnel: w2967 -> [w2997]
                tunnel: w2965 -> [w2996]
                tunnel: w2962 -> [w2998]
                tunnel: [w3001] -> w2961
                tunnel: [w2997] -> w2960
                tunnel: [w2996] -> w2959
                tunnel: w2961 -> [w3007]
                tunnel: w2960 -> [w3010]
                tunnel: w2959 -> [w3009]
                tunnel: [w3008] -> w2958
                tunnel: w2957 -> [w3006]
                frame #0 {
                }
                frame #1 {
                  w2980 = u8 2 items=["0", "1", "2", "3", "4"] ("Axis Number")
                  n692 = call "RS232C_SetSpeed.vi"("Low Speed"=u32 100, "High Speed"=u32 20000, "Acceleration Time"=u16 100, "Axis Number"=w2980, "Delimiter"=w2977, "VISAリソース名"=w2985, "Axis Count"=u8 2, "Range"=TRUE, "Main/Sub"=FALSE) -> ()  [unwired: 2 out]
                  n693 = Wait (ms)(milliseconds to wait=u32 500) -> ()  [unwired: 1 out]
                }
                frame #2 {
                  n694 = local read "scanning distance (um)"() -> (w2991:u32)
                  n695 = Divide(x=w2989, y=w2993) -> (x/y=w2992:dbl)
                  n696 = Multiply(x=w2992, y=w2991) -> (x*y=w2988:dbl)
                  n697 = Add(x=w2988, y="correction") -> (x+y=w2987:dbl)
                  n698 = To Long Integer(number=w2987) -> (32bit integer=w2986:i32)
                  "backwards pulses" <- w2986
                }
                frame #3 {
                  w3004 = u8 2 items=["0", "1", "2", "3", "4"] ("Axis Number")
                  n699 = Wait (ms)(milliseconds to wait=u32 500) -> ()  [unwired: 1 out]
                  n700 = local read "Direction 2"() -> (w3000:bool)
                  n701 = Not(x=w3000) -> (.not. x?=w2999:bool)
                  n702 = call "RS232C_Move.vi"("VISAリソース名"=w2997, "Axis Count"=u8 2, "Axis Number"=w3004, "Pulse Number"=w2998, "Direction"=w2999, "Delimiter"=w2996, "Main/Sub"=FALSE) -> ("OK Done"=w3001:bool)  [unwired: 1 out]
                }
                frame #4 {
                  n703 = case shown="True" w3006 {
                    tunnel: w3010 -> [_ w3019]
                    tunnel: w3009 -> [_ w3018]
                    tunnel: [w3011 w3013] -> w3008
                    tunnel: w3007 -> [w3011 _]
                    frame False {
                    }
                    frame True {
                      w3014 = u8 2 items=["0", "1", "2", "3", "4"] ("Axis Number")
                      w3016 = u32 2000 ("Low Speed")
                      n704 = Wait (ms)(milliseconds to wait=u32 500) -> ()  [unwired: 1 out]
                      n705 = call "RS232C_SetSpeed.vi"("Low Speed"=w3016, "High Speed"=w3016, "Acceleration Time"=u16 0, "Axis Number"=w3014, "Delimiter"=w3018, "VISAリソース名"=w3019, "Axis Count"=u8 2, "Range"=TRUE, "Main/Sub"=FALSE) -> ("OK Done"=w3013:bool)  [unwired: 1 out]
                    }
                  }
                }
              }
              n706 = local read "Enable screening\n(during flow zoometry)"() -> (w2957:bool)
            }
          }
        }
        n707 = local read "Continuous\nacquisition"() -> (w2883:bool)
        n708 = case shown="True" w2883 {
          tunnel: [w2930 w2936] -> w2895
          tunnel: [w2931 w2935] -> w2887
          tunnel: w2882 -> [w2927 _]
          frame False {
            n709 = Less?(x=w2927, y=0) -> (x < y?=w2928:bool)
            n710 = call <vilib>:"High Resolution Relative Seconds.vi"() -> ("relative seconds"=w2931:dbl)
            n711 = case shown="True" w2928 {
              tunnel: [states."Stream w/o flow" states."homing"] -> w2930
              frame False {
              }
              frame True {
              }
            }
          }
          frame True {
            n712 = local read "Enable screening\n(during flow zoometry)"() -> (w2934:bool)
            n713 = case shown="True" w2934 {
              tunnel: [w2939 states."2000"] -> w2936
              tunnel: [w2937 w2944] -> w2935
              frame False {
                n714 = local read "4C"() -> (w2938:bool)
                n715 = case shown="False" w2938 {
                  tunnel: [states."Acquire" states."405"] -> w2939
                  tunnel: [w2940 w2942] -> w2937
                  frame False {
                    n716 = call <vilib>:"High Resolution Relative Seconds.vi"() -> ("relative seconds"=w2940:dbl)
                  }
                  frame True {
                    n717 = call <vilib>:"High Resolution Relative Seconds.vi"() -> ("relative seconds"=w2942:dbl)
                  }
                }
              }
              frame True {
                n718 = call <vilib>:"High Resolution Relative Seconds.vi"() -> ("relative seconds"=w2944:dbl)
              }
            }
          }
        }
        n719 = Subtract(x=w2887, y=w2888) -> (x-y=w2886:dbl)
        "gp" <- w2886
        n720 = Insert Into Array(array=w2889, index=w2885, new element=w2886) -> (w2884:dbl[])
      }
      frame "homing" {
        w3048 = u8 2 items=["0", "1", "2", "3", "4"] ("Axis Number")
        w3041 = "\r\n"
        w3042 = u8 2 items=["0", "1", "2", "3", "4"] ("Axis Number")
        n721 = Increment(x=w3073) -> (x+1=w3072:i32)
        "False triggers" <- w3072
        n722 = local write "Moving"(TRUE ("Moving")) -> ()
        n723 = flat-sequence {
          tunnel: u32 100 ("Low Speed") -> [w3091]
          tunnel: u32 20000 ("Go to edge speed 2") -> [w3090]
          tunnel: u16 100 ("Acceleration Time") -> [w3089]
          tunnel: w3042 -> [w3088]
          tunnel: w3041 -> [w3087]
          tunnel: w3040 -> [w3086]
          tunnel: u8 2 ("Axis Count") -> [w3085]
          tunnel: TRUE ("Range") -> [w3084]
          tunnel: TRUE ("Main/Sub") -> [w3083]
          tunnel: [w3110] -> w3050
          tunnel: w3027 -> [w3104]
          tunnel: w3025 -> [w3103]
          tunnel: w3050 -> [w3173]
          tunnel: w3040 -> [w3176]
          tunnel: u8 2 ("Axis Count") -> [w3175]
          tunnel: w3048 -> [w3174]
          tunnel: TRUE ("Direction") -> [w3172]
          tunnel: w3041 -> [w3171]
          tunnel: FALSE ("Main/Sub") -> [w3170]
          frame #0 {
            n724 = call "RS232C_SetSpeed.vi"("Low Speed"=w3091, "High Speed"=w3090, "Acceleration Time"=w3089, "Axis Number"=w3088, "Delimiter"=w3087, "VISAリソース名"=w3086, "Axis Count"=w3085, "Range"=w3084, "Main/Sub"=w3083) -> ("OK Done"=→"homing speed":bool)  [unwired: 1 out]
          }
          frame #1 {
            n725 = local read "maximum"() -> (w3093:i32)
            n726 = local read "BUBBLE SIZE"() -> (w3095:i32)
            n727 = local read "larva size in frame"() -> (w3092:i32)
            n728 = local read "real R2"() -> (w3098:i32)
            n729 = local read "real R2"() -> (w3101:i32)
            n730 = Greater?(x=w3093, y=w3092) -> (0:w3094:bool)
            n731 = local read "screening"() -> (w3107:bool)
            n732 = Greater?(x=w3104, y=0) -> (0:w3105:bool)
            n733 = local read "4C"() -> (w3109:bool)
            n734 = Less?(x=w3101, y=16) -> (x < y?=w3099:bool)
            n735 = Less Or Equal?(x=w3098, y=85) -> (x <= y?=w3096:bool)
            n736 = Greater?(x=w3092, y=w3095) -> (0:w3102:bool)
            "larva size" <- w3102
            n737 = Wait (ms)(milliseconds to wait=u32 500) -> ()  [unwired: 1 out]
            n738 = case shown="False" w3109 {
              tunnel: [w3112 w3123] -> w3110
              tunnel: w3107 -> [w3111 _]
              tunnel: w3105 -> [_ w3122]
              tunnel: w3103 -> [_ w3121]
              tunnel: w3102 -> [_ w3120]
              tunnel: w3099 -> [_ w3119]
              tunnel: w3096 -> [_ w3118]
              tunnel: w3094 -> [_ w3117]
              frame False {
                n739 = case shown="True" w3111 {
                  tunnel: [w3113 w3115] -> w3112
                  frame False {
                    n740 = local read "scanning distance (um)"() -> (w3113:u32)
                  }
                  frame True {
                    n741 = local read "backwards pulses"() -> (w3114:i32)
                    n742 = local read "scanning distance (um)"() -> (w3116:u32)
                    n743 = Subtract(x=w3116, y=w3114) -> (x-y=w3115:u32)
                  }
                }
              }
              frame True {
                n744 = case shown="True" w3122 {
                  tunnel: [w3124 w3133] -> w3123
                  tunnel: w3121 -> [_ w3129]
                  tunnel: w3120 -> [_ w3128]
                  tunnel: w3119 -> [_ w3127]
                  tunnel: w3118 -> [_ w3126]
                  tunnel: w3117 -> [_ w3125]
                  frame False {
                    n745 = local read "scanning distance (um)"() -> (w3124:u32)
                  }
                  frame True {
                    n746 = local read "backwards pulses"() -> (w3132:i32)
                    n747 = Greater?(x=w3132, y=0) -> (0:w3130:bool)
                    n748 = case shown="True" w3130 {
                      tunnel: [w3134 w3141] -> w3133
                      tunnel: w3132 -> [_ w3140]
                      tunnel: w3129 -> [_ w3139]
                      tunnel: w3128 -> [_ w3138]
                      tunnel: w3127 -> [_ w3137]
                      tunnel: w3126 -> [_ w3136]
                      tunnel: w3125 -> [_ w3135]
                      frame False {
                        n749 = local read "scanning distance (um)"() -> (w3134:u32)
                      }
                      frame True {
                        n750 = case shown="False" w3139 {
                          tunnel: [w3147 w3167] -> w3141
                          tunnel: w3140 -> [w3146 _]
                          tunnel: w3138 -> [w3145 _]
                          tunnel: w3137 -> [w3144 _]
                          tunnel: w3136 -> [w3143 _]
                          tunnel: w3135 -> [w3142 _]
                          frame False {
                            n751 = case shown="True" w3145 {
                              tunnel: [w3148 w3153] -> w3147
                              tunnel: w3146 -> [_ w3152]
                              tunnel: w3144 -> [_ w3151]
                              tunnel: w3143 -> [_ w3150]
                              tunnel: w3142 -> [_ w3149]
                              frame False {
                                n752 = local read "scanning distance (um)"() -> (w3148:u32)
                              }
                              frame True {
                                n753 = case shown="False" w3151 {
                                tunnel: [w3157 w3166] -> w3153
                                tunnel: w3152 -> [w3156 _]
                                tunnel: w3150 -> [w3155 _]
                                tunnel: w3149 -> [w3154 _]
                                frame False {
                                n754 = case shown="True" w3155 {
                                tunnel: [w3158 w3161] -> w3157
                                tunnel: w3156 -> [_ w3160]
                                tunnel: w3154 -> [_ w3159]
                                frame False {
                                n755 = local read "scanning distance (um)"() -> (w3158:u32)
                                }
                                frame True {
                                n756 = case shown="False" w3159 {
                                tunnel: [w3162 w3164] -> w3161
                                tunnel: w3160 -> [_ w3163]
                                frame False {
                                n757 = local read "scanning distance (um)"() -> (w3162:u32)
                                }
                                frame True {
                                n758 = local read "scanning distance (um)"() -> (w3165:u32)
                                n759 = Subtract(x=w3165, y=w3163) -> (x-y=w3164:u32)
                                }
                                }
                                }
                                }
                                }
                                frame True {
                                n760 = local read "scanning distance (um)"() -> (w3166:u32)
                                }
                                }
                              }
                            }
                          }
                          frame True {
                            n761 = local read "scanning distance (um)"() -> (w3167:u32)
                          }
                        }
                      }
                    }
                  }
                }
              }
            }
          }
          frame #2 {
            n762 = call "RS232C_Move.vi"("VISAリソース名"=w3176, "Axis Count"=w3175, "Axis Number"=w3174, "Pulse Number"=w3173, "Direction"=w3172, "Delimiter"=w3171, "Main/Sub"=w3170) -> ("OK Done"=→"homing":bool)  [unwired: 1 out]
            n763 = local write "screening"(FALSE ("screening 2")) -> ()
          }
        }
        n764 = local read "maximum"() -> (w3024:i32)
        n765 = local read "larva size in frame"() -> (w3033:i32)
        n766 = local read "Continuous\nacquisition"() -> (w3078:bool)
        n767 = Greater?(x=w3033, y=w3024) -> (0:w3030:bool)
        n768 = Less?(x=w3033, y=100) -> (x < y?=w3031:bool)
        n769 = And(x=w3031, y=w3030) -> (x .and. y?=w3025:bool)
        n770 = case shown="True" w3078 {
          tunnel: [states."Chilling" w3181] -> w3077
          tunnel: [FALSE ("homing speed") FALSE ("homing speed")] -> w3036
          tunnel: w3025 -> [_ w3179]
          frame False {
          }
          frame True {
            n771 = case shown="True" w3179 {
              tunnel: [states."auto imaging" states."light reverse"] -> w3181
              frame False {
              }
              frame True {
              }
            }
          }
        }
        n772 = local write "homing"(w3036) -> ()
        n773 = local write "homing speed"(w3036) -> ()
      }
      frame "Acquire" {
        (unwired) 0 ("x")
        (unwired) i16 3 ("width (-)")
        n774 = local read "Last saved file number 2000"() -> (w3189:i32)
        n775 = Add(x=1, y=w3217) -> (x+y=w3249:i32)
        n776 = local read "Frames in memory"() -> (w3260:i32)
        n777 = Insert Into Array(array=w3252, index=w3249, new element=w3251) -> (w3250:string[])
        n778 = Increment(x=w3226) -> (x+1=w3225:i32)
        n779 = flat-sequence {
          tunnel: [w3394] -> w3256
          tunnel: [w3395] -> w3266
          tunnel: [w3396] -> w3265
          tunnel: [w3388] -> w3269
          tunnel: w3286 -> [w3394]
          tunnel: w3289 -> [w3395]
          tunnel: w3288 -> [w3396]
          frame #0 {
            w3388 = "\r\n"
            w3390 = u8 2 items=["0", "1", "2", "3", "4"] ("Axis Number")
            n780 = Wait (ms)(milliseconds to wait=u32 100) -> ()  [unwired: 1 out]
            n781 = call "RS232C_SetSpeed.vi"("Low Speed"="Acquire speed (um/s)", "High Speed"="Acquire speed (um/s)", "Acceleration Time"=u16 0, "Axis Number"=w3390, "Delimiter"=w3388, "VISAリソース名"=w3394, "Axis Count"=u8 2, "Range"="Range 2", "Main/Sub"=TRUE) -> ()  [unwired: 2 out]
          }
        }
        n782 = Less?(x="# to measure", y=w3249) -> (x < y?=w3275:bool)
        n783 = Number To Decimal String(number=w3189, width (-)=i16 0) -> ()  [unwired: 1 out]
        n784 = Path To String(path=w3279) -> (string=w3235:string)
        n785 = Format Into String(format string="%04d", w3217) -> (resulting string=w3219:string)  [unwired: 2 in, 1 out]
        n786 = Or(x=w3275, y="Continuous\nacquisition") -> (x .or. y?=w3273:bool)
        n787 = Concatenate Strings(w3235, "\\temp\\" ("string"), w3241, "_" ("string"), w3219, "_" ("string")) -> (w3280:string)
        n788 = String To Path(string=w3280) -> (path=w3236:path)
        "Last saved file" <- w3236
        n789 = local read "Larvae until move"() -> (w3228:i32)
        n790 = call <userlib>:"tm_startrecorder_40.vi"("error in (no error)"=w3266, "frames"=w3260, "File"=w3236, "Handle in"=w3265) -> ("error out"=w3264:errorcluster, "Handle out"=w3263:u32)  [unwired: 6 in]
        n791 = local read "loading tube#"() -> (w3203:i32)
        n792 = call <userlib>:"tm_startcapture_40.vi"("error in (no error)"=w3264, "Handle in"=w3263) -> ("error out"=w3262:errorcluster, "Handle out"=w3261:u32)  [unwired: 8 in]
        n793 = Greater?(x=w3228, y="Larva # to move") -> (0:w3201:bool)
        n794 = Less?(x=w3203, y=7) -> (x < y?=w3200:bool)
        n795 = local write "screening"(FALSE ("screening 2")) -> ()
        n796 = And(x=w3201, y=w3200) -> (x .and. y?=w3199:bool)
        n797 = while {
          tunnel: w3269 -> [w3339]
          tunnel: w3256 -> [w3349]
          tunnel: [w3348] -> w3272
          tunnel: [w3347] -> w3283
          tunnel: [w3345] -> w3270
          tunnel: "Movement direction" -> [w3345]
          tunnel: [w3341] -> _
          tunnel: [w3340] -> _
          tunnel: [w3338] -> w3254
          stop <- w3346 stop-if-true
          # "Move to scan larva"
          n798 = flat-sequence {
            tunnel: w3345 -> [w3351]
            tunnel: w3349 -> [w3352]
            tunnel: [w3352] -> w3344
            tunnel: [w3351] -> w3343
            tunnel: [w3350] -> w3340
            tunnel: w3339 -> [_]
            tunnel: [w3365] -> w3346
            tunnel: w3339 -> [w3360]
            tunnel: w3344 -> [w3364]
            tunnel: w3343 -> [w3359]
            tunnel: [w3364] -> w3342
            tunnel: ["um to move"] -> w3338
            tunnel: [w3369] -> w3348
            tunnel: w3342 -> [w3369]
            tunnel: [w3366] -> w3341
            frame #0 {
              n799 = Wait (ms)(milliseconds to wait=u32 500) -> ()  [unwired: 1 out]
              n800 = for {
                N: 1 -> [_]
                tunnel: [w3355] -> w3350
                n801 = local read "Sub img mean"() -> (w3356:dbl)
                n802 = local read "Mean trigger"() -> (w3357:i32)
                n803 = Greater Or Equal?(x=w3356, y=w3357) -> (x >= y?=w3355:bool)
              }
            }
            frame #1 {
              w3362 = u8 2 items=["0", "1", "2", "3", "4"] ("Axis Number")
              # "Extra scan"
              n804 = call "RS232C_Move.vi"("VISAリソース名"=w3364, "Axis Count"=u8 2, "Axis Number"=w3362, "Pulse Number"="um to move", "Direction"=w3359, "Delimiter"=w3360, "Main/Sub"=FALSE) -> ("OK Done"=w3365:bool)  [unwired: 1 out]
            }
            frame #2 {
              n805 = local read "Sub img mean"() -> (w3367:dbl)
              n806 = local read "Mean trigger"() -> (w3368:i32)
              n807 = Greater?(x=w3367, y=w3368) -> (0:w3366:bool)
            }
          }
          n808 = call <extravilib>:"Write.vi"("element"=w3346) -> ("channel"=w3347:T10)  [unwired: 1 out]
        }
        n809 = while {
          tunnel: w3261 -> [w3385]
          tunnel: w3262 -> [w3384]
          tunnel: [w3381] -> w3285
          tunnel: [w3380] -> w3284
          tunnel: w3283 -> [w3383]
          tunnel: w3267 -> [w3377]
          stop <- w3382 stop-if-true
          n810 = call <userlib>:"tm_waitnextframe_40.vi"("error in (no error)"=w3384, "Handle in"=w3385) -> ("error out"=w3380:errorcluster, "Frame Count"=w3376:i32, "Frame Index"=w3379:i32, "Handle out"=w3381:u32)  [unwired: 6 in]
          n811 = call <extravilib>:"Read.vi"("channel"=w3383) -> ("element"=w3382:bool)  [unwired: 1 in, 1 out]
          n812 = local write "Frame count"(w3376) -> ()
          n813 = Index Array(array=w3377, index=w3379) -> (element=w3378:T9)
          n814 = Multiply(x=2048, y=2048) -> (x*y=w3375:i32)
          n815 = call "IMAQ ImageToArray"("Image"=w3378) -> ("Image Pixels (U16)"=w3372:u16[][])  [unwired: 3 in, 4 out]
          n816 = local write "Obtained image"(w3372) -> ()
          n817 = Reshape Array(w3372, w3375) -> (w3371:u16[])
          n818 = call-poly <vilib>:"Mean.vi"("X"=w3371) -> ("mean"=w3370:dbl)  [unwired: 1 out]
          n819 = local write "Mean intensity\nof frame"(w3370) -> ()
        }
        n820 = call <userlib>:"tm_stopcapture_40.vi"("error in (no error)"=w3284, "Handle in"=w3285) -> ("error out"=w3281:errorcluster, "Handle out"=w3282:u32)  [unwired: 8 in]
        n821 = call <userlib>:"tm_stoprecorder_40.vi"("error in (no error)"=w3281, "Handle in"=w3282) -> ("error out"=w3238:errorcluster, "Handle out"=w3240:u32)  [unwired: 8 in]
        n822 = flat-sequence {
          tunnel: w3235 -> [w3294]
          tunnel: w3236 -> [w3295]
          tunnel: w3238 -> [w3296]
          tunnel: w3240 -> [w3293]
          tunnel: [w3293] -> w3234
          tunnel: [w3296] -> w3233
          tunnel: [w3295] -> w3232
          tunnel: [w3294] -> w3231
          tunnel: [w3310] -> w3239
          tunnel: [w3309] -> w3237
          tunnel: w3234 -> [w3310]
          tunnel: w3233 -> [w3309]
          tunnel: w3232 -> [w3300]
          tunnel: w3231 -> [w3308]
          frame #0 {
            n823 = Wait (ms)(milliseconds to wait=u32 100) -> ()  [unwired: 1 out]
          }
          frame #1 {
            n824 = Path To String(path=w3300) -> (string=w3299:string)
            n825 = Strip Path(path=w3300) -> (name=w3304:string)  [unwired: 1 out]
            n826 = Concatenate Strings(w3299, ".dcimg" ("string")) -> (w3297:string)
            n827 = Concatenate Strings(w3304, ".dcimg" ("string")) -> (w3302:string)
            n828 = Concatenate Strings(w3308, "\\raw\\" ("string"), w3302) -> (w3306:string)
            n829 = String To Path(string=w3297) -> (path=w3301:path)
            n830 = String To Path(string=w3306) -> (path=w3305:path)
            n831 = Move(source path=w3301, 10:w3305) -> ()  [unwired: 3 in, 3 out]
          }
        }
        n832 = flat-sequence {
          tunnel: w3270 -> [w3320]
          tunnel: w3272 -> [w3319]
          tunnel: [w3319] -> w3259
          tunnel: [w3320] -> w3258
          tunnel: [w3318] -> w3257
          tunnel: [w3326] -> w3271
          tunnel: w3259 -> [w3326]
          tunnel: w3258 -> [w3322]
          tunnel: w3257 -> [w3325]
          tunnel: w3255 -> [_]
          tunnel: w3254 -> [_]
          tunnel: w3213 -> [w3321]
          frame #0 {
            w3312 = u8 2 items=["0", "1", "2", "3", "4"] ("Axis Number")
            w3318 = "\r\n"
            n833 = call "RS232C_SetSpeed.vi"("Low Speed"=u32 100, "High Speed"=u16 10000 ("Acceleration Time"), "Acceleration Time"=u16 100, "Axis Number"=w3312, "Delimiter"=w3318, "VISAリソース名"=w3319, "Axis Count"=u8 2, "Range"=TRUE, "Main/Sub"=TRUE) -> ()  [unwired: 2 out]
          }
          frame #1 {
            w3327 = u8 2 items=["0", "1", "2", "3", "4"] ("Axis Number")
            n834 = Wait (ms)(milliseconds to wait=u32 500) -> ()  [unwired: 1 out]
            n835 = call "RS232C_Move.vi"("VISAリソース名"=w3326, "Axis Count"=u8 2, "Axis Number"=w3327, "Pulse Number"=w3321, "Direction"=w3322, "Delimiter"=w3325, "Main/Sub"=FALSE) -> ()  [unwired: 2 out]
          }
        }
        n836 = local read "backwards pulses"() -> (w3198:i32)
        n837 = local read "scanning distance (um)"() -> (w3196:u32)
        n838 = local read "um to move"() -> (w3195:u32)
        n839 = Add(x=w3195, y=w3198) -> (x+y=w3208:u32)
        n840 = Subtract(x=w3196, y=w3208) -> (x-y=w3206:u32)
        n841 = Greater?(x=0, y=w3198) -> (0:w3207:bool)
        n842 = case shown="False" w3273 {
          tunnel: [states."Chilling" w3332] -> w3276
          tunnel: w3199 -> [_ w3331]
          tunnel: w3207 -> [_ w3330]
          frame False {
          }
          frame True {
            n843 = case shown="False" w3331 {
              tunnel: [w3334 states."auto imaging"] -> w3332
              tunnel: w3330 -> [w3333 _]
              frame False {
                n844 = case shown="True" w3333 {
                  tunnel: [states."auto imaging" states."auto imaging"] -> w3334
                  frame False {
                  }
                  frame True {
                  }
                }
              }
              frame True {
              }
            }
          }
        }
        n845 = Subtract(x=w3196, y=w3195) -> (x-y=w3194:u32)
        n846 = case shown="False" w3207 {
          tunnel: w3206 -> [w3290 _]
          tunnel: [w3290 w3291] -> w3213
          tunnel: w3194 -> [_ w3291]
          frame False {
          }
          frame True {
          }
        }
        "Last saved #" <- w3217
      }
      frame "4c acquirement" {
        w3404 = "%04d" ("format string")
        (unwired) ".dcimg" ("string")
        (unwired) i16 3 ("width (-)")
        n847 = local read "Movement direction"() -> (w3422:bool)
        n848 = Add(x=1, y=w3418) -> (x+y=w3460:i32)
        n849 = local read "Frames in memory"() -> (w3470:i32)
        n850 = flat-sequence {
          tunnel: [w3594] -> w3467
          tunnel: [w3595] -> w3476
          tunnel: [w3596] -> w3475
          tunnel: [w3588] -> w3478
          tunnel: w3492 -> [w3594]
          tunnel: w3495 -> [w3595]
          tunnel: w3494 -> [w3596]
          frame #0 {
            w3588 = "\r\n"
            w3590 = u8 2 items=["0", "1", "2", "3", "4"] ("Axis Number")
            n851 = local read "Acquire speed (um/s)"() -> (w3586:u32)
            n852 = Wait (ms)(milliseconds to wait=u32 100) -> ()  [unwired: 1 out]
            n853 = call "RS232C_SetSpeed.vi"("Low Speed"=w3586, "High Speed"=w3586, "Acceleration Time"=u16 0, "Axis Number"=w3590, "Delimiter"=w3588, "VISAリソース名"=w3594, "Axis Count"=u8 2, "Range"=FALSE, "Main/Sub"=TRUE) -> ()  [unwired: 2 out]
          }
        }
        n854 = local write "Last saved #"(w3418) -> ()
        n855 = Insert Into Array(array=w3463, index=w3460, new element=w3462) -> (w3461:string[])
        n856 = Increment(x=w3437) -> (x+1=w3436:i32)
        n857 = local read "# to measure"() -> (w3419:i32)
        n858 = Less?(x=w3419, y=w3460) -> (x < y?=w3482:bool)
        n859 = Format Into String(format string=w3404, w3401) -> (resulting string=w3403:string)  [unwired: 2 in, 1 out]
        n860 = Path To String(path=w3485) -> (string=w3447:string)
        n861 = Format Into String(format string=w3404, w3418) -> (resulting string=w3432:string)  [unwired: 2 in, 1 out]
        n862 = local read "Larva # to move"() -> (w3420:i32)
        n863 = Concatenate Strings(w3447, "\\temp\\" ("string"), "4c Base file name", "_" ("string"), w3432, "wavelength", w3403) -> (w3486:string)
        n864 = String To Path(string=w3486) -> (path=w3448:path)
        "Last saved file 4c" <- w3448
        n865 = local read "Continuous\nacquisition"() -> (w3421:bool)
        n866 = Or(x=w3482, y=w3421) -> ()  [unwired: 1 out]
        n867 = local read "Larvae until move"() -> (w3440:i32)
        n868 = call <userlib>:"tm_startrecorder_40.vi"("error in (no error)"=w3476, "frames"=w3470, "File"=w3448, "Handle in"=w3475) -> ("error out"=w3474:errorcluster, "Handle out"=w3473:u32)  [unwired: 6 in]
        n869 = call <userlib>:"tm_startcapture_40.vi"("error in (no error)"=w3474, "Handle in"=w3473) -> ("error out"=w3472:errorcluster, "Handle out"=w3471:u32)  [unwired: 8 in]
        n870 = Greater?(x=w3440, y=w3420) -> (0:w3439:bool)
        n871 = while {
          tunnel: w3478 -> [w3539]
          tunnel: w3467 -> [w3549]
          tunnel: [w3548] -> w3481
          tunnel: [w3547] -> w3489
          tunnel: [w3545] -> w3479
          tunnel: w3422 -> [w3545]
          tunnel: [w3541] -> _
          tunnel: [w3540] -> _
          tunnel: [w3538] -> w3465
          stop <- w3546 stop-if-true
          # "Move to scan larva"
          n872 = flat-sequence {
            tunnel: w3545 -> [w3551]
            tunnel: w3549 -> [w3552]
            tunnel: [w3552] -> w3544
            tunnel: [w3551] -> w3543
            tunnel: [w3550] -> w3540
            tunnel: w3539 -> [_]
            tunnel: [w3565] -> w3546
            tunnel: w3539 -> [w3560]
            tunnel: w3544 -> [w3564]
            tunnel: w3543 -> [w3559]
            tunnel: [w3564] -> w3542
            tunnel: [w3558] -> w3538
            tunnel: [w3569] -> w3548
            tunnel: w3542 -> [w3569]
            tunnel: [w3566] -> w3541
            frame #0 {
              n873 = Wait (ms)(milliseconds to wait=u32 500) -> ()  [unwired: 1 out]
              n874 = for {
                N: 1 -> [_]
                tunnel: [w3555] -> w3550
                n875 = local read "Sub img mean"() -> (w3556:dbl)
                n876 = local read "Mean trigger"() -> (w3557:i32)
                n877 = Greater Or Equal?(x=w3556, y=w3557) -> (x >= y?=w3555:bool)
              }
            }
            frame #1 {
              w3562 = u8 2 items=["0", "1", "2", "3", "4"] ("Axis Number")
              # "Extra scan"
              n878 = local read "um to move"() -> (w3558:u32)
              n879 = call "RS232C_Move.vi"("VISAリソース名"=w3564, "Axis Count"=u8 2, "Axis Number"=w3562, "Pulse Number"=w3558, "Direction"=w3559, "Delimiter"=w3560, "Main/Sub"=FALSE) -> ("OK Done"=w3565:bool)  [unwired: 1 out]
            }
            frame #2 {
              n880 = local read "Sub img mean"() -> (w3567:dbl)
              n881 = local read "Mean trigger"() -> (w3568:i32)
              n882 = Greater?(x=w3567, y=w3568) -> (0:w3566:bool)
            }
          }
          n883 = call <extravilib>:"Write.vi"("element"=w3546) -> ("channel"=w3547:T10)  [unwired: 1 out]
        }
        n884 = while {
          tunnel: w3471 -> [w3585]
          tunnel: w3472 -> [w3584]
          tunnel: [w3581] -> w3491
          tunnel: [w3580] -> w3490
          tunnel: w3489 -> [w3583]
          tunnel: w3477 -> [w3577]
          stop <- w3582 stop-if-true
          n885 = call <userlib>:"tm_waitnextframe_40.vi"("error in (no error)"=w3584, "Handle in"=w3585) -> ("error out"=w3580:errorcluster, "Frame Count"=w3576:i32, "Frame Index"=w3579:i32, "Handle out"=w3581:u32)  [unwired: 6 in]
          n886 = call <extravilib>:"Read.vi"("channel"=w3583) -> ("element"=w3582:bool)  [unwired: 1 in, 1 out]
          n887 = local write "Frame count"(w3576) -> ()
          n888 = Index Array(array=w3577, index=w3579) -> (element=w3578:T9)
          n889 = Multiply(x=2048, y=2048) -> (x*y=w3575:i32)
          n890 = call "IMAQ ImageToArray"("Image"=w3578) -> ("Image Pixels (U16)"=w3572:u16[][])  [unwired: 3 in, 4 out]
          n891 = local write "Obtained image"(w3572) -> ()
          n892 = Reshape Array(w3572, w3575) -> (w3571:u16[])
          n893 = call-poly <vilib>:"Mean.vi"("X"=w3571) -> ("mean"=w3570:dbl)  [unwired: 1 out]
          n894 = local write "Mean intensity\nof frame"(w3570) -> ()
        }
        n895 = call <userlib>:"tm_stopcapture_40.vi"("error in (no error)"=w3490, "Handle in"=w3491) -> ("error out"=w3487:errorcluster, "Handle out"=w3488:u32)  [unwired: 8 in]
        n896 = call <userlib>:"tm_stoprecorder_40.vi"("error in (no error)"=w3487, "Handle in"=w3488) -> ("error out"=w3450:errorcluster, "Handle out"=w3452:u32)  [unwired: 8 in]
        n897 = local read "Continuous\nacquisition"() -> (w3399:bool)
        n898 = flat-sequence {
          tunnel: w3447 -> [w3500]
          tunnel: w3448 -> [w3501]
          tunnel: w3450 -> [w3502]
          tunnel: w3452 -> [w3499]
          tunnel: [w3499] -> w3446
          tunnel: [w3502] -> w3445
          tunnel: [w3501] -> w3444
          tunnel: [w3500] -> w3443
          tunnel: [w3516] -> w3451
          tunnel: [w3515] -> w3449
          tunnel: w3446 -> [w3516]
          tunnel: w3445 -> [w3515]
          tunnel: w3444 -> [w3506]
          tunnel: w3443 -> [w3514]
          frame #0 {
            n899 = Wait (ms)(milliseconds to wait=u32 100) -> ()  [unwired: 1 out]
          }
          frame #1 {
            n900 = Path To String(path=w3506) -> (string=w3505:string)
            n901 = Strip Path(path=w3506) -> (name=w3510:string)  [unwired: 1 out]
            n902 = Concatenate Strings(w3505, ".dcimg" ("string")) -> (w3503:string)
            n903 = Concatenate Strings(w3510, ".dcimg" ("string")) -> (w3508:string)
            n904 = Concatenate Strings(w3514, "\\raw\\" ("string"), w3508) -> (w3512:string)
            n905 = String To Path(string=w3503) -> (path=w3507:path)
            n906 = String To Path(string=w3512) -> (path=w3511:path)
            n907 = Move(source path=w3507, 10:w3511) -> ()  [unwired: 3 in, 3 out]
          }
        }
        n908 = case shown="False" w3399 {
          tunnel: [states."homing" states."4climbo"] -> w3483
          tunnel: w3439 -> [_ _]
          frame False {
          }
          frame True {
          }
        }
        n909 = flat-sequence {
          tunnel: w3479 -> [w3517]
          tunnel: w3481 -> [w3526]
          tunnel: [w3526] -> w3469
          tunnel: [w3525] -> w3468
          tunnel: [w3517] -> w3408
          tunnel: [w3533] -> w3480
          tunnel: w3469 -> [w3533]
          tunnel: w3468 -> [w3532]
          tunnel: w3466 -> [_]
          tunnel: w3465 -> [_]
          tunnel: w3425 -> [w3529]
          tunnel: w3408 -> [w3528]
          frame #0 {
            w3519 = u8 2 items=["0", "1", "2", "3", "4"] ("Axis Number")
            w3525 = "\r\n"
            n910 = call "RS232C_SetSpeed.vi"("Low Speed"=u32 100, "High Speed"=u16 2000 ("Acceleration Time"), "Acceleration Time"=u16 100, "Axis Number"=w3519, "Delimiter"=w3525, "VISAリソース名"=w3526, "Axis Count"=u8 2, "Range"=TRUE, "Main/Sub"=TRUE) -> ()  [unwired: 2 out]
          }
          frame #1 {
            w3534 = u8 2 items=["0", "1", "2", "3", "4"] ("Axis Number")
            n911 = Not(x=w3528) -> (.not. x?=w3527:bool)
            n912 = Wait (ms)(milliseconds to wait=u32 500) -> ()  [unwired: 1 out]
            n913 = call "RS232C_Move.vi"("VISAリソース名"=w3533, "Axis Count"=u8 2, "Axis Number"=w3534, "Pulse Number"=w3529, "Direction"=w3527, "Delimiter"=w3532, "Main/Sub"=FALSE) -> ()  [unwired: 2 out]
          }
        }
        n914 = local read "backwards pulses"() -> (w3428:i32)
        n915 = local read "scanning distance (um)"() -> (w3410:u32)
        n916 = local read "um to move"() -> (w3409:u32)
        n917 = Add(x=w3409, y=w3428) -> (x+y=w3429:u32)
        n918 = Subtract(x=w3410, y=w3429) -> (x-y=w3426:u32)
        n919 = Greater?(x=0, y=w3405) -> (0:w3427:bool)
        n920 = case shown="False" w3427 {
          tunnel: w3426 -> [_ _]
          tunnel: [w3496 u32 0] -> w3425
          tunnel: w3409 -> [w3496 _]
          frame False {
          }
          frame True {
          }
        }
      }
      frame "594" {
        w3609 = TRUE ("data")
        w3610 = FALSE ("data")
        w3611 = FALSE ("data")
        w3612 = FALSE ("data")
        n921 = invoke class="StepperMotorChannel" method="SetMoveAbsolutePosition"(reference=w3616, "position"=0.3333333333333333) -> (reference out=w3621:refnum<k24>)  [unwired: 2 in, 3 out]
        n922 = local write "405 i"(w3612) -> ()
        n923 = call-poly <vilib>:"DAQmx Write.vi"("task/channels in"=w3620, "data"=w3612) -> ()  [unwired: 11 in, 3 out]
        n924 = local write "488 i"(w3611) -> ()
        n925 = call-poly <vilib>:"DAQmx Write.vi"("task/channels in"=w3619, "data"=w3611) -> ()  [unwired: 11 in, 3 out]
        n926 = local write "532 i"(w3610) -> ()
        n927 = invoke class="StepperMotorChannel" method="MoveAbsolute"(reference=w3621, "waitTimeout"=1000) -> (reference out=w3615:refnum<k24>)  [unwired: 2 in, 3 out]
        n928 = call-poly <vilib>:"DAQmx Write.vi"("task/channels in"=w3618, "data"=w3610) -> ()  [unwired: 11 in, 3 out]
        n929 = local write "594 i"(w3609) -> ()
        n930 = call-poly <vilib>:"DAQmx Write.vi"("task/channels in"=w3617, "data"=w3609) -> ()  [unwired: 11 in, 3 out]
        n931 = local read "4c direction"() -> (w3603:bool)
        n932 = local write "Movement direction"(w3603) -> ()
        n933 = local write "wavelength"("_594" ("wavelength")) -> ()
        n934 = local read "Continuous\nacquisition"() -> (w3614:bool)
        n935 = case shown="True" w3614 {
          tunnel: [states."4cini" w3651] -> w3613
          frame False {
          }
          frame True {
            n936 = case shown="False" "594?" {
              tunnel: [states."4climbo" states."4c acquirement"] -> w3651
              frame False {
              }
              frame True {
              }
            }
          }
        }
      }
      frame "532" {
        w3669 = FALSE ("data")
        w3668 = TRUE ("data")
        w3667 = FALSE ("data")
        w3666 = FALSE ("data")
        n937 = invoke class="StepperMotorChannel" method="SetMoveAbsolutePosition"(reference=w3673, "position"=0.4166667) -> (reference out=w3678:refnum<k24>)  [unwired: 2 in, 3 out]
        n938 = local write "405 i"(w3666) -> ()
        n939 = call-poly <vilib>:"DAQmx Write.vi"("task/channels in"=w3677, "data"=w3666) -> ()  [unwired: 11 in, 3 out]
        n940 = local write "488 i"(w3667) -> ()
        n941 = call-poly <vilib>:"DAQmx Write.vi"("task/channels in"=w3676, "data"=w3667) -> ()  [unwired: 11 in, 3 out]
        n942 = local write "532 i"(w3668) -> ()
        n943 = invoke class="StepperMotorChannel" method="MoveAbsolute"(reference=w3678, "waitTimeout"=2000) -> (reference out=w3672:refnum<k24>)  [unwired: 2 in, 3 out]
        n944 = call-poly <vilib>:"DAQmx Write.vi"("task/channels in"=w3675, "data"=w3668) -> ()  [unwired: 11 in, 3 out]
        n945 = local write "594 i"(w3669) -> ()
        n946 = call-poly <vilib>:"DAQmx Write.vi"("task/channels in"=w3674, "data"=w3669) -> ()  [unwired: 11 in, 3 out]
        n947 = local read "4c direction"() -> (w3660:bool)
        n948 = local write "Movement direction"(w3660) -> ()
        n949 = local write "wavelength"("_532" ("wavelength")) -> ()
        n950 = local read "Continuous\nacquisition"() -> (w3671:bool)
        n951 = case shown="True" w3671 {
          tunnel: [states."4cini" w3708] -> w3670
          frame False {
          }
          frame True {
            n952 = case shown="False" "532?" {
              tunnel: [states."4climbo" states."4c acquirement"] -> w3708
              frame False {
              }
              frame True {
              }
            }
          }
        }
      }
      frame "4cini" {
        n953 = Increment(x=w3720) -> (x+1=w3719:i32)
        n954 = local write "Movement direction"(TRUE ("Movement direction")) -> ()
        n955 = local read "position"() -> (w3717:dbl)
        n956 = invoke class="StepperMotorChannel" method="SetMoveAbsolutePosition"(reference=w3732, "position"=w3717) -> (reference out=w3737:refnum<k24>)  [unwired: 2 in, 3 out]
        n957 = invoke class="StepperMotorChannel" method="MoveAbsolute"(reference=w3737, "waitTimeout"=2000) -> (reference out=w3731:refnum<k24>)  [unwired: 2 in, 3 out]
        n958 = local read "405"() -> (w3713:bool)
        n959 = local write "405 i"(w3713) -> ()
        n960 = call-poly <vilib>:"DAQmx Write.vi"("task/channels in"=w3736, "data"=w3713) -> ()  [unwired: 11 in, 3 out]
        n961 = local read "488"() -> (w3714:bool)
        n962 = local write "488 i"(w3714) -> ()
        n963 = call-poly <vilib>:"DAQmx Write.vi"("task/channels in"=w3735, "data"=w3714) -> ()  [unwired: 11 in, 3 out]
        n964 = local read "532"() -> (w3715:bool)
        n965 = local write "532 i"(w3715) -> ()
        n966 = call-poly <vilib>:"DAQmx Write.vi"("task/channels in"=w3734, "data"=w3715) -> ()  [unwired: 11 in, 3 out]
        n967 = local read "594"() -> (w3716:bool)
        n968 = local write "594 i"(w3716) -> ()
        n969 = call-poly <vilib>:"DAQmx Write.vi"("task/channels in"=w3733, "data"=w3716) -> ()  [unwired: 11 in, 3 out]
        n970 = local write "wavelength"("532" ("wavelength")) -> ()
        n971 = local read "Continuous\nacquisition"() -> (w3730:bool)
        n972 = case shown="True" w3730 {
          tunnel: [states."homing" states."homing"] -> w3729
          frame False {
          }
          frame True {
          }
        }
      }
      frame "488" {
        w3779 = FALSE ("data")
        w3780 = FALSE ("data")
        w3781 = TRUE ("data")
        w3782 = FALSE ("data")
        n973 = invoke class="StepperMotorChannel" method="SetMoveAbsolutePosition"(reference=w3786, "position"=0.08333333333333333) -> (reference out=w3791:refnum<k24>)  [unwired: 2 in, 3 out]
        n974 = local write "405 i"(w3782) -> ()
        n975 = Wait (ms)(milliseconds to wait=u32 2000) -> ()  [unwired: 1 out]
        n976 = call-poly <vilib>:"DAQmx Write.vi"("task/channels in"=w3790, "data"=w3782) -> ()  [unwired: 11 in, 3 out]
        n977 = local write "488 i"(w3781) -> ()
        n978 = call-poly <vilib>:"DAQmx Write.vi"("task/channels in"=w3789, "data"=w3781) -> ()  [unwired: 11 in, 3 out]
        n979 = local write "532 i"(w3780) -> ()
        n980 = invoke class="StepperMotorChannel" method="MoveAbsolute"(reference=w3791, "waitTimeout"=1000) -> (reference out=w3785:refnum<k24>)  [unwired: 2 in, 3 out]
        n981 = call-poly <vilib>:"DAQmx Write.vi"("task/channels in"=w3788, "data"=w3780) -> ()  [unwired: 11 in, 3 out]
        n982 = local write "594 i"(w3779) -> ()
        n983 = call-poly <vilib>:"DAQmx Write.vi"("task/channels in"=w3787, "data"=w3779) -> ()  [unwired: 11 in, 3 out]
        n984 = local read "4c direction"() -> (w3772:bool)
        n985 = local write "Movement direction"(w3772) -> ()
        n986 = local write "wavelength"("_488" ("wavelength")) -> ()
        n987 = local read "Continuous\nacquisition"() -> (w3784:bool)
        n988 = case shown="True" w3784 {
          tunnel: [states."4cini" w3821] -> w3783
          frame False {
          }
          frame True {
            n989 = case shown="False" "488?" {
              tunnel: [states."4climbo" states."4c acquirement"] -> w3821
              frame False {
              }
              frame True {
              }
            }
          }
        }
      }
      frame "405" {
        w3836 = FALSE ("data")
        w3837 = FALSE ("data")
        w3838 = FALSE ("data")
        w3839 = TRUE ("data")
        n990 = invoke class="StepperMotorChannel" method="SetMoveAbsolutePosition"(reference=w3843, "position"=0.24999999) -> (reference out=w3848:refnum<k24>)  [unwired: 2 in, 3 out]
        n991 = local write "405 i"(w3839) -> ()
        n992 = call-poly <vilib>:"DAQmx Write.vi"("task/channels in"=w3847, "data"=w3839) -> ()  [unwired: 11 in, 3 out]
        n993 = local write "488 i"(w3838) -> ()
        n994 = call-poly <vilib>:"DAQmx Write.vi"("task/channels in"=w3846, "data"=w3838) -> ()  [unwired: 11 in, 3 out]
        n995 = local write "532 i"(w3837) -> ()
        n996 = invoke class="StepperMotorChannel" method="MoveAbsolute"(reference=w3848, "waitTimeout"=2000) -> (reference out=w3842:refnum<k24>)  [unwired: 2 in, 3 out]
        n997 = call-poly <vilib>:"DAQmx Write.vi"("task/channels in"=w3845, "data"=w3837) -> ()  [unwired: 11 in, 3 out]
        n998 = local write "594 i"(w3836) -> ()
        n999 = call-poly <vilib>:"DAQmx Write.vi"("task/channels in"=w3844, "data"=w3836) -> ()  [unwired: 11 in, 3 out]
        n1000 = local read "4c direction"() -> (w3830:bool)
        n1001 = local write "Movement direction"(w3830) -> ()
        n1002 = local write "wavelength"("_405" ("wavelength")) -> ()
        n1003 = local read "Continuous\nacquisition"() -> (w3841:bool)
        n1004 = case shown="True" w3841 {
          tunnel: [states."4cini" w3878] -> w3840
          frame False {
          }
          frame True {
            n1005 = case shown="False" "405?" {
              tunnel: [states."4climbo" states."4c acquirement"] -> w3878
              frame False {
              }
              frame True {
              }
            }
          }
        }
      }
      frame "4climbo" {
        n1006 = local read "594 i"() -> (w3887:bool)
        n1007 = local read "488 i"() -> (w3886:bool)
        n1008 = local read "405 i"() -> (w3888:bool)
        n1009 = local read "532 i"() -> (w3885:bool)
        n1010 = Boolean To (0,1)(Boolean=w3888) -> (0, 1=w3902:i16)
        n1011 = Boolean To (0,1)(Boolean=w3886) -> (0, 1=w3900:i16)
        n1012 = Boolean To (0,1)(Boolean=w3885) -> (0, 1=w3899:i16)
        n1013 = Boolean To (0,1)(Boolean=w3887) -> (0, 1=w3898:i16)
        n1014 = Initialize Array(0.0 ("element"), 3 ("dimension size")) -> (w3895:dbl[])
        n1015 = Replace Array Subset(array=w3895, new element #1=w3902, index #1=0 ("index"), new element #2=w3900, index #2=1 ("index"), new element #3=w3899, index #3=2 ("index"), new element #4=w3898, index #4=3 ("index")) -> (w3894:dbl[])
        n1016 = Search 1D Array(1D array=w3894, element=1.0, start index (0)=0) -> (index of element=w3883:i32)
        n1017 = case shown="1" w3883 {
          tunnel: [states."488" states."594" states."homing" states."4cini" states."532"] -> w3884
          frame 0 {
          }
          frame 2 {
          }
          frame 3 {
          }
          frame 4, Default {
          }
          frame 1 {
          }
        }
      }
      frame "manual_imaging" {
        # "Camera streaming during acquisition"
        n1018 = Path To String(path=w4009) -> (string=w3977:string)
        n1019 = local read "# to measure"() -> (w3968:i32)
        n1020 = Increment(x=w3958) -> (x+1=w3957:i32)
        "Last saved file number 4" <- w3957
        n1021 = Number To Decimal String(number=w3958, width (-)=i16 3) -> (decimal integer string=w3966:string)
        n1022 = local read "Frames in memory"() -> (w3994:i32)
        n1023 = local read "Movement direction"() -> (w3969:bool)
        n1024 = Insert Into Array(array=w3986, index=w3957, new element=w3985) -> (w3984:string[])
        n1025 = Concatenate Strings(w3977, w3967, w3966) -> (w4010:string)
        n1026 = Less?(x=w3968, y=w3957) -> (x < y?=w4006:bool)
        n1027 = String To Path(string=w4010) -> (path=w3978:path)
        n1028 = local read "Continuous\nacquisition"() -> (w3963:bool)
        n1029 = Or(x=w4006, y=w3963) -> (x .or. y?=w3962:bool)
        n1030 = local read "Last saved file number 4"() -> (w3974:i32)
        n1031 = flat-sequence {
          tunnel: [w4099] -> w3990
          tunnel: [w4100] -> w4000
          tunnel: [w4101] -> w3999
          tunnel: [w4093] -> w4002
          tunnel: w4016 -> [w4099]
          tunnel: w4019 -> [w4100]
          tunnel: w4018 -> [w4101]
          frame #0 {
            w4093 = "\r\n"
            w4095 = u8 2 items=["0", "1", "2", "3", "4"] ("Axis Number")
            n1032 = local read "Acquire speed (um/s)"() -> (w4091:u32)
            n1033 = Wait (ms)(milliseconds to wait=u32 200) -> ()  [unwired: 1 out]
            n1034 = call "RS232C_SetSpeed.vi"("Low Speed"=w4091, "High Speed"=w4091, "Acceleration Time"=u16 0, "Axis Number"=w4095, "Delimiter"=w4093, "VISAリソース名"=w4099, "Axis Count"=u8 2, "Range"="High speed?", "Main/Sub"=TRUE) -> ()  [unwired: 2 out]
          }
        }
        n1035 = Greater?(x=w3974, y=100) -> (0:w3972:bool)
        n1036 = case shown="True" w3962 {
          tunnel: [states."Chilling" w4042] -> w4007
          tunnel: w3972 -> [_ w4041]
          frame False {
          }
          frame True {
            n1037 = case shown="False" w4041 {
              tunnel: [states."antic\n" states."auto imaging"] -> w4042
              frame False {
              }
              frame True {
              }
            }
          }
        }
        n1038 = while {
          tunnel: w4002 -> [w4046]
          tunnel: w3990 -> [w4056]
          tunnel: [w4055] -> w4005
          tunnel: [w4054] -> w4013
          tunnel: [w4052] -> w4003
          tunnel: w3969 -> [w4052]
          tunnel: [w4048] -> _
          tunnel: [w4047] -> _
          tunnel: [w4045] -> w3988
          stop <- w4053 stop-if-true
          # "Move to scan larva"
          n1039 = flat-sequence {
            tunnel: w4052 -> [w4058]
            tunnel: w4056 -> [w4059]
            tunnel: [w4059] -> w4051
            tunnel: [w4058] -> w4050
            tunnel: [w4057] -> w4047
            tunnel: w4046 -> [_]
            tunnel: [w4072] -> w4053
            tunnel: w4046 -> [w4067]
            tunnel: w4051 -> [w4071]
            tunnel: w4050 -> [w4066]
            tunnel: [w4071] -> w4049
            tunnel: [w4065] -> w4045
            tunnel: [w4076] -> w4055
            tunnel: w4049 -> [w4076]
            tunnel: [w4073] -> w4048
            frame #0 {
              n1040 = for {
                N: 1 -> [_]
                tunnel: [w4062] -> w4057
                n1041 = local read "Sub img mean"() -> (w4063:dbl)
                n1042 = local read "Mean trigger"() -> (w4064:i32)
                n1043 = Greater Or Equal?(x=w4063, y=w4064) -> (x >= y?=w4062:bool)
              }
              n1044 = Wait (ms)(milliseconds to wait=u32 500) -> ()  [unwired: 1 out]
            }
            frame #1 {
              w4069 = u8 2 items=["0", "1", "2", "3", "4"] ("Axis Number")
              # "Extra scan"
              n1045 = local read "um to move"() -> (w4065:u32)
              n1046 = call "RS232C_Move.vi"("VISAリソース名"=w4071, "Axis Count"=u8 2, "Axis Number"=w4069, "Pulse Number"=w4065, "Direction"=w4066, "Delimiter"=w4067, "Main/Sub"=FALSE) -> ("OK Done"=w4072:bool)  [unwired: 1 out]
            }
            frame #2 {
              n1047 = local read "Sub img mean"() -> (w4074:dbl)
              n1048 = local read "Mean trigger"() -> (w4075:i32)
              n1049 = Greater?(x=w4074, y=w4075) -> (0:w4073:bool)
            }
          }
          n1050 = call <extravilib>:"Write.vi"("element"=w4053) -> ("channel"=w4054:T10)  [unwired: 1 out]
        }
        n1051 = flat-sequence {
          tunnel: w4003 -> [w4028]
          tunnel: w4005 -> [w4027]
          tunnel: [w4027] -> w3993
          tunnel: [w4028] -> w3992
          tunnel: [w4026] -> w3991
          tunnel: [w4037] -> w4004
          tunnel: w3993 -> [w4037]
          tunnel: w3992 -> [w4030]
          tunnel: w3991 -> [w4036]
          tunnel: w3989 -> [w4033]
          tunnel: w3988 -> [w4031]
          frame #0 {
            w4020 = u8 2 items=["0", "1", "2", "3", "4"] ("Axis Number")
            w4022 = u16 3000 ("Acceleration Time")
            w4026 = "\r\n"
            n1052 = call "RS232C_SetSpeed.vi"("Low Speed"=w4022, "High Speed"=w4022, "Acceleration Time"=u16 0, "Axis Number"=w4020, "Delimiter"=w4026, "VISAリソース名"=w4027, "Axis Count"=u8 2, "Range"=TRUE, "Main/Sub"=TRUE) -> ()  [unwired: 2 out]
          }
          frame #1 {
            w4038 = u8 2 items=["0", "1", "2", "3", "4"] ("Axis Number")
            n1053 = Not(x=w4030) -> (.not. x?=w4029:bool)
            n1054 = Wait (ms)(milliseconds to wait=u32 500) -> ()  [unwired: 1 out]
            n1055 = Add(x=w4031, y=w4033) -> (x+y=w4032:u32)
            n1056 = call "RS232C_Move.vi"("VISAリソース名"=w4037, "Axis Count"=u8 2, "Axis Number"=w4038, "Pulse Number"=w4032, "Direction"=w4029, "Delimiter"=w4036, "Main/Sub"=FALSE) -> ()  [unwired: 2 out]
          }
        }
        n1057 = call <userlib>:"tm_startrecorder_40.vi"("error in (no error)"=w4000, "frames"=w3994, "File"=w3978, "Handle in"=w3999) -> ("error out"=w3998:errorcluster, "Handle out"=w3997:u32)  [unwired: 6 in]
        n1058 = call <userlib>:"tm_startcapture_40.vi"("error in (no error)"=w3998, "Handle in"=w3997) -> ("error out"=w3996:errorcluster, "Handle out"=w3995:u32)  [unwired: 8 in]
        n1059 = while {
          tunnel: w3995 -> [w4090]
          tunnel: w3996 -> [w4089]
          tunnel: [w4086] -> w4015
          tunnel: [w4085] -> w4014
          tunnel: w4013 -> [w4088]
          tunnel: w4001 -> [w4082]
          stop <- w4087 stop-if-true
          n1060 = call <userlib>:"tm_waitnextframe_40.vi"("error in (no error)"=w4089, "Handle in"=w4090) -> ("error out"=w4085:errorcluster, "Frame Count"=w4081:i32, "Frame Index"=w4084:i32, "Handle out"=w4086:u32)  [unwired: 6 in]
          n1061 = call <extravilib>:"Read.vi"("channel"=w4088) -> ("element"=w4087:bool)  [unwired: 1 in, 1 out]
          n1062 = local write "Frame count"(w4081) -> ()
          n1063 = Index Array(array=w4082, index=w4084) -> (element=w4083:T9)
          n1064 = call "IMAQ ImageToArray"("Image"=w4083) -> ("Image Pixels (U16)"=w4079:u16[][])  [unwired: 3 in, 4 out]
          n1065 = local write "Obtained image"(w4079) -> ()
          n1066 = Reshape Array(w4079, 4194304 ("dimension size")) -> (w4078:u16[])
          n1067 = call-poly <vilib>:"Mean.vi"("X"=w4078) -> ("mean"=w4077:dbl)  [unwired: 1 out]
          n1068 = local write "Mean intensity\nof frame"(w4077) -> ()
        }
        n1069 = call <userlib>:"tm_stopcapture_40.vi"("error in (no error)"=w4014, "Handle in"=w4015) -> ("error out"=w4011:errorcluster, "Handle out"=w4012:u32)  [unwired: 8 in]
        n1070 = call <userlib>:"tm_stoprecorder_40.vi"("error in (no error)"=w4011, "Handle in"=w4012) -> ("error out"=w3970:errorcluster, "Handle out"=w3971:u32)  [unwired: 8 in]
      }
      frame "4000" {
        (unwired) 0.0 ("new element/subarray")
        # "Set stage speed for acquisition"
        n1071 = local read "Frames in memory"() -> (w4172:i32)
        n1072 = Path To String(path=w4160) -> (string=w4194:string)
        n1073 = Number To Decimal String(number=w4141, width (-)=i16 3) -> (decimal integer string=w4164:string)
        n1074 = Add(x=1, y=w4141) -> (x+y=w4125:i32)
        "Last saved file number 4000" <- w4125
        n1075 = local read "Movement direction"() -> (w4137:bool)
        n1076 = Concatenate Strings(w4194, w4164) -> (w4193:string)
        n1077 = flat-sequence {
          tunnel: [w4282] -> w4168
          tunnel: [w4283] -> w4178
          tunnel: [w4284] -> w4177
          tunnel: [w4276] -> w4180
          tunnel: w4200 -> [w4282]
          tunnel: w4203 -> [w4283]
          tunnel: w4202 -> [w4284]
          frame #0 {
            w4276 = "\r\n"
            w4278 = u8 2 items=["0", "1", "2", "3", "4"] ("Axis Number")
            n1078 = Wait (ms)(milliseconds to wait=u32 500) -> ()  [unwired: 1 out]
            n1079 = call "RS232C_SetSpeed.vi"("Low Speed"="Acquire speed 2 (um/s)", "High Speed"="Acquire speed 2 (um/s)", "Acceleration Time"=u16 0, "Axis Number"=w4278, "Delimiter"=w4276, "VISAリソース名"=w4282, "Axis Count"=u8 2, "Range"=TRUE, "Main/Sub"=FALSE) -> ("OK Done"=→"OK Done 4":bool)  [unwired: 1 out]
          }
        }
        n1080 = String To Path(string=w4193) -> (path=w4148:path)
        "Last saved file 4000" <- w4148
        n1081 = call <userlib>:"tm_startrecorder_40.vi"("error in (no error)"=w4178, "frames"=w4172, "File"=w4148, "Handle in"=w4177) -> ("error out"=w4176:errorcluster, "Handle out"=w4175:u32)  [unwired: 6 in]
        n1082 = Initialize Array("", 1000 ("dimension size")) -> (w4155:string[])
        n1083 = call <userlib>:"tm_startcapture_40.vi"("error in (no error)"=w4176, "Handle in"=w4175) -> ("error out"=w4174:errorcluster, "Handle out"=w4173:u32)  [unwired: 8 in]
        n1084 = Less?(x="Samples to measure 2", y=w4125) -> (x < y?=w4188:bool)
        n1085 = Insert Into Array(array=w4155, index=w4125, new element=w4163) -> ()  [unwired: 1 out]
        n1086 = Or(x=w4188, y="GS speed 2") -> (x .or. y?=w4186:bool)
        n1087 = case shown="False" w4186 {
          tunnel: [states."Chilling" w4232] -> w4189
          tunnel: "calibration?" -> [_ w4231]
          frame False {
          }
          frame True {
            n1088 = case shown="True" w4231 {
              tunnel: [states."Acquire" states."homing"] -> w4232
              frame False {
              }
              frame True {
              }
            }
          }
        }
        n1089 = while {
          tunnel: w4180 -> [w4236]
          tunnel: w4168 -> [w4244]
          tunnel: [w4243] -> w4185
          tunnel: [w4242] -> w4197
          tunnel: [w4240] -> w4183
          tunnel: w4137 -> [w4240]
          tunnel: [w4235] -> w4166
          stop <- w4241 stop-if-true
          # "Move to scan larva"
          n1090 = flat-sequence {
            tunnel: w4240 -> [w4245]
            tunnel: w4244 -> [w4246]
            tunnel: [w4246] -> w4239
            tunnel: [w4245] -> w4238
            tunnel: w4236 -> [_]
            tunnel: [w4255] -> w4241
            tunnel: w4236 -> [w4250]
            tunnel: w4239 -> [w4254]
            tunnel: w4238 -> [w4249]
            tunnel: [w4254] -> w4237
            tunnel: [w4248] -> w4235
            tunnel: [w4256] -> w4243
            tunnel: w4237 -> [w4256]
            frame #0 {
              n1091 = Wait (ms)(milliseconds to wait=u32 500) -> ()  [unwired: 1 out]
            }
            frame #1 {
              w4252 = u8 2 items=["0", "1", "2", "3", "4"] ("Axis Number")
              # "Extra scan"
              n1092 = local read "um to move"() -> (w4248:u32)
              n1093 = call "RS232C_Move.vi"("VISAリソース名"=w4254, "Axis Count"=u8 2, "Axis Number"=w4252, "Pulse Number"=w4248, "Direction"=w4249, "Delimiter"=w4250, "Main/Sub"=FALSE) -> ("OK Done"=w4255:bool)  [unwired: 1 out]
            }
            frame #2 {
            }
          }
          n1094 = call <extravilib>:"Write.vi"("element"=w4241) -> ("channel"=w4242:T10)  [unwired: 1 out]
        }
        n1095 = Initialize Array(0.0 ("element"), 200 ("dimension size"), 2048 ("dimension size"), 2048 ("dimension size")) -> (w4152:dbl[][][])
        n1096 = while {
          tunnel: w4173 -> [w4272]
          tunnel: w4174 -> [w4271]
          tunnel: [w4268] -> w4199
          tunnel: [w4267] -> w4198
          tunnel: w4197 -> [w4270]
          tunnel: w4179 -> [w4264]
          shift-right: [w4262] -> w4151
          shift-left: w4152 -> [w4263]
          stop <- w4269 stop-if-true
          n1097 = call <extravilib>:"Read.vi"("channel"=w4270) -> ("element"=w4269:bool)  [unwired: 1 in, 1 out]
          n1098 = call <userlib>:"tm_waitnextframe_40.vi"("error in (no error)"=w4271, "Handle in"=w4272) -> ("error out"=w4267:errorcluster, "Frame Count"=w4261:i32, "Frame Index"=w4266:i32, "Handle out"=w4268:u32)  [unwired: 6 in]
          n1099 = Index Array(array=w4264, index=w4266) -> (element=w4265:T9)
          n1100 = local write "Frame count"(w4261) -> ()
          n1101 = call "IMAQ ImageToArray"("Image"=w4265) -> ("Image Pixels (U16)"=w4259:u16[][])  [unwired: 3 in, 4 out]
          n1102 = local write "Obtained image"(w4259) -> ()
          n1103 = Reshape Array(w4259, 4194304 ("dimension size")) -> (w4260:u16[])
          n1104 = Replace Array Subset(array=w4263, new element=w4259, index (dim 0)=w4261) -> (w4262:dbl[][][])  [unwired: 2 in]
          n1105 = call-poly <vilib>:"Mean.vi"("X"=w4260) -> ("mean"=w4258:dbl)  [unwired: 1 out]
          n1106 = local write "Mean intensity\nof frame"(w4258) -> ()
        }
        n1107 = local write "screening"(TRUE ("screening")) -> ()
        n1108 = flat-sequence {
          tunnel: w4183 -> [w4220]
          tunnel: w4185 -> [w4219]
          tunnel: [w4219] -> w4171
          tunnel: [w4220] -> w4170
          tunnel: [w4218] -> w4169
          tunnel: [w4227] -> w4184
          tunnel: w4171 -> [w4227]
          tunnel: w4170 -> [w4223]
          tunnel: w4169 -> [w4226]
          tunnel: w4166 -> [w4221]
          frame #0 {
            w4212 = u8 2 items=["0", "1", "2", "3", "4"] ("Axis Number")
            w4214 = u16 2000 ("Acceleration Time")
            w4218 = "\r\n"
            n1109 = call "RS232C_SetSpeed.vi"("Low Speed"=w4214, "High Speed"=w4214, "Acceleration Time"=u16 0, "Axis Number"=w4212, "Delimiter"=w4218, "VISAリソース名"=w4219, "Axis Count"=u8 2, "Range"=TRUE, "Main/Sub"=FALSE) -> ()  [unwired: 2 out]
          }
          frame #1 {
            w4228 = u8 2 items=["0", "1", "2", "3", "4"] ("Axis Number")
            n1110 = Not(x=w4223) -> (.not. x?=w4222:bool)
            n1111 = Wait (ms)(milliseconds to wait=u32 500) -> ()  [unwired: 1 out]
            n1112 = call "RS232C_Move.vi"("VISAリソース名"=w4227, "Axis Count"=u8 2, "Axis Number"=w4228, "Pulse Number"=w4221, "Direction"=w4222, "Delimiter"=w4226, "Main/Sub"=FALSE) -> ()  [unwired: 2 out]
          }
        }
        n1113 = for {
          tunnel: w4151 -> [w4211] mode=indexing
          tunnel: [w4206] -> w4136 mode=indexing
          tunnel: [w4204] -> _ mode=indexing
          workers-P: _ -> [_]
          tunnel: [w4204] -> _ mode=indexing
          w4210 = 2048 ("dimension size")
          n1114 = Multiply(x=w4210, y=w4210) -> (x*y=w4209:i32)
          n1115 = Reshape Array(w4211, w4209) -> (w4208:dbl[])
          n1116 = call-poly <vilib>:"Mean.vi"("X"=w4208) -> ("mean"=w4204:dbl)  [unwired: 1 out]
          n1117 = Greater?(x=w4204, y="wave trigger") -> (0:w4207:bool)
          n1118 = Boolean To (0,1)(Boolean=w4207) -> (0, 1=w4206:i16)
        }
        n1119 = call <userlib>:"tm_stopcapture_40.vi"("error in (no error)"=w4198, "Handle in"=w4199) -> ("error out"=w4195:errorcluster, "Handle out"=w4196:u32)  [unwired: 8 in]
        n1120 = call <userlib>:"tm_stoprecorder_40.vi"("error in (no error)"=w4195, "Handle in"=w4196) -> ("error out"=w4181:errorcluster, "Handle out"=w4182:u32)  [unwired: 8 in]
        n1121 = call-poly <vilib>:"Write Waveforms to File.vi"("waveform"=w4136, "file path (dialog if empty)"=w4148) -> ()  [unwired: 8 in, 2 out]
        n1122 = Reverse 1D Array(array=w4136) -> (reversed array=w4146:i16[])
        n1123 = Search 1D Array(1D array=w4136, element=i16 1) -> (index of element=w4135:i32)  [unwired: 1 in]
        n1124 = Search 1D Array(1D array=w4146, element=i16 1) -> (index of element=w4143:i32)  [unwired: 1 in]
        n1125 = Initialize Array(0.0 ("element"), 1000 ("dimension size")) -> (w4126:dbl[])
        n1126 = Add(x=w4135, y=w4143) -> (x+y=w4144:i32)
        n1127 = Subtract(x=200, y=w4144) -> (x-y=w4134:i32)
        n1128 = Array Subset(array=w4126, index=w4135, length=w4134) -> (w4133:dbl[])
        n1129 = Insert Into Array(array=w4139, index=w4125, new element=w4134) -> (w4138:i16[])
        n1130 = call-poly <vilib>:"Mean.vi"("X"=w4133) -> ("mean"=w4123:dbl)  [unwired: 1 out]
        n1131 = Insert Into Array(array=w4124, index=w4125, new element=w4123) -> (w4122:dbl[])
        n1132 = call <vilib>:"High Resolution Relative Seconds.vi"() -> ("relative seconds"=w4102:dbl)
      }
      frame "screening" {
        n1133 = case shown="False" "go to 2000?" {
          tunnel: [w4343 w4345] -> w4299
          tunnel: [w4342 w4344] -> w4286
          frame False {
            n1134 = local read "Last saved file 4000"() -> (w4343:path)
            n1135 = call <vilib>:"High Resolution Relative Seconds.vi"() -> ("relative seconds"=w4342:dbl)
          }
          frame True {
            n1136 = local read "Last saved file 2000"() -> (w4349:path)
            n1137 = call <vilib>:"High Resolution Relative Seconds.vi"() -> ("relative seconds"=w4344:dbl)
            n1138 = Path To String(path=w4349) -> (string=w4348:string)
            n1139 = Concatenate Strings(w4348, ".dcimg" ("string")) -> (w4346:string)
            n1140 = String To Path(string=w4346) -> (path=w4345:path)
          }
        }
        n1141 = case shown="\"MAX INTENSITY\"" "screening method" {
          tunnel: w4299 -> [w4355 w4386 w4420 w4459]
          tunnel: [w4354 _ _ _] -> _
          tunnel: [w4353 w4385 _ _] -> _
          tunnel: [FALSE FALSE w4418 w4458] -> w4295
          tunnel: [w4350 w4382 w4417 w4457] -> w4287
          frame "Pix count" {
            n1142 = for {
              N: 0 -> [_]
              tunnel: w4355 -> [w4364]
              tunnel: [w4356] -> w4353 mode=indexing
              tunnel: [w4359] -> w4354 mode=indexing
              n1143 = call <userlib>:"tm_opendcimgfile_40.vi"("Path"=w4364) -> ("error out"=w4366:errorcluster, "Total Frames"=w4357:i32, "File Handle"=w4367:u32)  [unwired: 8 in]
              n1144 = for {
                N: w4357 -> [_]
                tunnel: w4367 -> [w4378]
                tunnel: w4366 -> [w4377]
                tunnel: [w4376] -> w4365
                tunnel: [w4374] -> w4363
                tunnel: [w4371] -> w4362 mode=indexing
                i -> [w4375]
                n1145 = call <userlib>:"tm_getdcimgframe.vi"("error in (no error)"=w4377, "Frame Index"=w4375, "File Handle in"=w4378) -> ("error out"=w4376:errorcluster, "Data"=w4373:u16[][], "File Handle out"=w4374:u32)  [unwired: 5 in, 1 out]
                n1146 = for {
                  tunnel: w4373 -> [w4379] mode=indexing
                  tunnel: [w4380] -> w4372 mode=indexing
                  workers-P: 36 -> [_]
                  n1147 = call <vilib>:"Threshold Detector.vi"("width"=1, "X"=w4379) -> ("count"=w4380:i32)  [unwired: 1 in, 2 out]
                }
                n1148 = Add Array Elements(numeric array=w4372) -> (sum=w4371:i32)
              }
              n1149 = call <userlib>:"tm_closedcimgfile_40.vi"("error in (no error)"=w4365, "File Handle"=w4363) -> ()  [unwired: 9 in, 1 out]
              n1150 = Add Array Elements(numeric array=w4362) -> (sum=w4358:i32)
              n1151 = Divide(x=w4358, y=w4357) -> (x/y=w4356:dbl)
              n1152 = Greater?(x=w4356, y=9000 ("x")) -> (0:w4360:bool)
              n1153 = case shown="True" w4360 {
                tunnel: [1 ("index") 2 ("index")] -> w4359
                frame False {
                  # "PURE NON TUBBY"
                }
                frame True {
                  # "TUBBY"
                }
              }
            }
            n1154 = call <vilib>:"High Resolution Relative Seconds.vi"() -> ("relative seconds"=w4350:dbl)
          }
          frame "Average int" {
            n1155 = for {
              N: 0 -> [_]
              tunnel: w4386 -> [w4393]
              tunnel: [w4390] -> _ mode=indexing
              tunnel: [w4389] -> _ mode=indexing
              tunnel: [w4387] -> w4385 mode=indexing
              n1156 = call <userlib>:"tm_opendcimgfile_40.vi"("Path"=w4393) -> ("error out"=w4395:errorcluster, "Total Frames"=w4392:i32, "File Handle"=w4396:u32)  [unwired: 8 in]
              n1157 = for {
                N: w4392 -> [_]
                tunnel: w4396 -> [w4407]
                tunnel: w4395 -> [w4406]
                tunnel: [w4405] -> w4394
                tunnel: [w4403] -> w4391
                tunnel: [w4400] -> w4389 mode=indexing
                tunnel: [w4399] -> w4388 mode=indexing
                i -> [w4404]
                n1158 = call <userlib>:"tm_getdcimgframe.vi"("error in (no error)"=w4406, "Frame Index"=w4404, "File Handle in"=w4407) -> ("error out"=w4405:errorcluster, "Data"=w4402:u16[][], "File Handle out"=w4403:u32)  [unwired: 5 in, 1 out]
                n1159 = for {
                  tunnel: w4402 -> [w4411] mode=indexing
                  tunnel: [w4412] -> w4401 mode=indexing
                  workers-P: 36 -> [_]
                  tunnel: [w4409] -> w4397 mode=indexing
                  n1160 = call <vilib>:"Threshold Detector.vi"("width"=1, "X"=w4411) -> ("count"=w4412:i32, "Indices"=w4410:i32[])  [unwired: 1 in, 1 out]
                  n1161 = for {
                    tunnel: w4411 -> [w4416]
                    tunnel: w4410 -> [w4415] mode=indexing
                    tunnel: [w4414] -> w4408 mode=indexing
                    n1162 = Index Array(array=w4416, index=w4415) -> (element=w4414:u16)
                  }
                  n1163 = Array Size(array=w4408) -> ()  [unwired: 1 out]
                  n1164 = call-poly <vilib>:"Mean.vi"("X"=w4408) -> ("mean"=w4409:dbl)  [unwired: 1 out]
                }
                n1165 = call-poly <vilib>:"Mean.vi"("X"=w4397) -> ("mean"=w4399:dbl)  [unwired: 1 out]
                n1166 = Add Array Elements(numeric array=w4401) -> (sum=w4400:i32)
              }
              n1167 = call <userlib>:"tm_closedcimgfile_40.vi"("error in (no error)"=w4394, "File Handle"=w4391) -> ()  [unwired: 9 in, 1 out]
              n1168 = Add Array Elements(numeric array=w4389) -> (sum=w4390:i32)
              n1169 = call-poly <vilib>:"Mean.vi"("X"=w4388) -> ("mean"=w4387:dbl)  [unwired: 1 out]
            }
            n1170 = call <vilib>:"High Resolution Relative Seconds.vi"() -> ("relative seconds"=w4382:dbl)
          }
          frame "MAX INTENSITY" {
            n1171 = call <userlib>:"tm_opendcimgfile_40.vi"("Path"=w4420) -> ("error out"=w4425:errorcluster, "Total Frames"=w4426:i32, "File Handle"=w4424:u32)  [unwired: 8 in]
            n1172 = for {
              N: w4426 -> [_]
              tunnel: w4424 -> [w4456]
              tunnel: w4425 -> [w4455]
              tunnel: [w4454] -> _
              tunnel: [w4450] -> w4431
              tunnel: [w4444] -> w4429 mode=indexing
              workers-P: _ -> [_]
              i -> [w4453]
              n1173 = Multiply(x=2048.0, y=2048.0) -> (x*y=w4442:dbl)
              n1174 = call <userlib>:"tm_getdcimgframe.vi"("error in (no error)"=w4455, "Frame Index"=w4453, "File Handle in"=w4456) -> ("error out"=w4454:errorcluster, "Data"=w4443:u16[][], "File Handle out"=w4450:u32)  [unwired: 5 in, 1 out]
              n1175 = Reshape Array(w4443, w4442) -> (w4441:u16[])
              n1176 = call "Sort 1D Array.vim"("unsorted array"=w4441) -> ("sorted array"=w4449:u16[])  [unwired: 10 in]
              n1177 = Reverse 1D Array(array=w4449) -> (reversed array=w4448:u16[])
              n1178 = Array Subset(array=w4448, index=0, length=5) -> (w4445:u16[])
              n1179 = call-poly <vilib>:"Mean.vi"("X"=w4445) -> ("mean"=w4444:dbl)  [unwired: 1 out]
            }
            n1180 = call "Sort 1D Array.vim"("unsorted array"=w4429) -> ("sorted array"=w4430:dbl[])  [unwired: 10 in]
            n1181 = Reverse 1D Array(array=w4430) -> (reversed array=w4427:dbl[])
            n1182 = Array Subset(array=w4427, index=0, length=5) -> (w4428:dbl[])
            n1183 = call-poly <vilib>:"Mean.vi"("X"=w4428) -> ("mean"=w4419:dbl)  [unwired: 1 out]
            n1184 = Greater?(x="max intensity\n threshold", y=w4419) -> (0:w4418:bool)
            n1185 = case shown="True" w4418 {
              tunnel: [1 ("index") 2 ("index")] -> _
              tunnel: w4431 -> [w4434 w4439]
              tunnel: [w4434 w4439] -> w4432
              tunnel: [w4433 w4437] -> w4417
              frame False {
                # "PURE NON TUBBY"
                n1186 = Wait (ms)(milliseconds to wait=u32 5) -> ()  [unwired: 1 out]
                n1187 = call <vilib>:"High Resolution Relative Seconds.vi"() -> ("relative seconds"=w4433:dbl)
              }
              frame True {
                # "TUBBY"
                n1188 = Wait (ms)(milliseconds to wait=u32 5) -> ()  [unwired: 1 out]
                n1189 = call <vilib>:"High Resolution Relative Seconds.vi"() -> ("relative seconds"=w4437:dbl)
              }
            }
            n1190 = call <userlib>:"tm_closedcimgfile_40.vi"("File Handle"=w4432) -> ()  [unwired: 10 in, 1 out]
          }
          frame "morphology" {
            w4461 = 0 ("start index (0)")
            w4467 = i16 1 ("element")
            n1191 = call <userlib>:"tm_opendcimgfile_40.vi"("Path"=w4459) -> ("error out"=w4472:errorcluster, "Total Frames"=w4464:i32, "File Handle"=w4471:u32)  [unwired: 8 in]
            n1192 = for {
              N: w4464 -> [_]
              tunnel: w4471 -> [w4501]
              tunnel: w4472 -> [w4500]
              tunnel: [w4499] -> _
              tunnel: [w4495] -> w4473
              tunnel: [w4483] -> w4469 mode=indexing
              workers-P: 6 -> [_]
              i -> [w4498]
              n1193 = Multiply(x=2048.0, y=2048.0) -> (x*y=w4488:dbl)
              n1194 = call <userlib>:"tm_getdcimgframe.vi"("error in (no error)"=w4500, "Frame Index"=w4498, "File Handle in"=w4501) -> ("error out"=w4499:errorcluster, "Data"=w4489:u16[][], "File Handle out"=w4495:u32)  [unwired: 5 in, 1 out]
              n1195 = Reshape Array(w4489, w4488) -> (w4487:u16[])
              n1196 = call "Sort 1D Array.vim"("unsorted array"=w4487) -> ("sorted array"=w4494:u16[])  [unwired: 10 in]
              n1197 = Reverse 1D Array(array=w4494) -> (reversed array=w4493:u16[])
              n1198 = Array Subset(array=w4493, index=0, length=4194304) -> (w4490:u16[])
              n1199 = call-poly <vilib>:"Mean.vi"("X"=w4490) -> ("mean"=w4486:dbl)  [unwired: 1 out]
              "mean" <- w4486
              n1200 = Greater?(x=w4486, y="morphology\nthreshold 2") -> (0:w4484:bool)
              n1201 = Boolean To (0,1)(Boolean=w4484) -> (0, 1=w4483:i16)
            }
            n1202 = Reverse 1D Array(array=w4469) -> (reversed array=w4468:i16[])
            n1203 = Search 1D Array(1D array=w4469, element=w4467, start index (0)=w4461) -> (index of element=w4466:i32)
            n1204 = Search 1D Array(1D array=w4468, element=w4467, start index (0)=w4461) -> (index of element=w4465:i32)
            n1205 = Add(x=w4466, y=w4465) -> (x+y=w4463:i32)
            n1206 = Subtract(x=w4464, y=w4463) -> (x-y=w4462:i32)
            n1207 = Greater?(x="morphology\nthreshold 1", y=w4462) -> (0:w4458:bool)
            n1208 = case shown="False" w4458 {
              tunnel: [1 ("index") 2 ("index")] -> _
              tunnel: w4473 -> [w4476 w4481]
              tunnel: [w4476 w4481] -> w4474
              tunnel: [w4475 w4479] -> w4457
              frame False {
                # "PURE NON TUBBY"
                n1209 = Wait (ms)(milliseconds to wait=u32 5) -> ()  [unwired: 1 out]
                n1210 = call <vilib>:"High Resolution Relative Seconds.vi"() -> ("relative seconds"=w4475:dbl)
              }
              frame True {
                # "TUBBY"
                n1211 = Wait (ms)(milliseconds to wait=u32 5) -> ()  [unwired: 1 out]
                n1212 = call <vilib>:"High Resolution Relative Seconds.vi"() -> ("relative seconds"=w4479:dbl)
              }
            }
            n1213 = call <userlib>:"tm_closedcimgfile_40.vi"("File Handle"=w4474) -> ()  [unwired: 10 in, 1 out]
          }
        }
        n1214 = Subtract(x=w4287, y=w4286) -> (x-y=→"morphology \nscreening time":dbl)
        n1215 = case shown="True" w4295 {
          tunnel: [states."Acquire" states."homing"] -> w4296
          tunnel: [w4333 w4340] -> _
          tunnel: [w4332 w4337] -> w4288
          frame False {
            n1216 = call <vilib>:"High Resolution Relative Seconds.vi"() -> ("relative seconds"=w4332:dbl)
            n1217 = Wait (ms)(milliseconds to wait=u32 500) -> ()  [unwired: 1 out]
            n1218 = call <vilib>:"High Resolution Relative Seconds.vi"() -> ("relative seconds"=w4333:dbl)
            n1219 = local write "screening"(FALSE ("screening 2")) -> ()
          }
          frame True {
            n1220 = call <vilib>:"High Resolution Relative Seconds.vi"() -> ("relative seconds"=w4337:dbl)
            n1221 = call <vilib>:"High Resolution Relative Seconds.vi"() -> ("relative seconds"=w4340:dbl)
            n1222 = Wait (ms)(milliseconds to wait=u32 500) -> ()  [unwired: 1 out]
            n1223 = local write "screening"(TRUE ("screening 2")) -> ()
          }
        }
        n1224 = Subtract(x=w4288, y=w4290) -> (x-y=→"screening time":dbl)
        "screening" <- FALSE ("screening 2")
      }
      frame "2000" {
        # "Camera streaming during acquisition"
        n1225 = local read "Last saved file number 2000"() -> (w4559:i32)
        n1226 = local read "Frames in memory"() -> (w4573:i32)
        n1227 = local read "Movement direction"() -> (w4538:bool)
        n1228 = Add(x=1, y=w4506) -> (x+y=w4527:i32)
        n1229 = Initialize Array("", 1000 ("dimension size")) -> (w4553:string[])
        n1230 = Number To Decimal String(number=w4506, width (-)=i16 3) -> (decimal integer string=w4563:string)
        n1231 = Insert Into Array(array=w4553, index=w4527, new element=w4562) -> ()  [unwired: 1 out]
        n1232 = Less?(x="Samples to measure 3", y=w4506) -> (x < y?=w4589:bool)
        n1233 = Or(x=w4589, y="GS speed 3") -> (x .or. y?=w4587:bool)
        n1234 = flat-sequence {
          tunnel: [w4696] -> w4569
          tunnel: [w4697] -> w4579
          tunnel: [w4698] -> w4578
          tunnel: [w4690] -> w4581
          tunnel: w4601 -> [w4696]
          tunnel: w4604 -> [w4697]
          tunnel: w4603 -> [w4698]
          frame #0 {
            w4690 = "\r\n"
            w4692 = u8 2 items=["0", "1", "2", "3", "4"] ("Axis Number")
            n1235 = Wait (ms)(milliseconds to wait=u32 500) -> ()  [unwired: 1 out]
            n1236 = call "RS232C_SetSpeed.vi"("Low Speed"="Acquire speed 3 (um/s)", "High Speed"="Acquire speed 3 (um/s)", "Acceleration Time"=u16 0, "Axis Number"=w4692, "Delimiter"=w4690, "VISAリソース名"=w4696, "Axis Count"=u8 2, "Range"=TRUE, "Main/Sub"=FALSE) -> ()  [unwired: 2 out]
          }
        }
        n1237 = Path To String(path="Save base file name 2000") -> (string=w4595:string)
        n1238 = Concatenate Strings(w4595, w4563) -> (w4594:string)
        n1239 = String To Path(string=w4594) -> (path=w4546:path)
        "Last saved file 2000" <- w4546
        n1240 = call <userlib>:"tm_startrecorder_40.vi"("error in (no error)"=w4579, "frames"=w4573, "File"=w4546, "Handle in"=w4578) -> ("error out"=w4577:errorcluster, "Handle out"=w4576:u32)  [unwired: 6 in]
        n1241 = call <userlib>:"tm_startcapture_40.vi"("error in (no error)"=w4577, "Handle in"=w4576) -> ("error out"=w4575:errorcluster, "Handle out"=w4574:u32)  [unwired: 8 in]
        n1242 = Initialize Array(0.0 ("element"), 200 ("dimension size"), 2048 ("dimension size"), 2048 ("dimension size")) -> (w4550:dbl[][][])
        n1243 = while {
          tunnel: w4581 -> [w4641]
          tunnel: w4569 -> [w4651]
          tunnel: [w4650] -> w4586
          tunnel: [w4649] -> w4598
          tunnel: [w4647] -> w4584
          tunnel: w4538 -> [w4647]
          tunnel: [w4643] -> _
          tunnel: [w4642] -> w4566
          tunnel: [w4640] -> w4568
          stop <- w4648 stop-if-true
          # "Move to scan larva"
          n1244 = flat-sequence {
            tunnel: w4647 -> [w4653]
            tunnel: w4651 -> [w4654]
            tunnel: [w4654] -> w4646
            tunnel: [w4653] -> w4645
            tunnel: [w4652] -> w4642
            tunnel: w4641 -> [_]
            tunnel: [w4667] -> w4648
            tunnel: w4641 -> [w4662]
            tunnel: w4646 -> [w4666]
            tunnel: w4645 -> [w4661]
            tunnel: [w4666] -> w4644
            tunnel: [w4660] -> w4640
            tunnel: [w4671] -> w4650
            tunnel: w4644 -> [w4671]
            tunnel: [w4668] -> w4643
            frame #0 {
              n1245 = Wait (ms)(milliseconds to wait=u32 500) -> ()  [unwired: 1 out]
              n1246 = for {
                N: 1 -> [_]
                tunnel: [w4657] -> w4652
                n1247 = local read "Sub img mean"() -> (w4658:dbl)
                n1248 = local read "Mean trigger"() -> (w4659:i32)
                n1249 = Greater Or Equal?(x=w4658, y=w4659) -> (x >= y?=w4657:bool)
              }
            }
            frame #1 {
              w4664 = u8 2 items=["0", "1", "2", "3", "4"] ("Axis Number")
              # "Extra scan"
              n1250 = local read "um to move"() -> (w4660:u32)
              n1251 = call "RS232C_Move.vi"("VISAリソース名"=w4666, "Axis Count"=u8 2, "Axis Number"=w4664, "Pulse Number"=w4660, "Direction"=w4661, "Delimiter"=w4662, "Main/Sub"=FALSE) -> ("OK Done"=w4667:bool)  [unwired: 1 out]
            }
            frame #2 {
              n1252 = local read "Sub img mean"() -> (w4669:dbl)
              n1253 = local read "Mean trigger"() -> (w4670:i32)
              n1254 = Greater?(x=w4669, y=w4670) -> (0:w4668:bool)
            }
          }
          n1255 = call <extravilib>:"Write.vi"("element"=w4648) -> ("channel"=w4649:T10)  [unwired: 1 out]
        }
        n1256 = while {
          tunnel: w4574 -> [w4687]
          tunnel: w4575 -> [w4686]
          tunnel: [w4683] -> w4600
          tunnel: [w4682] -> w4599
          tunnel: w4598 -> [w4685]
          tunnel: w4580 -> [w4679]
          shift-right: [w4677] -> w4549
          shift-left: w4550 -> [w4678]
          stop <- w4684 stop-if-true
          n1257 = call <extravilib>:"Read.vi"("channel"=w4685) -> ("element"=w4684:bool)  [unwired: 1 in, 1 out]
          n1258 = call <userlib>:"tm_waitnextframe_40.vi"("error in (no error)"=w4686, "Handle in"=w4687) -> ("error out"=w4682:errorcluster, "Frame Count"=w4676:i32, "Frame Index"=w4681:i32, "Handle out"=w4683:u32)  [unwired: 6 in]
          n1259 = Index Array(array=w4679, index=w4681) -> (element=w4680:T9)
          n1260 = call "IMAQ ImageToArray"("Image"=w4680) -> ("Image Pixels (U16)"=w4674:u16[][])  [unwired: 3 in, 4 out]
          n1261 = local write "Frame count"(w4676) -> ()
          n1262 = Reshape Array(w4674, 4194304) -> (w4675:u16[])
          n1263 = local write "Obtained image"(w4674) -> ()
          n1264 = Replace Array Subset(array=w4678, new element=w4674, index (dim 0)=w4676) -> (w4677:dbl[][][])  [unwired: 2 in]
          n1265 = call-poly <vilib>:"Mean.vi"("X"=w4675) -> ("mean"=w4673:dbl)  [unwired: 1 out]
          n1266 = local write "Mean intensity\nof frame"(w4673) -> ()
        }
        n1267 = call <userlib>:"tm_stopcapture_40.vi"("error in (no error)"=w4599, "Handle in"=w4600) -> ("error out"=w4596:errorcluster, "Handle out"=w4597:u32)  [unwired: 8 in]
        n1268 = call <userlib>:"tm_stoprecorder_40.vi"("error in (no error)"=w4596, "Handle in"=w4597) -> ("error out"=w4582:errorcluster, "Handle out"=w4583:u32)  [unwired: 8 in]
        n1269 = case shown="True" w4587 {
          tunnel: [states."auto imaging" w4637] -> w4590
          frame False {
          }
          frame True {
            n1270 = case shown="True" "go to 4000?" {
              tunnel: [states."screening" states."4000"] -> w4637
              frame False {
              }
              frame True {
              }
            }
          }
        }
        n1271 = for {
          tunnel: w4549 -> [w4611] mode=indexing
          tunnel: [w4608] -> w4525 mode=indexing
          tunnel: [w4606] -> _ mode=indexing
          workers-P: _ -> [_]
          tunnel: [w4606] -> w4528 mode=indexing
          n1272 = local read "wave trigger"() -> (w4607:dbl)
          n1273 = Reshape Array(w4611, 4194304 ("dimension size")) -> (w4610:dbl[])
          n1274 = call-poly <vilib>:"Mean.vi"("X"=w4610) -> ("mean"=w4606:dbl)  [unwired: 1 out]
          n1275 = Greater?(x=w4606, y=w4607) -> (0:w4609:bool)
          n1276 = Boolean To (0,1)(Boolean=w4609) -> (0, 1=w4608:i16)
        }
        n1277 = case shown="False" w4566 {
          tunnel: w4565 -> [w4612 w4615]
          tunnel: [w4612 w4614] -> w4564
          frame False {
          }
          frame True {
            n1278 = local read "Last saved file number 2000"() -> (w4613:i32)
            n1279 = Replace Array Subset(array=w4615, new element=w4613, index=w4613) -> (w4614:dbl[])
          }
        }
        n1280 = flat-sequence {
          tunnel: w4584 -> [w4624]
          tunnel: w4586 -> [w4623]
          tunnel: [w4623] -> w4572
          tunnel: [w4624] -> w4571
          tunnel: [w4622] -> w4570
          tunnel: [w4632] -> w4585
          tunnel: w4572 -> [w4632]
          tunnel: w4571 -> [w4628]
          tunnel: w4570 -> [w4631]
          tunnel: w4568 -> [w4626]
          tunnel: w4518 -> [_]
          tunnel: [w4625] -> w4502
          frame #0 {
            w4616 = u8 2 items=["0", "1", "2", "3", "4"] ("Axis Number")
            w4618 = u16 4000 ("Acceleration Time")
            w4622 = "\r\n"
            n1281 = call "RS232C_SetSpeed.vi"("Low Speed"=w4618, "High Speed"=w4618, "Acceleration Time"=u16 0, "Axis Number"=w4616, "Delimiter"=w4622, "VISAリソース名"=w4623, "Axis Count"=u8 2, "Range"=TRUE, "Main/Sub"=FALSE) -> ()  [unwired: 2 out]
          }
          frame #1 {
            w4633 = u8 2 items=["0", "1", "2", "3", "4"] ("Axis Number")
            n1282 = Not(x=w4628) -> (.not. x?=w4627:bool)
            n1283 = Wait (ms)(milliseconds to wait=u32 500) -> ()  [unwired: 1 out]
            n1284 = call "RS232C_Move.vi"("VISAリソース名"=w4632, "Axis Count"=u8 2, "Axis Number"=w4633, "Pulse Number"=w4626, "Direction"=w4627, "Delimiter"=w4631, "Main/Sub"=FALSE) -> ()  [unwired: 2 out]
            n1285 = call <vilib>:"High Resolution Relative Seconds.vi"() -> ("relative seconds"=w4625:dbl)
          }
        }
        n1286 = call-poly <vilib>:"Write Waveforms to File.vi"("waveform"=w4525, "file path (dialog if empty)"=w4546) -> ()  [unwired: 8 in, 2 out]
        n1287 = Reverse 1D Array(array=w4525) -> (reversed array=w4544:i16[])
        n1288 = Search 1D Array(1D array=w4544, element=i16 1) -> (index of element=w4541:i32)  [unwired: 1 in]
        n1289 = Search 1D Array(1D array=w4525, element=i16 1) -> (index of element=w4531:i32)  [unwired: 1 in]
        n1290 = Add(x=w4531, y=w4541) -> (x+y=w4542:i32)
        n1291 = Subtract(x=200, y=w4542) -> (x-y=w4530:i32)
        n1292 = Insert Into Array(array=w4534, index=w4527, new element=w4530) -> (w4535:i16[])
        n1293 = Array Subset(array=w4528, index=w4531, length=w4530) -> (w4532:dbl[])
        n1294 = Initialize Array(0.0 ("element"), 1000 ("dimension size")) -> (w4522:dbl[])
        n1295 = call-poly <vilib>:"Mean.vi"("X"=w4532) -> ("mean"=w4529:dbl)  [unwired: 1 out]
        n1296 = Insert Into Array(array=w4522, index=w4559, new element=w4529) -> (w4558:dbl[])
        "Last saved file number 2000" <- w4506
      }
      frame "Close" {
        n1297 = call-poly <vilib>:"DAQmx Create Virtual Channel.vi"("lines"=tag "Dev1/port0/line6") -> ("task out"=w4758:refnum<k21>, "error out"=w4757:errorcluster)  [unwired: 13 in]
        n1298 = call <vilib>:"DAQmx Start Task.vi"("task/channels in"=w4758, "error in"=w4757) -> ("task out"=w4755:refnum<k21>, "error out"=w4754:errorcluster)  [unwired: 12 in]
        n1299 = call <userlib>:"tm_unpreparecapture_40.vi"("error in (no error)"=w4786, "Handle in"=w4787) -> ("error out"=w4789:errorcluster, "Handle out"=w4788:u32)  [unwired: 8 in]
        n1300 = call-poly <vilib>:"DAQmx Write.vi"("task/channels in"=w4766, "data"=FALSE) -> ()  [unwired: 11 in, 3 out]
        n1301 = call-poly <vilib>:"DAQmx Write.vi"("task/channels in"=w4764, "data"=FALSE) -> ()  [unwired: 11 in, 3 out]
        n1302 = call-poly <vilib>:"DAQmx Write.vi"("task/channels in"=w4765, "data"=FALSE) -> ()  [unwired: 11 in, 3 out]
        n1303 = local read "4C"() -> (w4720:bool)
        n1304 = local read "tb Pulses to move"() -> (w4709:u32)
        n1305 = local read "tube changing #"() -> (w4708:i32)
        n1306 = case shown="False" w4720 {
          tunnel: w4721 -> [_ w4809]
          frame False {
          }
          frame True {
            n1307 = invoke class="BenchtopStepperControl" method="CloseDevice"(reference=w4809) -> ()  [unwired: 2 in, 3 out]
          }
        }
        n1308 = call <userlib>:"tm_closecamera_40.vi"("error in (no error)"=w4789, "Handle in"=w4788) -> ("error out"=w4790:errorcluster)  [unwired: 9 in]
        n1309 = call <userlib>:"tm_deinitialize_40.vi"("error in (no error)"=w4790) -> ("error out"=→"Camera error out":errorcluster)  [unwired: 10 in]
        n1310 = Multiply(x=w4709, y=w4708) -> (x*y=w4707:u32)
        n1311 = local read "tube Direction"() -> (w4711:bool)
        n1312 = Not(x=w4711) -> (.not. x?=w4710:bool)
        n1313 = stacked-sequence {
          tunnel: w4706 -> [w4794 w4801]
          tunnel: FALSE ("Main/Sub") -> [w4795 w4808]
          tunnel: w4707 -> [_ w4805]
          tunnel: w4710 -> [_ w4804]
          tunnel: "\r\n" -> [w4793 w4802]
          tunnel: [_ w4803] -> _
          tunnel: [_ w4801] -> _
          tunnel: [_ w4802] -> _
          frame #0 {
            w4798 = u8 2 items=["0", "1", "2", "3", "4"] ("Axis Number")
            n1314 = call "RS232C_SetSpeed.vi"("Low Speed"=u32 100, "High Speed"=u32 2000, "Acceleration Time"=u16 100, "Axis Number"=w4798, "Delimiter"=w4793, "VISAリソース名"=w4794, "Axis Count"=u8 2, "Range"=TRUE, "Main/Sub"=w4795) -> ()  [unwired: 2 out]
          }
          frame #1 {
            w4806 = u8 1 items=["0", "1", "2", "3", "4"] ("Axis Number")
            n1315 = call "RS232C_Move.vi"("VISAリソース名"=w4801, "Axis Count"=u8 2, "Axis Number"=w4806, "Pulse Number"=w4805, "Direction"=w4804, "Delimiter"=w4802, "Main/Sub"=w4808) -> ("OK Done"=w4803:bool)  [unwired: 1 out]
          }
        }
        n1316 = call <vilib>:"High Resolution Relative Seconds.vi"() -> ("relative seconds"=→"experiment stop time (relative)":dbl)
        n1317 = flat-sequence {
          tunnel: refnum<visa-resource-name> "USB0::0x1AB1::0x0643::DG9A242400208::INSTR" ("VISA resource name") -> [w4814]
          tunnel: w4755 -> [w4813]
          tunnel: [w4813] -> w4752
          tunnel: w4754 -> [w4812]
          tunnel: [w4812] -> w4751
          tunnel: refnum<visa-resource-name> "USB0::0x1AB1::0x0643::DG9A242400205::INSTR" ("VISA resource name") -> [w4811]
          tunnel: [w4811] -> w4750
          tunnel: [w4810] -> w4728
          tunnel: [w4815] -> w4749
          tunnel: w4752 -> [w4819]
          tunnel: [w4819] -> w4748
          tunnel: w4751 -> [w4818]
          tunnel: [w4818] -> w4747
          tunnel: w4750 -> [w4817]
          tunnel: [w4817] -> w4746
          tunnel: w4728 -> [w4816]
          tunnel: w4749 -> [w4828]
          tunnel: [w4822] -> w4745
          tunnel: w4748 -> [w4825]
          tunnel: [w4825] -> w4744
          tunnel: w4747 -> [w4824]
          tunnel: [w4824] -> w4743
          tunnel: w4746 -> [w4823]
          tunnel: [w4823] -> w4742
          tunnel: w4745 -> [w4832]
          tunnel: [w4832] -> w4741
          tunnel: w4744 -> [w4831]
          tunnel: [w4831] -> w4740
          tunnel: w4743 -> [w4830]
          tunnel: [w4830] -> w4739
          tunnel: w4742 -> [w4834]
          tunnel: [w4829] -> w4738
          tunnel: w4741 -> [w4838]
          tunnel: [w4838] -> w4737
          tunnel: w4740 -> [w4837]
          tunnel: [w4837] -> w4736
          tunnel: w4739 -> [w4836]
          tunnel: [w4836] -> w4735
          tunnel: w4738 -> [w4840]
          tunnel: [w4835] -> w4734
          tunnel: w4737 -> [w4847]
          tunnel: [w4847] -> w4733
          tunnel: w4736 -> [w4846]
          tunnel: [w4846] -> w4732
          tunnel: w4735 -> [w4845]
          tunnel: [w4845] -> w4731
          tunnel: w4734 -> [w4848]
          tunnel: [w4843] -> w4727
          tunnel: w4733 -> [w4853]
          tunnel: w4732 -> [w4851]
          tunnel: [w4851] -> w4730
          tunnel: w4731 -> [w4850]
          tunnel: [w4850] -> w4729
          tunnel: w4727 -> [w4849]
          tunnel: w4730 -> [w4859]
          tunnel: w4729 -> [w4858]
          frame #0 {
            # "CONNECT"
            n1318 = VISA Open(VISA resource name=w4814) -> (VISA resource name=w4810:refnum<visa-resource-name>)  [unwired: 4 in, 1 out]
          }
          frame #1 {
            n1319 = Wait (ms)(milliseconds to wait=u32 500) -> ()  [unwired: 1 out]
            n1320 = VISA Write(VISA resource name=w4816, write buffer=":OUTP2 OFF") -> (VISA resource name out=w4815:refnum<visa-resource-name>)  [unwired: 1 in, 2 out]
          }
          frame #2 {
            n1321 = VISA Write(VISA resource name=w4828, write buffer=":OUTP1 OFF") -> (VISA resource name out=w4822:refnum<visa-resource-name>)  [unwired: 1 in, 2 out]
            n1322 = Wait (ms)(milliseconds to wait=u32 500) -> ()  [unwired: 1 out]
          }
          frame #3 {
            n1323 = VISA Open(VISA resource name=w4834) -> (VISA resource name=w4829:refnum<visa-resource-name>)  [unwired: 4 in, 1 out]
            n1324 = Wait (ms)(milliseconds to wait=u32 500) -> ()  [unwired: 1 out]
          }
          frame #4 {
            n1325 = VISA Write(VISA resource name=w4840, write buffer=":OUTP2 OFF") -> (VISA resource name out=w4835:refnum<visa-resource-name>)  [unwired: 1 in, 2 out]
            n1326 = Wait (ms)(milliseconds to wait=u32 500) -> ()  [unwired: 1 out]
          }
          frame #5 {
            n1327 = Wait (ms)(milliseconds to wait=u32 500) -> ()  [unwired: 1 out]
            n1328 = VISA Write(VISA resource name=w4848, write buffer=":OUTP1 OFF") -> (VISA resource name out=w4843:refnum<visa-resource-name>)  [unwired: 1 in, 2 out]
          }
          frame #6 {
            n1329 = VISA Clear(VISA resource name=w4853) -> ()  [unwired: 1 in, 2 out]
            n1330 = VISA Clear(VISA resource name=w4849) -> ()  [unwired: 1 in, 2 out]
            n1331 = Wait (ms)(milliseconds to wait=u32 500) -> ()  [unwired: 1 out]
          }
          frame #7 {
            n1332 = call-poly <vilib>:"DAQmx Write.vi"("task/channels in"=w4859, "data"=TRUE, "error in"=w4858) -> ("task out"=w4855:refnum<k21>, "error out"=w4854:errorcluster)  [unwired: 10 in, 1 out]
            n1333 = call <vilib>:"DAQmx Stop Task.vi"("task/channels in"=w4855, "error in"=w4854) -> ("task out"=w4857:refnum<k21>, "error out"=w4856:errorcluster)  [unwired: 12 in]
            n1334 = call <vilib>:"DAQmx Clear Task.vi"("task in"=w4857, "error in"=w4856) -> ()  [unwired: 13 in, 1 out]
          }
        }
      }
      frame "Stop" {
        w4905 = FALSE
        n1335 = invoke class="VI" method="Abort VI"(reference=w4863) -> ()  [unwired: 2 in, 3 out]
        n1336 = call-poly <vilib>:"DAQmx Write.vi"("task/channels in"=w4907, "data"=w4905, "error in"=w4895) -> ("task out"=w4897:refnum<k21>, "error out"=w4894:errorcluster)  [unwired: 10 in, 1 out]
        n1337 = call-poly <vilib>:"DAQmx Write.vi"("task/channels in"=w4906, "data"=w4905, "error in"=w4892) -> ("task out"=w4896:refnum<k21>, "error out"=w4891:errorcluster)  [unwired: 10 in, 1 out]
        n1338 = call-poly <vilib>:"DAQmx Write.vi"("task/channels in"=w4909, "data"=w4905, "error in"=w4908) -> ("task out"=w4898:refnum<k21>, "error out"=w4893:errorcluster)  [unwired: 10 in, 1 out]
        n1339 = call <vilib>:"DAQmx Stop Task.vi"("task/channels in"=w4897, "error in"=w4894) -> ("task out"=w4904:refnum<k21>, "error out"=w4903:errorcluster)  [unwired: 12 in]
        n1340 = call <vilib>:"DAQmx Stop Task.vi"("task/channels in"=w4896, "error in"=w4891) -> ("task out"=w4900:refnum<k21>, "error out"=w4899:errorcluster)  [unwired: 12 in]
        n1341 = call <vilib>:"DAQmx Stop Task.vi"("task/channels in"=w4898, "error in"=w4893) -> ("task out"=w4902:refnum<k21>, "error out"=w4901:errorcluster)  [unwired: 12 in]
        n1342 = call <vilib>:"DAQmx Clear Task.vi"("task in"=w4904, "error in"=w4903) -> ()  [unwired: 13 in, 1 out]
        n1343 = call <vilib>:"DAQmx Clear Task.vi"("task in"=w4900, "error in"=w4899) -> ()  [unwired: 13 in, 1 out]
        n1344 = call <vilib>:"DAQmx Clear Task.vi"("task in"=w4902, "error in"=w4901) -> ()  [unwired: 13 in, 1 out]
        n1345 = local read "experiment stop time (relative)"() -> (w4874:dbl)
        n1346 = local read "experiment start time (relative)"() -> (w4873:dbl)
        n1347 = Subtract(x=w4874, y=w4873) -> (x-y=w4872:dbl)
        n1348 = Divide(x=w4872, y=60.0) -> (x/y=w4868:dbl)
        "experiment time(mins)" <- w4868
        n1349 = Greater?(x=w4868, y=5.0) -> (0:w4870:bool)
        n1350 = case shown="True" w4870 {
          tunnel: w4867 -> [_ w4955]
          tunnel: w4866 -> [_ w4951]
          frame False {
          }
          frame True {
            w4935 = "15528131356@163.com" ("username")
            w4948 = "\\" ("string")
            # "email system"
            n1351 = local read "Save directory"() -> (w4953:path)
            n1352 = local read "Last saved #"() -> (w4971:i32)
            n1353 = Increment(x=w4971) -> (x+1=w4962:i32)
            n1354 = local read "experiment time(mins)"() -> (w4963:dbl)
            n1355 = Path To String(path=w4953) -> (string=w4952:string)
            n1356 = Number To Decimal String(number=w4962) -> (decimal integer string=w4970:string)  [unwired: 1 in]
            n1357 = Divide(x=w4962, y=w4963) -> (x/y=w4961:dbl)
            n1358 = Number To Decimal String(number=w4963, width (-)=i16 4) -> (decimal integer string=w4973:string)
            n1359 = Number To Decimal String(number=w4961) -> (decimal integer string=w4960:string)  [unwired: 1 in]
            n1360 = case shown="\"chenglang\"" "Operator" {
              tunnel: [string[] ["ktsubasa@g.ecc.u-tokyo.ac.jp"] ("to") string[] ["hu-chenglang@g.ecc.u-tokyo.ac.jp"] ("to") string[] ["gabrielwangld@gmail.com"] ("cc")] -> w4928
              frame "kobayashi" {
              }
              frame "chenglang" {
              }
              frame "hanqing WANG", Default {
              }
            }
            n1361 = Concatenate Strings("Experiment time:" ("string"), w4973, w4948, "Sample number:" ("string"), w4970, "/Throughput:" ("string"), w4960, "" ("string"), "real laser power:" ("string"), w4951, "sample name:" ("string"), w4955, "saving directory:" ("string"), w4952, "clearing date:" ("string"), "clearing date", w4948) -> (w4936:string)
            n1362 = Get Date/Time String() -> (date string=w4968:string, time string=w4965:string)  [unwired: 3 in]
            n1363 = Concatenate Strings("smtp.163.com" ("string"), ":" ("string"), "25" ("string")) -> (w4931:string)
            n1364 = call <vilib>:"Open Handle.vi"("server address"=w4931, "from"=w4935, "username"=w4935, "password"="element1010") -> ("handle out"=w4947:T12, "error out"=w4946:errorcluster)  [unwired: 10 in]
            n1365 = call <vilib>:"Set Recipients.vi"("handle in"=w4947, "to"=w4928, "cc"=string[] ["pteamcalendar@gmail.com"], "error in (no error)"=w4946) -> ("handle out"=w4945:T12, "error out"=w4944:errorcluster)  [unwired: 10 in]
            n1366 = Concatenate Strings("Experiment record_" ("Subject"), w4968, "_" ("string"), w4965) -> (w4937:string)
            n1367 = call-poly <vilib>:"Set Message.vi"("handle in"=w4945, "subject"=w4937, "plain text message"=w4936, "error in (no error)"=w4944) -> ("handle out"=w4943:T12, "error out"=w4942:errorcluster)  [unwired: 10 in]
            n1368 = call <vilib>:"Set Attachments.vi"("handle in"=w4943, "error in (no error)"=w4942) -> ("handle out"=w4941:T12, "error out"=w4940:errorcluster)  [unwired: 12 in]
            n1369 = call <vilib>:"Send.vi"("handle in"=w4941, "error in (no error)"=w4940) -> ("handle out"=w4939:T12, "error out"=w4938:errorcluster)  [unwired: 11 in, 1 out]
            n1370 = call <vilib>:"Close Handle.vi"("handle in"=w4939, "error in (no error)"=w4938) -> ()  [unwired: 12 in, 2 out]
          }
        }
      }
    }
    "Larvae until move" <- w156
    "at imaging time" <- w129
    "tube changing #" <- w119
    n1371 = Format Into String(w211) -> (resulting string=→"Current state":string)  [unwired: 3 in, 1 out]
    "4c label #" <- w99
  }
  n1372 = flat-sequence {
    tunnel: w66 -> [w4984]
    tunnel: w50 -> [_]
    tunnel: w49 -> [_]
    tunnel: w48 -> [_]
    tunnel: w45 -> [_]
    tunnel: w41 -> [_]
    tunnel: w34 -> [_]
    tunnel: w33 -> [w4982]
    tunnel: w32 -> [w4981]
    tunnel: w15 -> [w4978]
    frame #0 {
      n1373 = call <vilib>:"DAQmx Stop Task.vi"("task/channels in"=w4982, "error in"=w4981) -> ("task out"=w4980:refnum<k21>, "error out"=w4979:errorcluster)  [unwired: 12 in]
      n1374 = VISA Clear(VISA resource name=w4978) -> ()  [unwired: 1 in, 2 out]
      n1375 = call <vilib>:"DAQmx Clear Task.vi"("task in"=w4980, "error in"=w4979) -> ()  [unwired: 13 in, 1 out]
      n1376 = Index Array(array=w4984, index=1500) -> (element=w4985:T9)
      n1377 = call "IMAQ Dispose"("All Images? (No)"=TRUE, "Image"=w4985) -> ()  [unwired: 4 in, 1 out]
    }
  }
